vi "main_scan_2.vi"() -> ()   [LabVIEW 2009]
uses:
  <vilib>/userDefined/High Color/IMAQdx.ctl
  <vilib>/vision/Image Controls.llb/IMAQ Image.ctl
  global_stage_initialised.vi
  <vilib>/vision/driver/IMAQdx.llb/IMAQdx Buffer Number Mode.ctl
  <vilib>/Utility/file.llb/Write To Spreadsheet File (DBL).vi
  <vilib>/vision/driver/NI_Vision_Acquisition_Software.lvlib
  C:/Program Files/National Instruments/LabVIEW 2009/resource/objmgr/imaqdx.rc
panel:
  in  "Max. Spannungsdifferenz":dbl=150.0
  out "Geschätzte Messzeit":string="00:00"
  out "Start time [ms]":timestamp
  out "2D-Intensitätsverteilung (MCP)":dbl[][](graph)
  in  "# Photosignale":i32
  in  "Achs-ID":i32
  in  "Spannungskanal":refnum<k21>
  out "x-U-Scan läuft":bool
  out "Spannungsscan läuft":bool
  out "LAPD Spannung (V)":dbl format="%#.3g"
  out "Summierte Helligkeit (a.u.)":u64
  out "# Messschritte":i32
  out "Aktueller Messschritt":i32
  in  "LAPD-Daten speichern":bool
  in  "Summierte Helligkeit speichern":bool
  in  "Einzelbilder speichern":bool
  in  "Gemittelte Bilder speichern":bool
  in  "# Bilder/Messschritt":i32=1
  in  "SN von Rotationsbühne":i32=83831982
  in  "Wellenplatte [°]":refnum<k7>(container)
  out "Wellenplatte":bool
  in  "Waveplate ON/OFF":bool
  in  "Registerkarte":T1(tab)=enum."x-U-Scan"
  out "Aktuelle xyz-Position [mm]":dbl[](array[numeric]) format="%.5g"
  in  "Rasterweite [µm]":dbl[](array[numeric])
  in  "# Rasterschritte":i32[](array[numeric])=[1, 1, 1] min=1 step=1
  in  "Rasterung ON/OFF":bool
  out "Start xyz-Position [mm]":dbl[](array[numeric]) format="%.5g"
  in  "Rasterart":T2(ring)=enum."2D-Scan(xy)"
  out "Rasterschritt [µm]":dbl[](array[numeric])
  out "2D-Intensitätsverteilung (LAPD)":dbl[][](graph)
  out "Spannungsstart [V]":dbl[](array[numeric])
  out "TIP/SUP":string[](array[string])=["Tip", "Suppressor"]
  out "Spannungsschritt [V]":dbl[](array[numeric]) format="%.1g"
  out "Aktuelle Spannung [V]":dbl[](array[numeric]) format="%.1f"
  in  "# Spannungsschritte":i32[](array[numeric])
  in  "Spannungsweite [V]":dbl[](array[numeric])
  in  "Spannungsscan ON/OFF":bool
  out "Schräglage berücksichtigen":string="Schräglage berücksichtigen"
  in  "Ausgleichslage Start festlegen":bool
  out "x-U-Scan (Ausgleichslage) xy-Start [mm]":dbl[](array[numeric]) format="%_5g"
  in  "Raum-Koordinate 2 (Lagenausgleich)":enum16{"x-Achse", "y-Achse", "z-Achse"}(ring)=enum."y-Achse"
  out "x-U-Scan y-Startposition [mm]":dbl format="%.4g"
  out "x-U-Scan aktuelle y-Position [mm]":dbl format="%.4g"
  in  "x-U-Scan (Ausgleichslage) Steigung":dbl format="%_3g"
  out "x-U-Scan Spannungsstart [V]":dbl
  out "x-U-Scan Spannungsschritt [V]":dbl
  out "x-U-Scan aktuelle Spannung [V]":dbl
  in  "# x-U-Scan Spannungsschritte":i32
  in  "x-U-Scan Spannungsweite [V]":dbl
  in  "Raum-Koordinate 1":enum16{"x-Achse", "y-Achse", "z-Achse"}(ring)
  in  "Spannungs-Koordinate":enum16{"Tip-Spannung", "Suppressor-Spannung"}(ring)=2
  in  "x-U-Scan ON/OFF":bool
  in  "x-U-Scan x-Rasterweite [µm]":dbl
  in  "# x-U-Scan x-Rasterschritte":i32
  out "x-U-Scan x-Startposition [mm]":dbl format="%.4g"
  out "x-U-Scan aktuelle x-Position [mm]":dbl format="%.4g"
  out "x-U-Scan x-Rasterschritt [µm]":dbl
  out "x-U-Scan (Ausgleichslage) xy-End [mm]":dbl[](array[numeric]) format="%_5g"
  in  "Ausgleichslage Ende festlegen":bool
  in  "Sequenz Ordner":string="Referenzbilder"
  in  "Sequenzaufnahme ON":bool
  in  "MCP-Spannung [V]":dbl=1400.0
  in  "P-Schirm-Spannung [V]":dbl=4400.0
  in  "Proben-ID":string="140528_06"
  out "Messlogbuch":path
  out "Gemitteltes Bild":u64[][](array[numeric])
  in  "Polarisation [°]":dbl=90.0
  out "Current y step":i32
  out "Current z step":i32
  out "Current x step":i32
  out "Scanschleifenzähler":i32
  out "Kameraschleifenzähler":i32
  out "Steuerschleifenzähler":i32
  out "Bühne":bool
  in  "HV ON/OFF":bool
  out "HV-Steuerung":bool
  in  "Suppressor-Spannung [V]":dbl min=0.0 max=1000.0 step=1.0 format="%.1p"
  in  "Tip-Spannung [V]":dbl min=0.0 max=800.0 step=1.0 format="%.1p"
  in  "Leistung (iK) [mW]":dbl format="%.1g"
  in  "LAPD-Kanal (Meilhaus)":u32=1 max=31
  out "Save folder":string
  out "Buffer Number":u64
  out "ROI table":string[](array[string])=["Breite [px]", "Höhe [px]", "X-Offset [px]", "Y-Offset [px]"]
  in  "Vollbild":bool
  out "Frame Rate (FPS)":dbl format="%#_3g"
  in  "Buffer Interval":u32=1
  out "Ereignis: FrameDone?":refnum<event-registration>
  out "Image Display":T3(plugin-control)
  in  "ROI":i32[](array[numeric])=[640, 480, 0, 0]
  in  "Shutter time (ms)":u16(ring)=3 items=["1000", "500", "200", "100", "50", "20", "10"]
  out "Buffer Overrun":bool
  out "Image Memory":T3
  out "Kamera":bool
  in  "Kamera ON/OFF":bool
  in  "Detektionskamera":T4="cam0"
  out "Day folder":string
  in  "Root folder":string="E:\\GIPES\\Messungen\\"
  out "z-Achse":i32=3
  out "y-Achse":i32=2
  out "x-Achse":i32=1
  out "Event: Rasterung gestartet?":refnum<user-event>
  out "Fehler (Ausgang)":errorcluster
  in  "Programm beenden":bool
  out "Rasterung läuft":bool
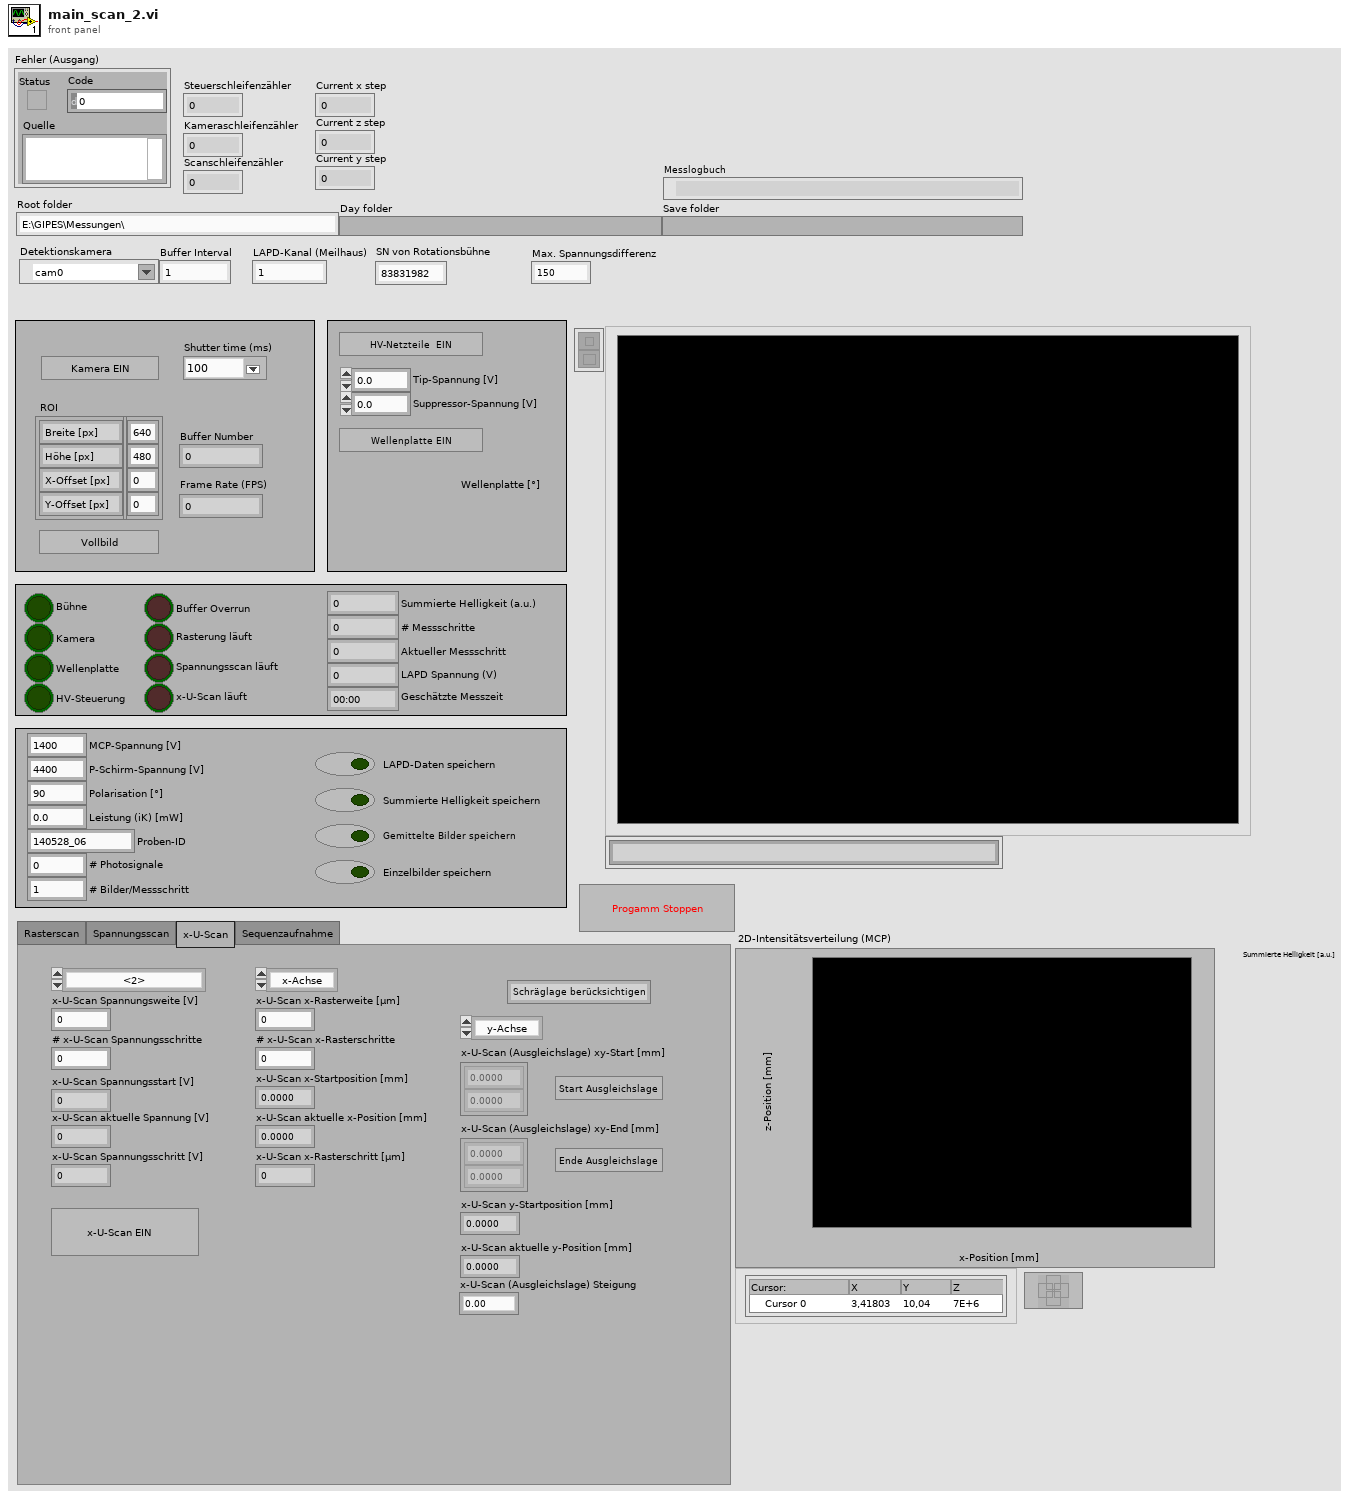
[diagram p1: front panel]
types:
  T1 = enum32{"Rasterscan", "Spannungsscan", "x-U-Scan", "Sequenzaufnahme"}
  T2 = enum16{"Linescan(x)", "Linescan(z)", "2D-Scan(xy)", "2D-Scan(yz)", "2D-Scan(xz)"}
  T3 = typedef "IMAQ Image.ctl" = refnum<image>
  T4 = typedef "IMAQdx.ctl" = refnum<k21>
  T5 = enum32{"Bad", "Idle", "Run top level", "Running"}
  T6 = typedef "NI_Vision_Acquisition_Software.lvlib/IMAQdx Buffer Number Mode.ctl" = enum32{"Next", "Last", "Buffer Number"}
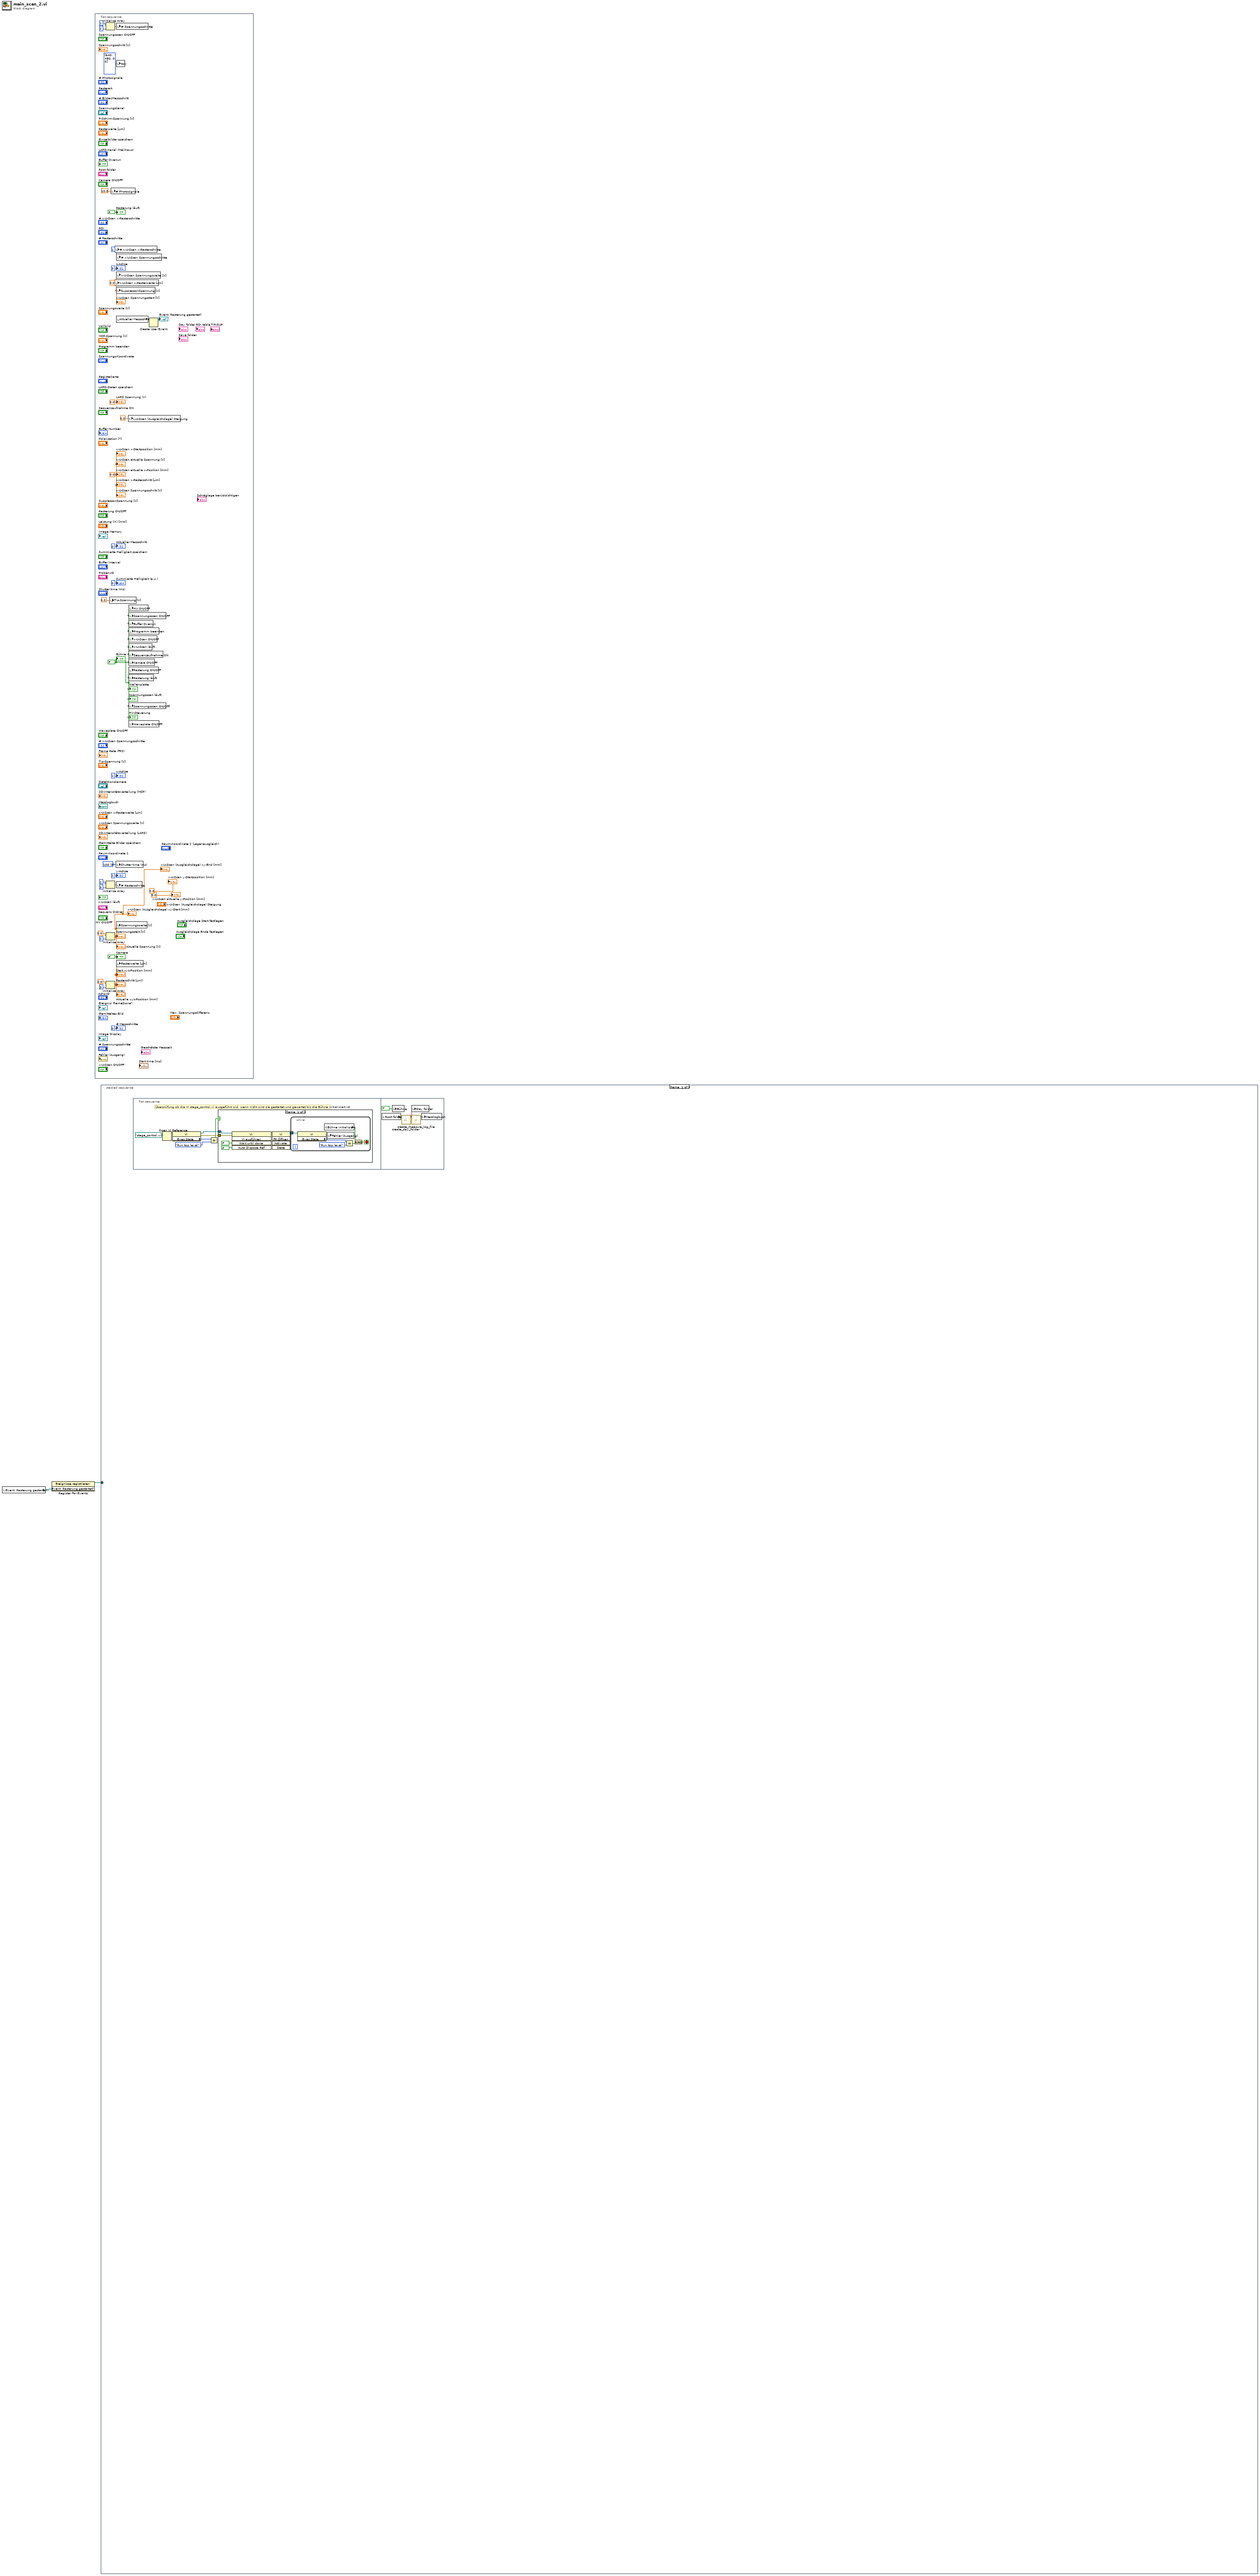
[diagram p0: block diagram]
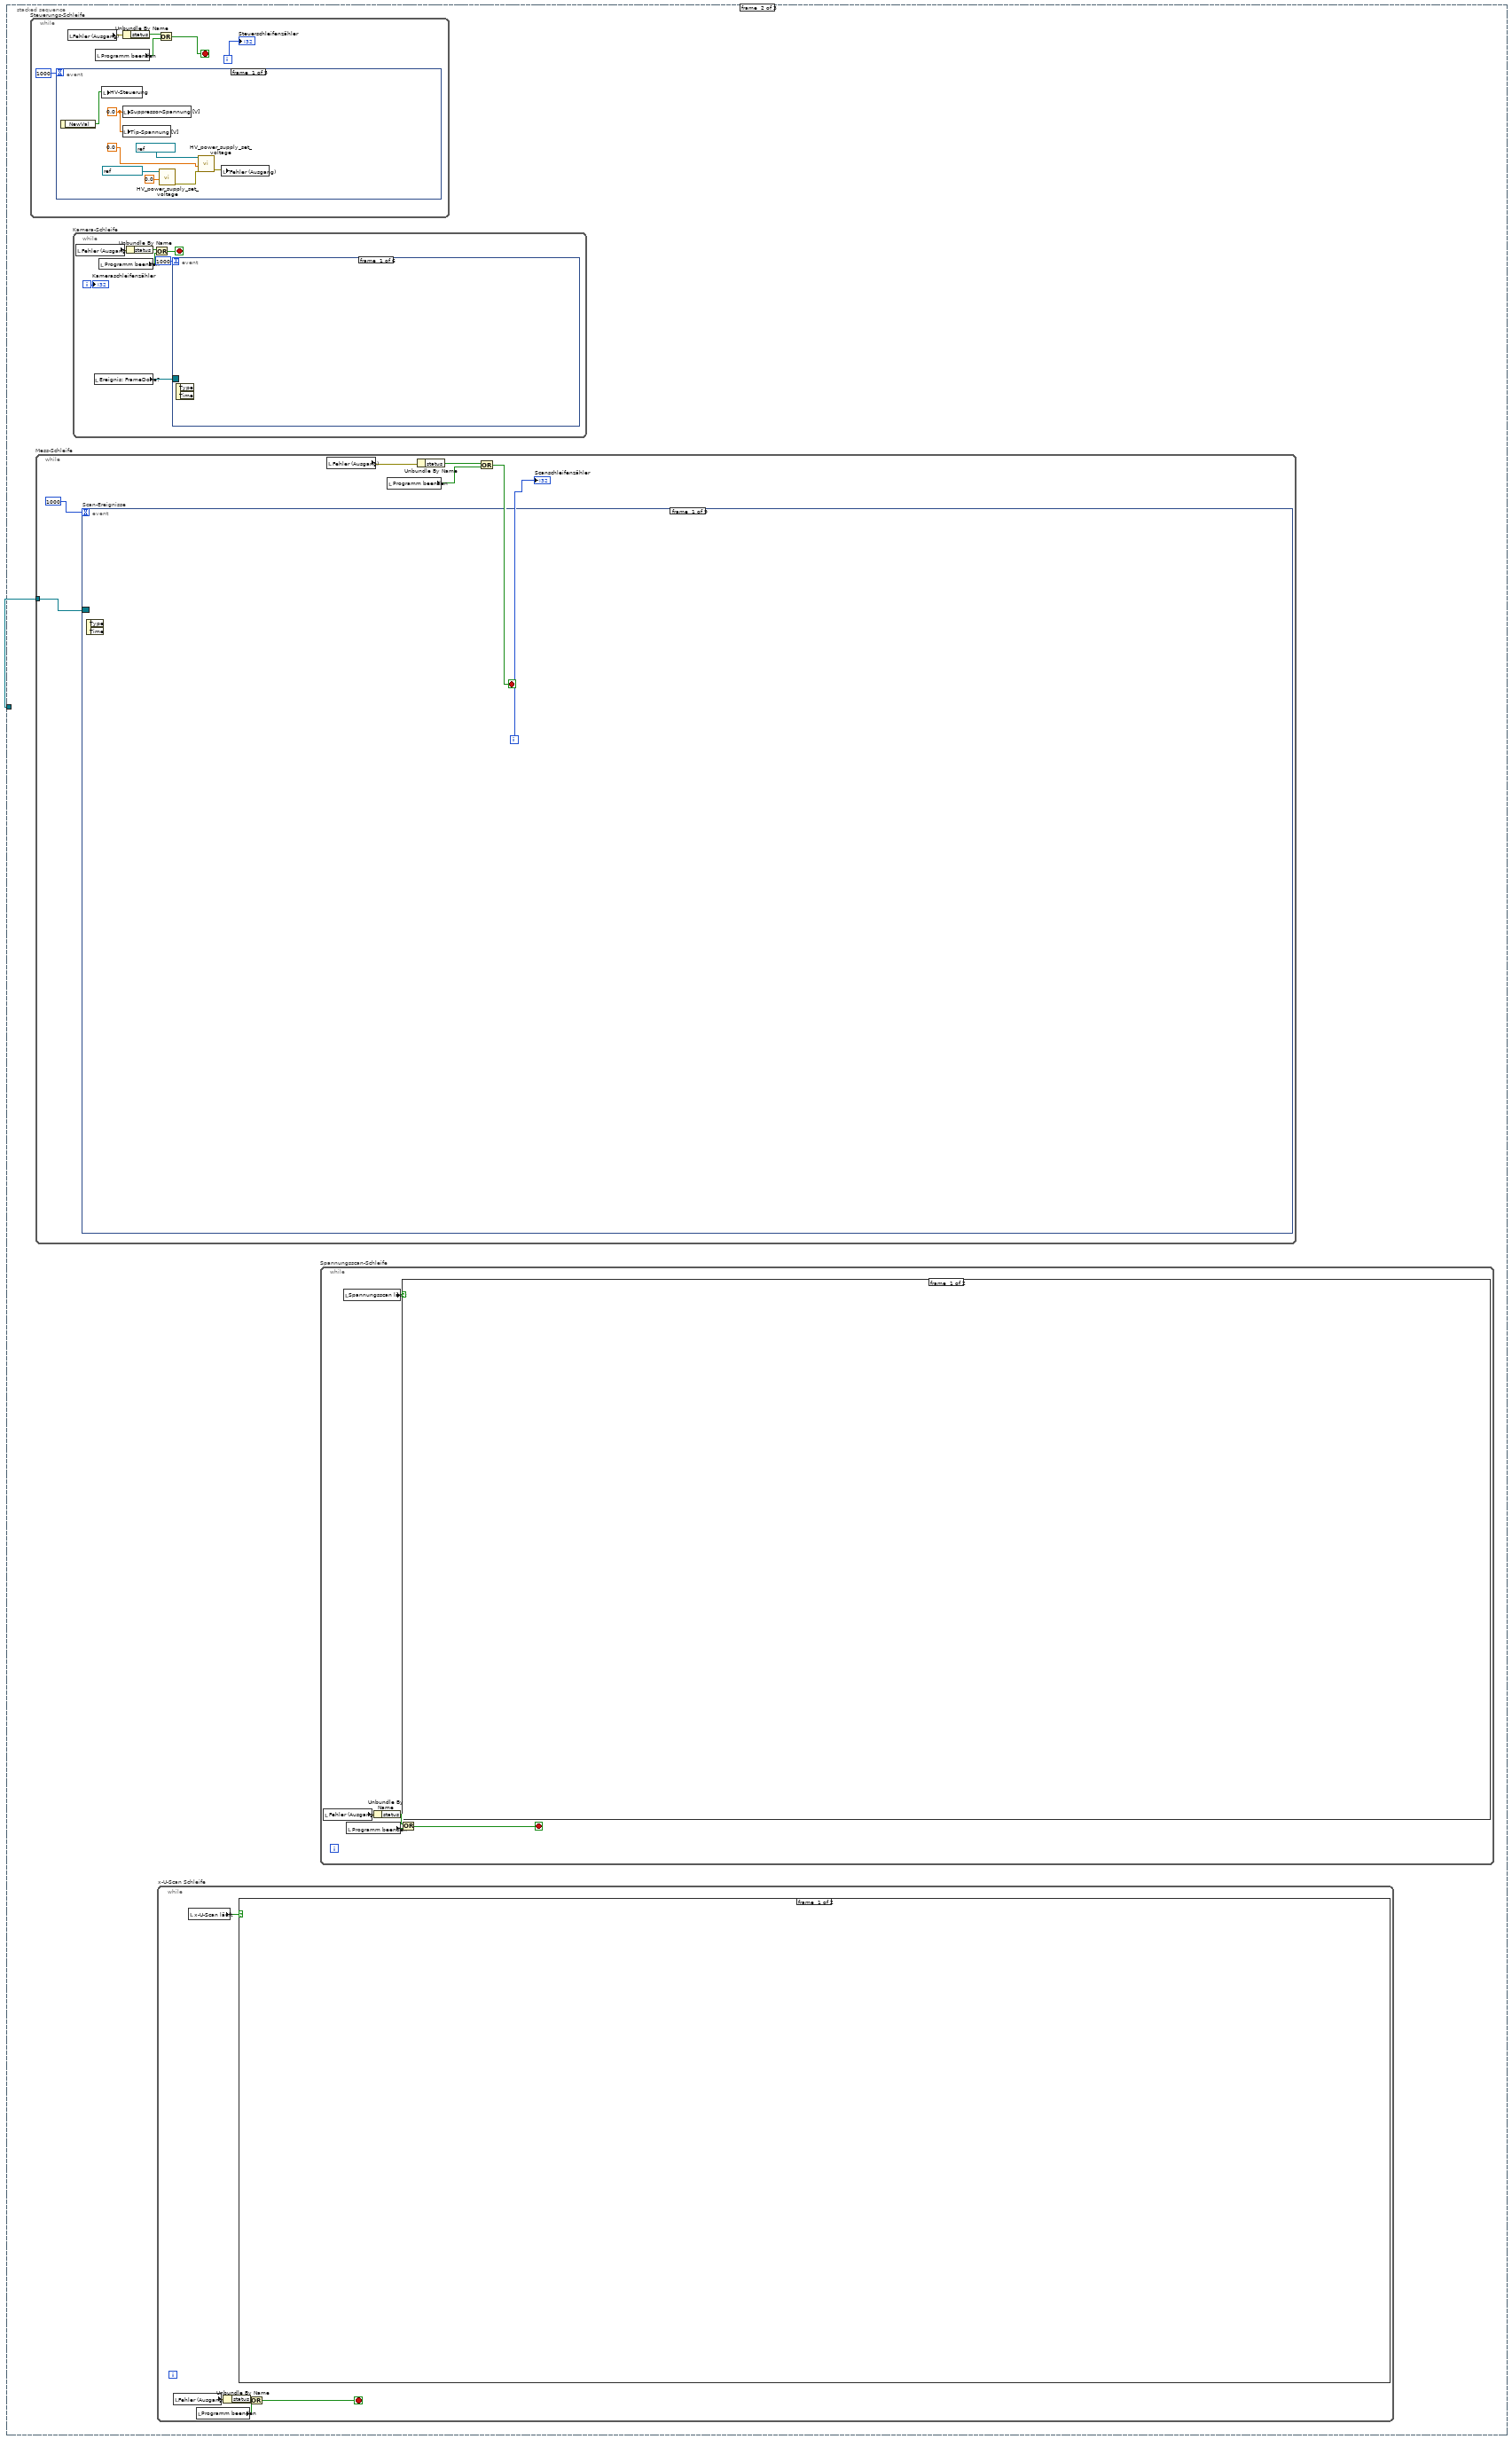
[diagram p3: hidden frame]
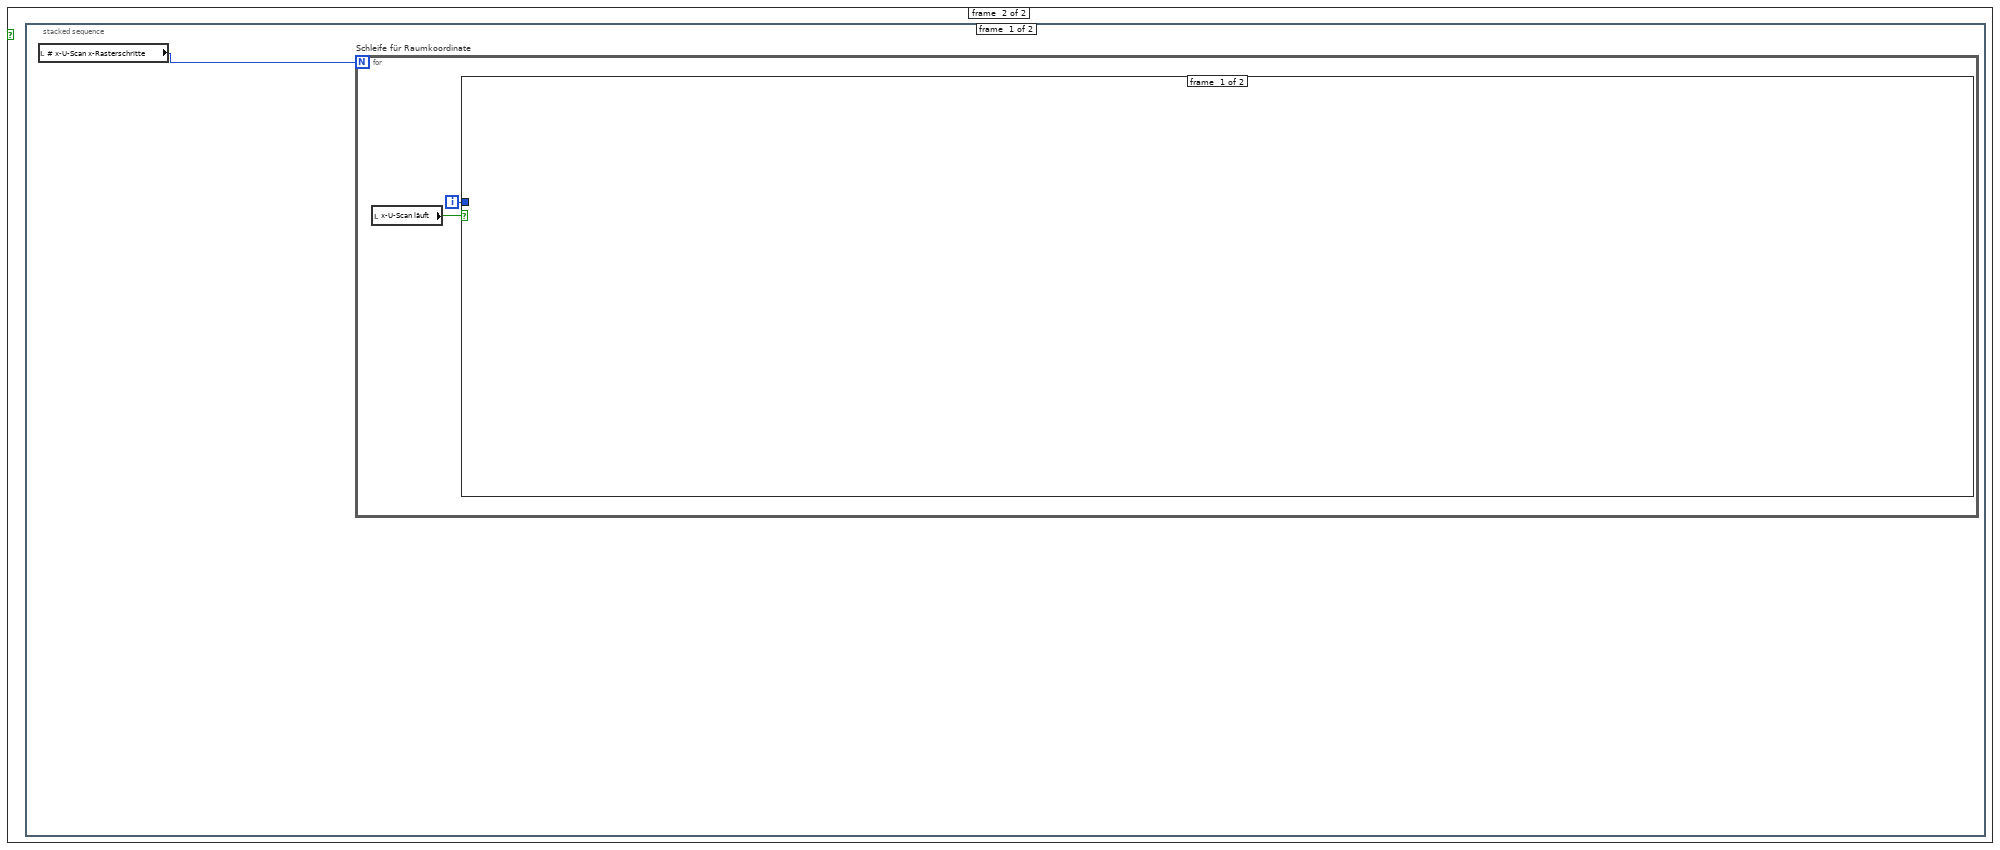
[diagram p4: hidden frame]
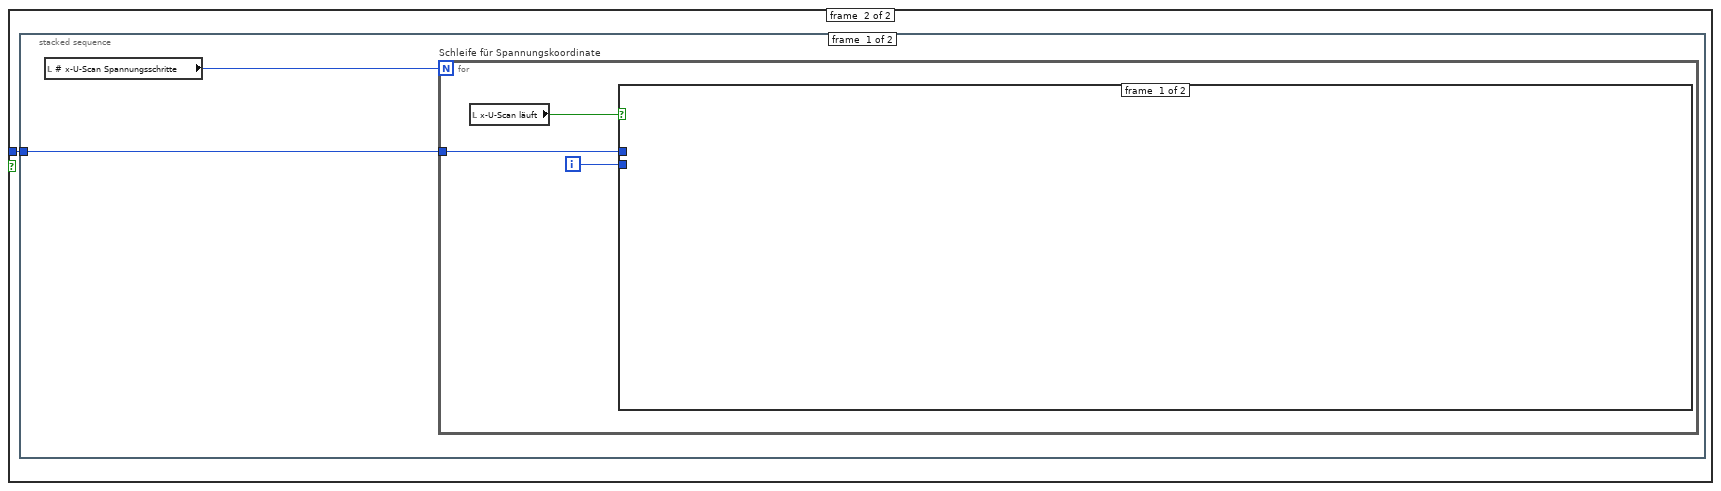
[diagram p5: hidden frame]
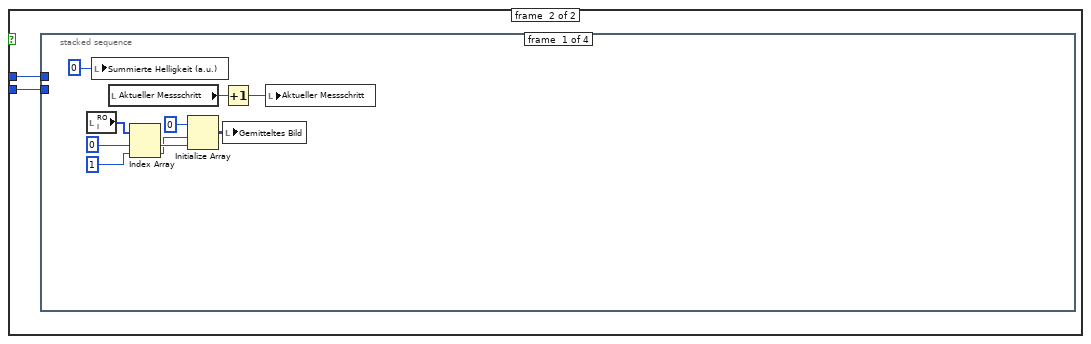
[diagram p6: hidden frame]
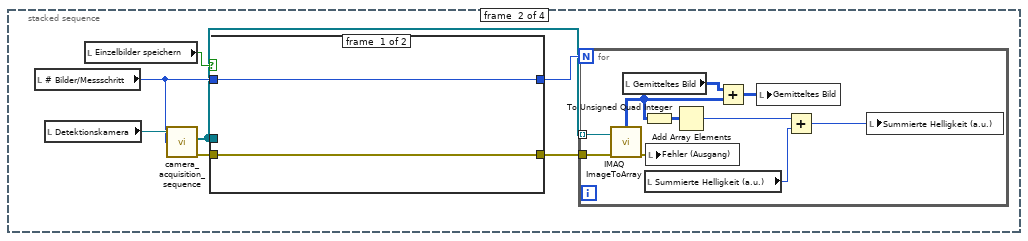
[diagram p7: hidden frame]
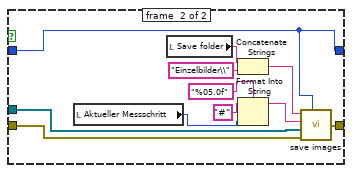
[diagram p8: hidden frame]
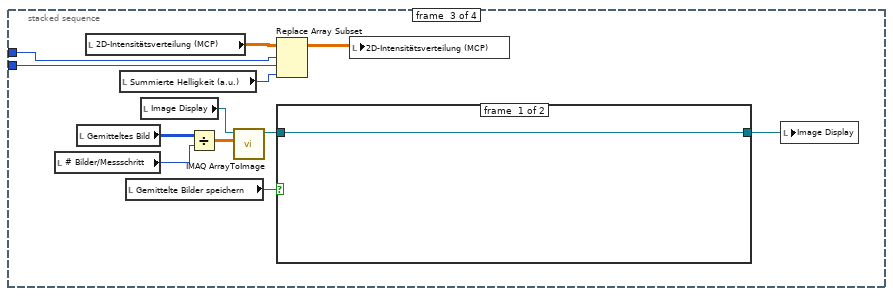
[diagram p9: hidden frame]
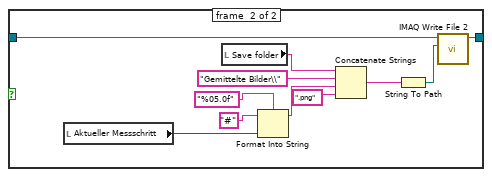
[diagram p10: hidden frame]
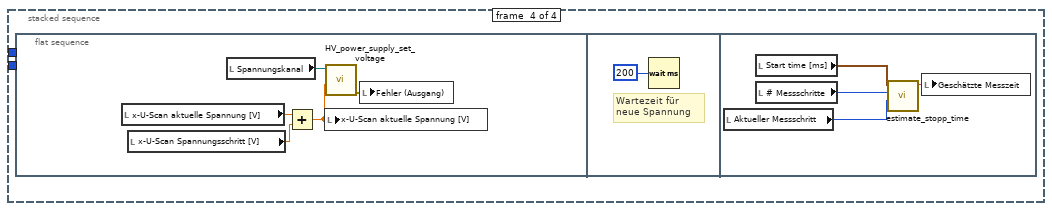
[diagram p11: hidden frame]
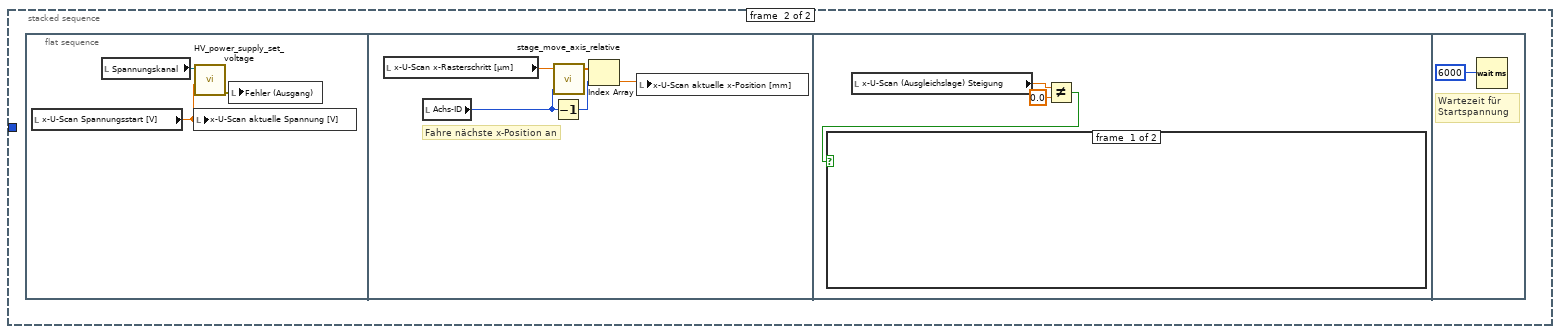
[diagram p12: hidden frame]
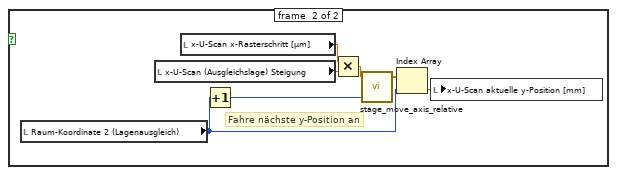
[diagram p13: hidden frame]
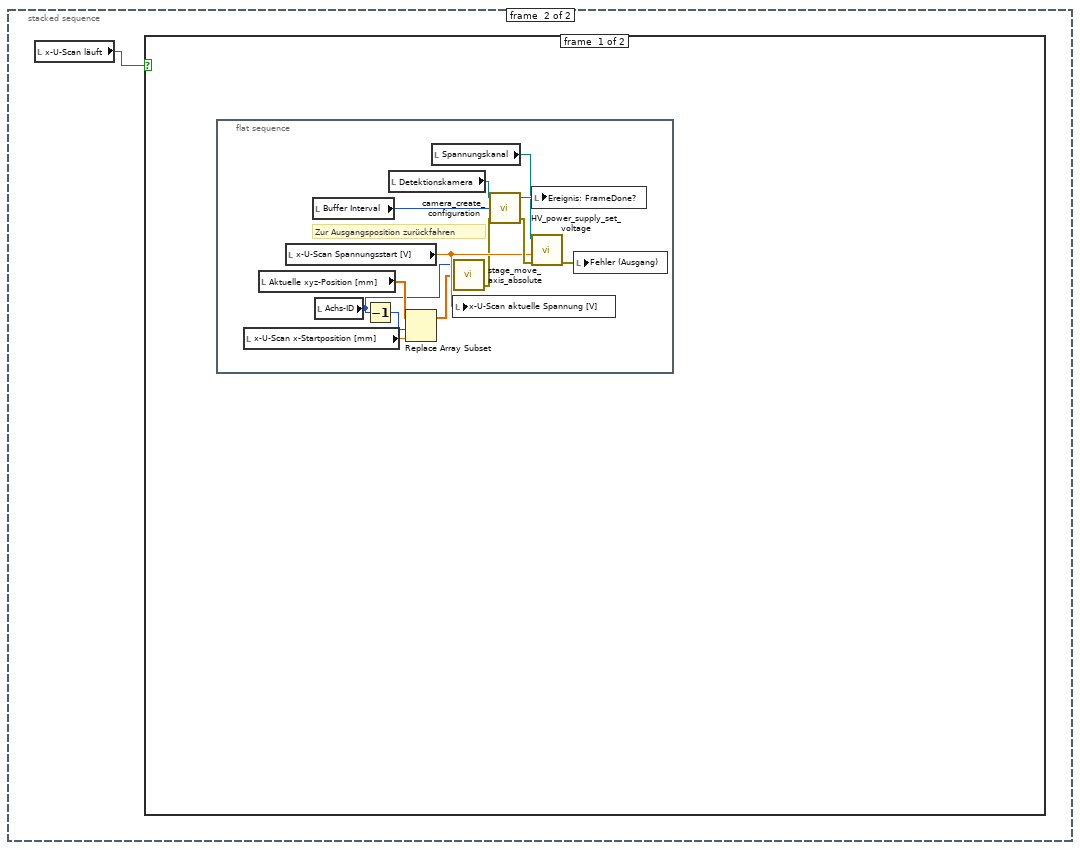
[diagram p14: hidden frame]
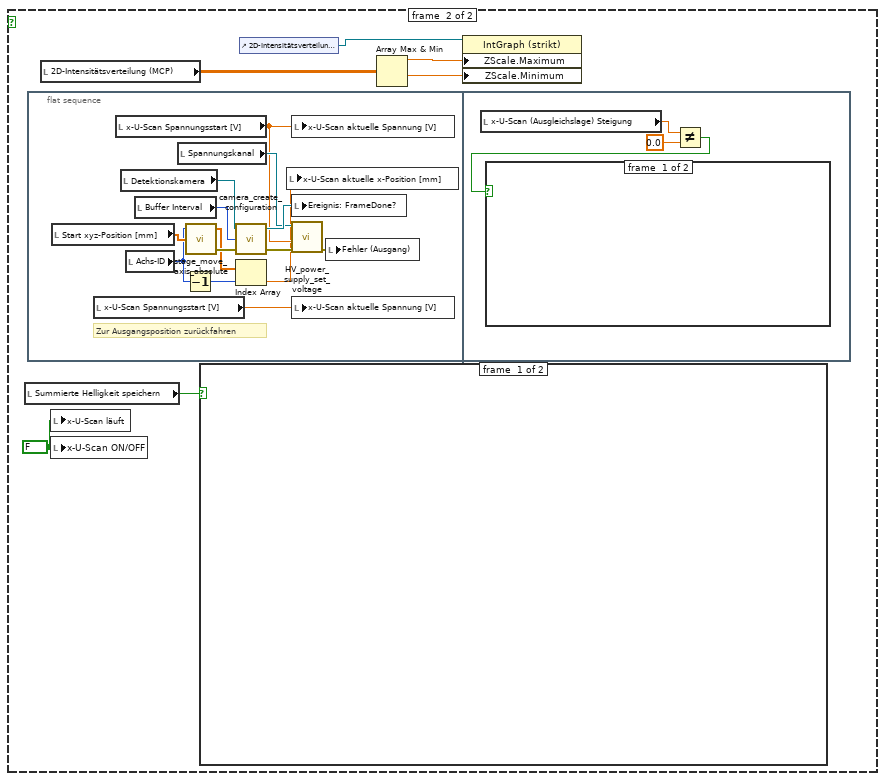
[diagram p15: hidden frame]
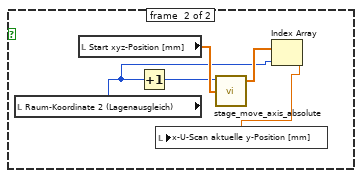
[diagram p16: hidden frame]
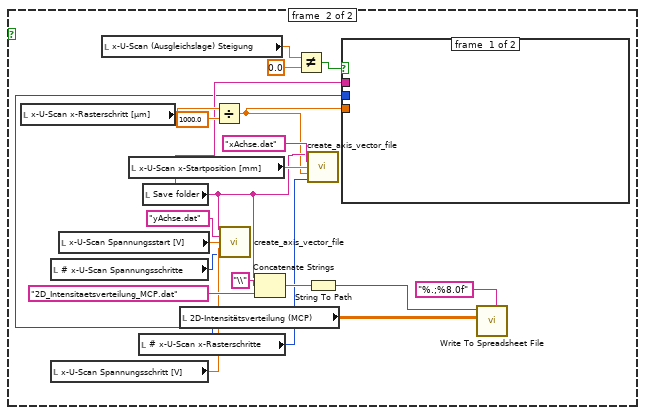
[diagram p17: hidden frame]
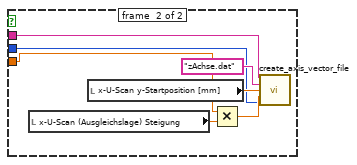
[diagram p18: hidden frame]
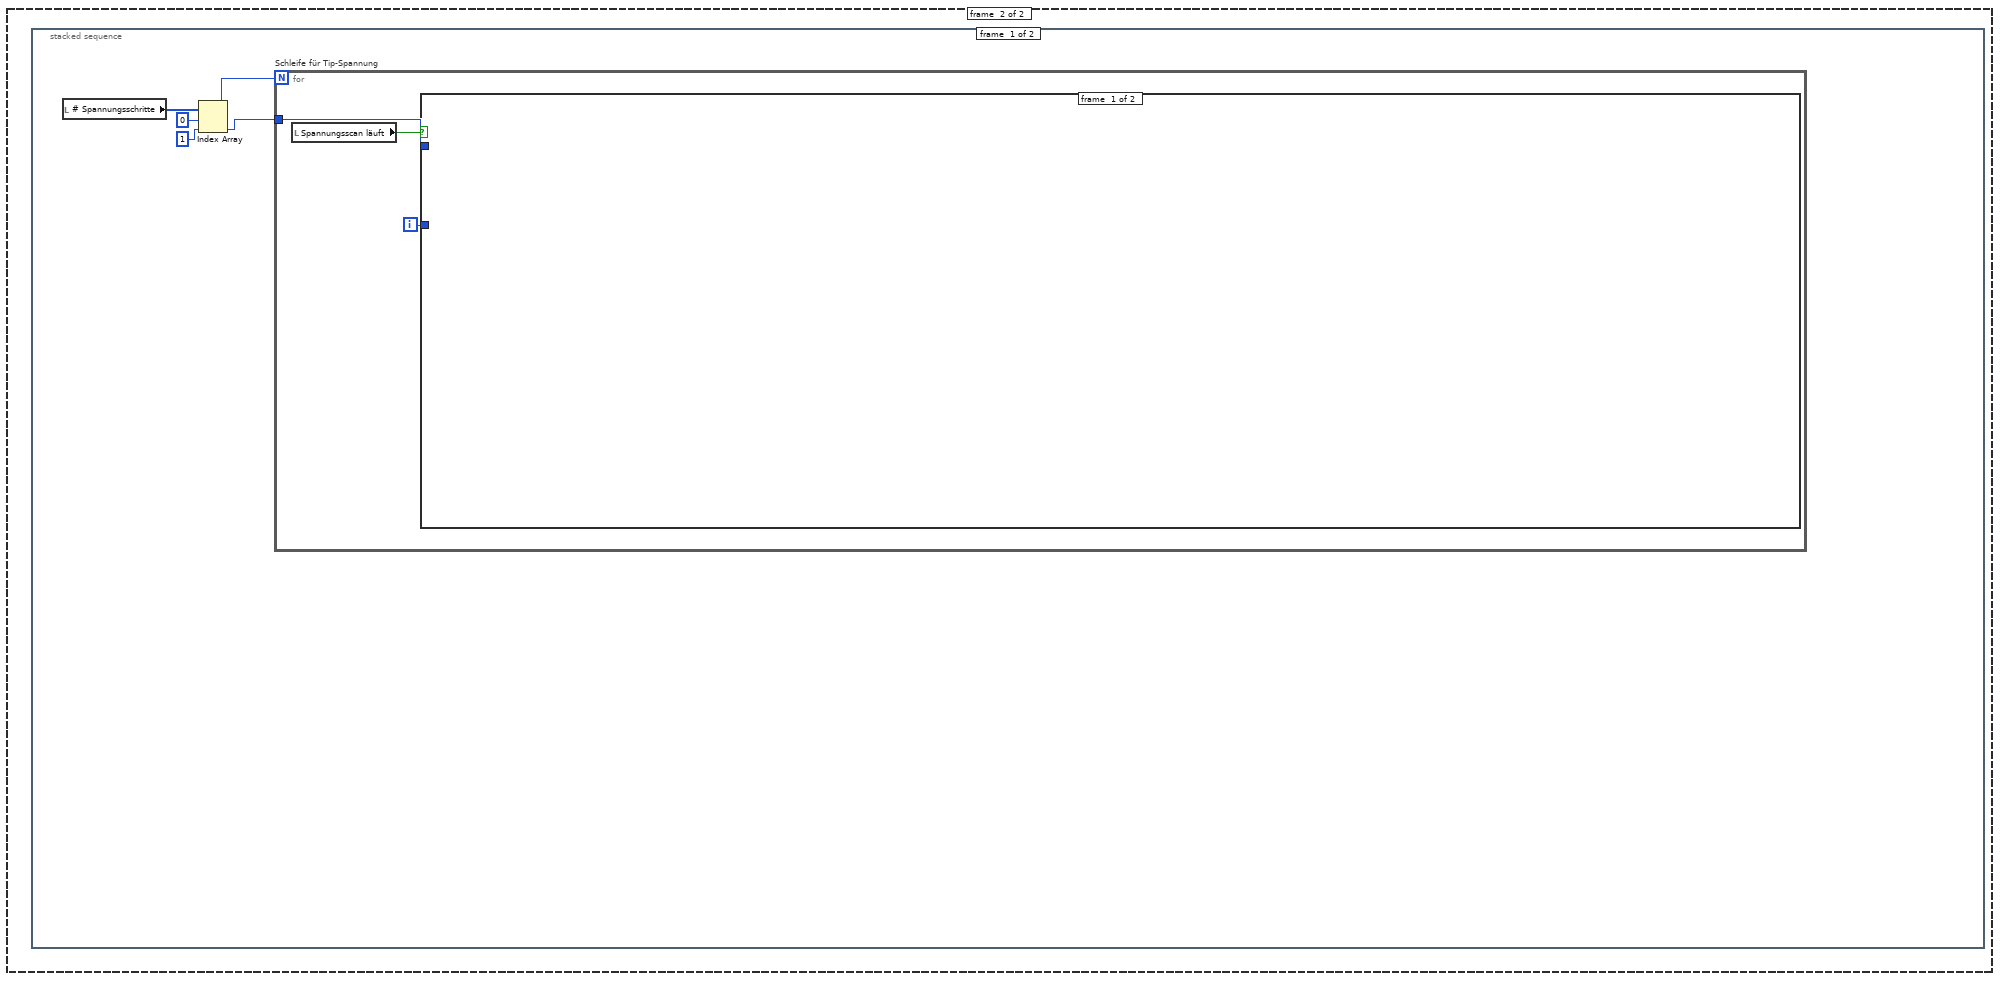
[diagram p19: hidden frame]
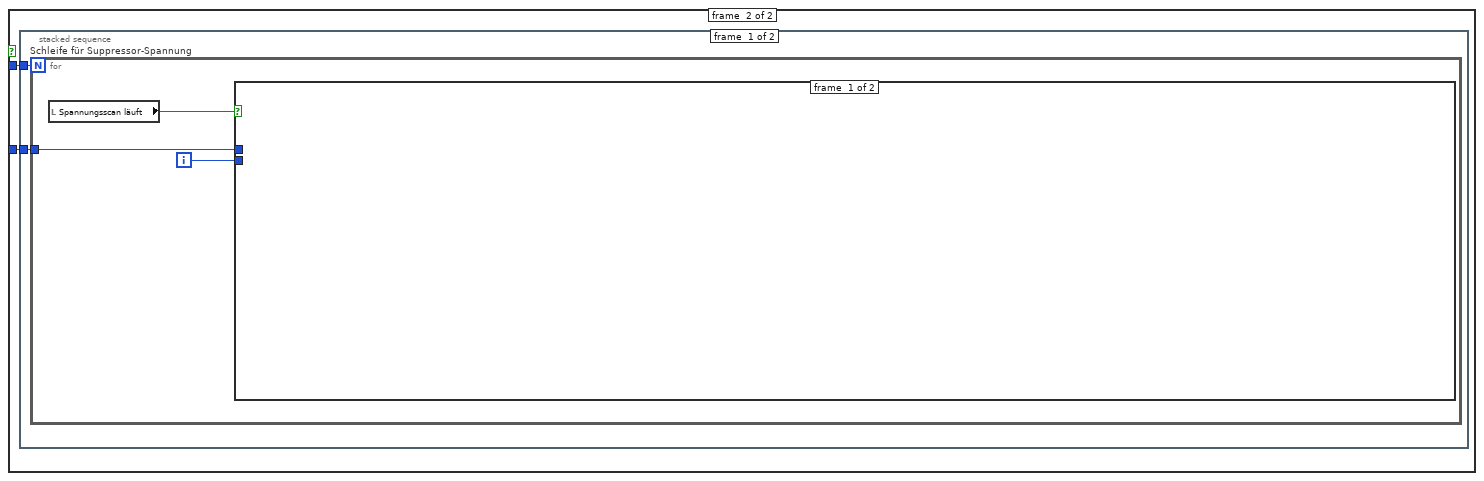
[diagram p20: hidden frame]
diagram:
  n1 = local read "Event: Rasterung gestartet?"() -> (w2:refnum<user-event>)
  n2 = register-events(w2) -> (reference out=w1:refnum<event-registration>)  [unwired: 2 in, 1 out]
  n3 = flat-sequence {
    frame #0 {
      w9 = 1 ("# x-U-Scan Spannungsschritte")
      w10 = 0.0 ("Aktuelle x-Position [mm]")
      w8 = 0.0 ("Suppressor-Spannung [V]")
      w23 = u16 3 items=["1000", "500", "200", "100", "50", "20", "10"] ("Shutter time (ms)")
      w6 = FALSE ("Scanstart")
      n4 = Initialize Array(1 ("Element"), 2 ("Dimension")) -> (w11:i32[])
      n5 = Initialize Array(1 ("Dimension"), 3 ("Dimension")) -> (w35:i32[])
      n6 = Initialize Array(0.0 ("Element"), 2 ("Dimension")) -> (w7:dbl[])
      "Aktuelle Spannung [V]" <- w7
      "Spannungsstart [V]" <- w7
      "x-U-Scan (Ausgleichslage) xy-Start [mm]" <- w7
      "x-U-Scan (Ausgleichslage) xy-End [mm]" <- w7
      n7 = Initialize Array(0.0 ("Element"), 3 ("Dimension")) -> (w17:dbl[])
      "Aktuelle xyz-Position [mm]" <- w17
      "Start xyz-Position [mm]" <- w17
      "Rasterschritt [µm]" <- w17
      n8 = local write "Tip-Spannung [V]"(0.0 ("Tip-Spannung [V]")) -> ()
      n9 = local write "# Photosignale"(10.0 ("Anzahl Mittelungen")) -> ()
      n10 = local write "# x-U-Scan x-Rasterschritte"(w9) -> ()
      n11 = local write "x-U-Scan x-Rasterweite [µm]"(w8) -> ()
      n12 = local write "Shutter time (ms)"(w23) -> ()
      n13 = local write "# Spannungsschritte"(w11) -> ()
      n14 = local write "ROI"(i32[] [640, 480, 0, 0] ("Region of Interest (px)")) -> ()
      n15 = local write "# x-U-Scan Spannungsschritte"(w9) -> ()
      n16 = local write "x-U-Scan Spannungsweite [V]"(w8) -> ()
      n17 = local write "Suppressor-Spannung [V]"(w8) -> ()
      n18 = local read "Aktueller Messschritt"() -> (w28:i32)
      n19 = local write "# Rasterschritte"(w35) -> ()
      n20 = local write "Spannungsweite [V]"(w7) -> ()
      n21 = local write "Rasterweite [µm]"(w17) -> ()
      n22 = local write "x-U-Scan (Ausgleichslage) Steigung"(0.0 ("x-U-Scan (Ausgleichslage) Steigung")) -> ()
      n23 = local write "HV ON/OFF"(w6) -> ()
      n24 = local write "Spannungsscan ON/OFF"(w6) -> ()
      n25 = local write "Buffer Overrun"(w6) -> ()
      n26 = local write "Programm beenden"(w6) -> ()
      n27 = local write "x-U-Scan ON/OFF"(w6) -> ()
      n28 = local write "x-U-Scan läuft"(w6) -> ()
      n29 = local write "Sequenzaufnahme ON"(w6) -> ()
      n30 = local write "Kamera ON/OFF"(w6) -> ()
      n31 = local write "Rasterung ON/OFF"(w6) -> ()
      n32 = local write "Rasterung läuft"(w6) -> ()
      n33 = local write "Spannungsscan ON/OFF"(w6) -> ()
      n34 = local write "Waveplate ON/OFF"(w6) -> ()
      n35 = Create User Event(user event datatype=w28) -> (user event=→"Event: Rasterung gestartet?":refnum<user-event>)  [unwired: 1 in, 1 out]
      "Rasterung läuft" <- FALSE ("Scan aktiv")
      "# Messschritte" <- 0 ("# Messschritte")
      "Aktueller Messschritt" <- 0 ("Aktueller Messschritt")
      "x-Achse" <- 1 ("x-Achse")
      "y-Achse" <- 2 ("y-Achse")
      "z-Achse" <- 3 ("z-Achse")
      "Summierte Helligkeit (a.u.)" <- i64 0 ("Numerisches Element")
      "LAPD Spannung (V)" <- 0.0 ("Transmittierte Intensität (a.u.)")
      "Bühne" <- w6
      "Wellenplatte" <- w6
      "Kamera" <- FALSE ("Camera eingeschaltet")
      "HV-Steuerung" <- w6
      "Spannungsscan läuft" <- w6
      "x-U-Scan aktuelle x-Position [mm]" <- w10
      "x-U-Scan x-Rasterschritt [µm]" <- w10
      "x-U-Scan aktuelle Spannung [V]" <- w10
      "x-U-Scan Spannungsschritt [V]" <- w10
      "x-U-Scan x-Startposition [mm]" <- w10
      "x-U-Scan Spannungsstart [V]" <- w8
      "x-U-Scan aktuelle y-Position [mm]" <- 0.0 ("x-U-Scan aktuelle y-Position [mm]")
      "x-U-Scan y-Startposition [mm]" <- 0.0 ("x-U-Scan y-Startposition [mm]")
    }
  }
  n36 = stacked-sequence {
    tunnel: w1 -> [_ w61 _]
    frame #0 {
      n37 = flat-sequence {
        frame #0 {
          # "Überprüfung ob die VI stage_control.vi ausgeführt wid, wenn nicht wird sie gestartet und gewartet bis die Bühne initialisiert ist"
          n38 = Open VI Reference(vi path=path "stage_control.vi" ("VI-Pfad")) -> (vi reference=w39:refnum<vi>)  [unwired: 5 in, 1 out]
          n39 = property class="VI"(reference=w39) -> (reference out=w38:refnum<vi>, error out=w37:errorcluster, "Exec.State"=w42:T5)  [unwired: 1 in]
          n40 = Equal?(x=w42, y=T5."Run top level") -> (x = y?=w40:bool)
          n41 = case shown="False" w40 {
            tunnel: w38 -> [w49 _]
            tunnel: w37 -> [w48 _]
            frame #0 {
              n42 = invoke class="VI" method="VI ausführen"(reference=w49, error in=w48, "Wait until done"=FALSE ("Warten bis beendet"), "Auto Dispose Ref"=FALSE ("Referenz automatisch schließen")) -> (reference out=w45:refnum<vi>)  [unwired: 1 in, 4 out]
              n43 = invoke class="VI" method="FP.Öffnen"(reference=w45) -> (reference out=w44:refnum<vi>)  [unwired: 4 in, 4 out]
              n44 = while {
                tunnel: w44 -> [w56]
                stop <- w51 stop-if-true
                n45 = property class="VI"(reference=w56) -> (error out=w55:errorcluster, "Exec.State"=w54:T5)  [unwired: 1 in, 1 out]
                n46 = global read "global_stage_initialised.vi" "Bühne initialisiert"() -> (w50:bool)
                n47 = local write "Fehler (Ausgang)"(w55) -> ()
                n48 = Equal?(x=w54, y=T5."Run top level") -> (x = y?=w52:bool)
                n49 = And(x=w50, y=w52) -> (x .and. y?=w51:bool)
              }
            }
            frame #1 {
            }
          }
        }
        frame #1 {
          n50 = local read "Root folder"() -> (w60:string)
          n51 = local write "Bühne"(TRUE ("Bühne bereit")) -> ()
          n52 = call "create_day_folder.vi"("Root folder"=w60) -> ("Day Folder"=w58:string)  [unwired: 9 in, 1 out]
          n53 = local write "Day folder"(w58) -> ()
          n54 = call "create_measure_log_file.vi"("Tagesordner"=w58) -> ("Messlogbuch"=w57:path)  [unwired: 9 in]
          n55 = local write "Messlogbuch"(w57) -> ()
        }
      }
    }
    frame #1 {
      n56 = while "Steuerungs-Schleife" {
        i -> [w418]
        stop <- w417 stop-if-true
        n57 = event shown="[2] \"Tip-Spannung [V]\": Wertänderung" {
          selector: _ -> [_ _ _ _ _]
          dyn-events: _ -> [_ _ _ _ _]
          timeout: 1000 -> [_ _ _ _ _]
          event #0 {
            w423 = 0.0 ("Suppressor-Spannung [V]")
            n58 = event-data() -> ("NewVal"=w424:bool)  [unwired: 1 in]
            n59 = local write "HV-Steuerung"(w424) -> ()
            n60 = local write "Suppressor-Spannung [V]"(w423) -> ()
            n61 = local write "Tip-Spannung [V]"(w423) -> ()
            n62 = call "HV_power_supply_set_voltage.vi"("Desired output voltage in V (HV power supply)"=0.0, "Channel of HV power supply"=refnum<k21> "Dev0/Ao0") -> ("error out"=w426:errorcluster)  [unwired: 8 in]
            n63 = call "HV_power_supply_set_voltage.vi"("error in"=w426, "Desired output voltage in V (HV power supply)"=0.0, "Channel of HV power supply"=refnum<k21> "Dev0/Ao1") -> ("error out"=w425:errorcluster)  [unwired: 7 in]
            n64 = local write "Fehler (Ausgang)"(w425) -> ()
          }
          event #1 {
            n65 = event-data() -> ("NewVal"=w431:bool)  [unwired: 1 in]
            n66 = case shown="True" w431 {
              frame #0 {
                n67 = local read "Wellenplatte [°]"() -> (w434:refnum<k7>)
                n68 = invoke class="MG17Motor" method="StopCtrl"(reference=w434) -> (error out=w433:errorcluster)  [unwired: 2 in, 2 out]
                n69 = Unbundle By Name(w433) -> ("status"=w432:bool)
                n70 = local write "Wellenplatte"(w432) -> ()
              }
              frame #1 {
                n71 = property class="MG17Motor"(reference="Wellenplatte [°]", "HWSerialNum"="SN von Rotationsbühne") -> (reference out=w441:refnum<k7>, error out=w440:errorcluster)  [unwired: 1 in]
                n72 = invoke class="MG17Motor" method="StartCtrl"(reference=w441, error in=w440) -> (error out=w439:errorcluster)  [unwired: 1 in, 2 out]
                n73 = local write "Fehler (Ausgang)"(w439) -> ()
                n74 = Unbundle By Name(w439) -> ("status"=w438:bool)
                n75 = Not(x=w438) -> (.not. x?=w437:bool)
                n76 = local write "Wellenplatte"(w437) -> ()
              }
            }
          }
          event #2 {
            n77 = event-data() -> ("OldVal"=w442:dbl, "NewVal"=w448:dbl)  [unwired: 1 in]
            n78 = local read "Suppressor-Spannung [V]"() -> (w447:dbl)
            n79 = local read "Max. Spannungsdifferenz"() -> (w445:dbl)
            n80 = local read "HV-Steuerung"() -> (w443:bool)
            n81 = Subtract(x=w448, y=w447) -> (x-y=w446:dbl)
            n82 = Less Or Equal?(x=w446, y=w445) -> (x <= y?=w444:bool)
            n83 = case shown="True" w443 {
              tunnel: w444 -> [_ w450]
              tunnel: w442 -> [_ w449]
              frame #0 {
              }
              frame #1 {
                n84 = case shown="True" w450 {
                  tunnel: w449 -> [w451 _]
                  frame #0 {
                    n85 = local write "Tip-Spannung [V]"(w451) -> ()
                  }
                  frame #1 {
                    n86 = local read "Tip-Spannung [V]"() -> (w452:dbl)
                    n87 = call "HV_power_supply_set_voltage.vi"("Desired output voltage in V (HV power supply)"=w452, "Channel of HV power supply"=refnum<k21> "Dev0/Ao1") -> ("error out"=w453:errorcluster)  [unwired: 8 in]
                    n88 = local write "Fehler (Ausgang)"(w453) -> ()
                  }
                }
              }
            }
          }
          event #3 {
            n89 = event-data() -> ("OldVal"=w455:dbl, "NewVal"=w457:dbl)  [unwired: 1 in]
            n90 = local read "Max. Spannungsdifferenz"() -> (w458:dbl)
            n91 = local read "Tip-Spannung [V]"() -> (w456:dbl)
            n92 = local read "HV-Steuerung"() -> (w461:bool)
            n93 = Subtract(x=w456, y=w457) -> (x-y=w460:dbl)
            n94 = Less Or Equal?(x=w460, y=w458) -> (x <= y?=w459:bool)
            n95 = case shown="True" w461 {
              tunnel: w459 -> [_ w463]
              tunnel: w455 -> [_ w462]
              frame #0 {
              }
              frame #1 {
                n96 = case shown="True" w463 {
                  tunnel: w462 -> [w464 _]
                  frame #0 {
                    n97 = local write "Suppressor-Spannung [V]"(w464) -> ()
                  }
                  frame #1 {
                    n98 = local read "Suppressor-Spannung [V]"() -> (w465:dbl)
                    n99 = call "HV_power_supply_set_voltage.vi"("Desired output voltage in V (HV power supply)"=w465, "Channel of HV power supply"=refnum<k21> "Dev0/Ao0") -> ("error out"=w466:errorcluster)  [unwired: 8 in]
                    n100 = local write "Fehler (Ausgang)"(w466) -> ()
                  }
                }
              }
            }
          }
          event #4 {
            n101 = event-data() -> ()  [unwired: 1 in, 2 out]
          }
        }
        n102 = local read "Fehler (Ausgang)"() -> (w422:errorcluster)
        n103 = local read "Programm beenden"() -> (w421:bool)
        n104 = Unbundle By Name(w422) -> ("status"=w420:bool)
        n105 = Or(x=w420, y=w421) -> (x .or. y?=w417:bool)
        "Steuerschleifenzähler" <- w418
      }
      n106 = while "Mess-Schleife" {
        tunnel: w61 -> [w470]
        i -> [w469]
        stop <- w468 stop-if-true
        n107 = event "Scan-Ereignisse" shown="[3] <Event: Rasterung gestartet?>: Benutzerereignis" {
          selector: w470 -> [_ _ _ _ _ _ _ _ _]
          dyn-events: _ -> [_ _ _ _ _ _ _ _ _]
          timeout: 1000 -> [_ _ _ _ _ _ _ _ _]
          event #0 {
            n108 = event-data() -> ()  [unwired: 1 in, 2 out]
          }
          event #1 {
            n109 = event-data() -> ("NewVal"=w477:bool)  [unwired: 1 in]
            n110 = local read "Kamera"() -> (w476:bool)
            n111 = And(x=w476, y=w477) -> (x .and. y?=w475:bool)
            n112 = case shown="True" w475 {
              frame #0 {
                n113 = local write "Rasterung läuft"(FALSE ("Rasterung läuft")) -> ()
              }
              frame #1 {
                n114 = stacked-sequence {
                  frame #0 {
                    n115 = flat-sequence {
                      tunnel: [w489] -> w479
                      tunnel: w479 -> [w552]
                      frame #0 {
                        n116 = local read "# Bilder/Messschritt"() -> (w495:i32)
                        n117 = local read "Rasterweite [µm]"() -> (w500:dbl[])
                        n118 = local read "# Rasterschritte"() -> (w502:i32[])
                        n119 = control-ref of="Rasterart"() -> (w498:refnum<vi>)
                        n120 = local read "ROI"() -> (w483:i32[])
                        n121 = property class="Enum (strikt)"(reference=w498) -> ("RingText.Text"=w484:string)  [unwired: 1 in, 2 out]
                        n122 = local read "Rasterart"() -> (w503:T2)
                        n123 = control-ref of="Shutter time (ms)"() -> (w497:refnum<vi>)
                        n124 = call "stage_get_current_xyz.vi"() -> ("Aktuelle xyz-Position OUT [mm]"=w488:dbl[])  [unwired: 3 in, 1 out]
                        n125 = case shown="\"2D-Scan(xz)\"" w503 {
                          tunnel: w502 -> [w511 w527 w532 w541 w547]
                          tunnel: [w510 w526 w533 w540 w544] -> w501
                          tunnel: w500 -> [w509 w517 w529 w537 w546]
                          tunnel: [w508 w516 w528 w536 w545] -> w499
                          frame #0 {
                            n126 = Replace Array Subset(array=w509, new element #1=0.0 ("Neues Element/Teil-Array"), index #1=1 ("Index"), new element #2=0.0 ("Neues Element/Teil-Array"), index #2=2 ("Index")) -> (w508:dbl[])
                            n127 = Replace Array Subset(array=w511, new element #1=1 ("Neues Element/Teil-Array"), index #1=1 ("Index"), new element #2=1 ("Neues Element/Teil-Array"), index #2=2 ("Index")) -> (w510:i32[])
                          }
                          frame #1 {
                            n128 = Replace Array Subset(array=w517, new element #1=0.0 ("Neues Element/Teil-Array"), index #1=0 ("Index"), new element #2=0.0 ("Neues Element/Teil-Array"), index #2=1 ("Index")) -> (w516:dbl[])
                            n129 = Replace Array Subset(array=w527, new element #1=1 ("Neues Element/Teil-Array"), index #1=0 ("Index"), new element #2=1 ("Neues Element/Teil-Array"), index #2=1 ("Index")) -> (w526:i32[])
                          }
                          frame #2 {
                            n130 = Replace Array Subset(array=w529, new element=0.0 ("Neues Element/Teil-Array"), index=2 ("Index")) -> (w528:dbl[])
                            n131 = Replace Array Subset(array=w532, new element=1 ("Neues Element/Teil-Array"), index=2 ("Index")) -> (w533:i32[])
                          }
                          frame #3 {
                            n132 = Replace Array Subset(array=w537, new element=0.0 ("Neues Element/Teil-Array"), index=0 ("Index")) -> (w536:dbl[])
                            n133 = Replace Array Subset(array=w541, new element=1 ("Neues Element/Teil-Array"), index=0 ("Index")) -> (w540:i32[])
                          }
                          frame #4 {
                            n134 = Replace Array Subset(array=w546, new element=0.0 ("Neues Element/Teil-Array"), index=1 ("Index")) -> (w545:dbl[])
                            n135 = Replace Array Subset(array=w547, new element=1 ("Neues Element/Teil-Array"), index=1 ("Index")) -> (w544:i32[])
                          }
                        }
                        n136 = property class="Ring (strikt)"(reference=w497) -> ("RingText.Text"=w496:string)  [unwired: 1 in, 2 out]
                        n137 = Decimal String To Number(string=w496) -> (number=w493:i32)  [unwired: 2 in, 1 out]
                        n138 = local read "P-Schirm-Spannung [V]"() -> (w487:dbl)
                        n139 = local read "Suppressor-Spannung [V]"() -> (w482:dbl)
                        n140 = local read "MCP-Spannung [V]"() -> (w486:dbl)
                        n141 = local read "Leistung (iK) [mW]"() -> (w485:dbl)
                        n142 = local read "Polarisation [°]"() -> (w490:dbl)
                        n143 = local read "Tip-Spannung [V]"() -> (w481:dbl)
                        n144 = local read "Messlogbuch"() -> (w492:path)
                        n145 = local read "Proben-ID"() -> (w491:string)
                        n146 = Get Date/Time In Seconds() -> (seconds since 1Jan1904=w480:timestamp)
                        n147 = Multiply(x=w495, y=w493) -> (x*y=w494:i32)
                        n148 = local write "Start time [ms]"(w480) -> ()
                        n149 = local write "Rasterweite [µm]"(w499) -> ()
                        n150 = local write "# Rasterschritte"(w501) -> ()
                        n151 = call "create_measure_log_entry.vi"("Messlogbuch-Pfad"=w492, "Probe"=w491, "Polarisation [°]"=w490, "Messart"=w484, "ROI"=w483, "Messungen/Messschritt"=w495, "Maximalleistung (iK) [mW]"=w485, "Tip-Spannung [V]"=w481, "Suppressor-Spannung [V]"=w482, "Zeit/Messschritt [ms]"=w493, "MCP-Spannung [V]"=w486, "Zeit/Messung [ms]"=w494, "Phosphorschirm-Spannung [V]"=w487, "xyz [mm]"=w488) -> ("Messung Nr."=w489:i32)  [unwired: 4 in, 1 out]
                      }
                      frame #1 {
                        n152 = local read "Day folder"() -> (w558:string)
                        n153 = local read "Fehler (Ausgang)"() -> (w553:errorcluster)
                        n154 = local write "Aktueller Messschritt"(0 ("Aktueller Messschritt")) -> ()
                        n155 = local read "Rasterweite [µm]"() -> (w578:dbl[])
                        n156 = local read "# Rasterschritte"() -> (w577:i32[])
                        n157 = local read "# Rasterschritte"() -> (w575:i32[])
                        n158 = local read "Einzelbilder speichern"() -> (w561:bool)
                        n159 = call "create_save_folder.vi"("Day folder"=w558, "Measuring number"=w552, "Measuring folder"="Rasterung" ("Subfolder"), "error in"=w553) -> ("Save Folder"=w557:string, "Error Out"=w556:errorcluster)  [unwired: 5 in]
                        n160 = local write "Save folder"(w557) -> ()
                        n161 = Divide(x=w578, y=w577) -> (x/y=w576:dbl[])
                        n162 = Index Array(array=w575, index #1=0 ("Index"), index #2=1 ("Index"), index #3=2 ("Index")) -> (element #1=w572:i32, element #2=w571:i32, element #3=w570:i32)
                        n163 = Multiply(x=w572, y=w571) -> (x*y=w569:i32)
                        n164 = local write "Rasterschritt [µm]"(w576) -> ()
                        n165 = local read "Kamera"() -> (w564:bool)
                        n166 = local read "Gemittelte Bilder speichern"() -> (w562:bool)
                        n167 = case shown="True" w561 {
                          tunnel: w556 -> [w579 w581]
                          tunnel: [w579 w580] -> w555
                          frame #0 {
                          }
                          frame #1 {
                            n168 = local read "Save folder"() -> (w584:string)
                            n169 = Concatenate Strings(w584, "\\Einzelbilder" ("Subfolder")) -> (w582:string)
                            n170 = String To Path(string=w582) -> (path=w585:path)
                            n171 = call <vilib>:"Check if File or Folder Exists.vi"("error in (no error)"=w581, "path"=w585) -> ("error out"=w580:errorcluster, "file or folder exists?"=w586:bool, "dup path"=w587:path)  [unwired: 7 in]
                            n172 = case shown="False" w586 {
                              tunnel: w587 -> [w588 _]
                              frame #0 {
                                n173 = Create Folder(path (use dialog)=w588) -> ()  [unwired: 2 in, 3 out]
                              }
                              frame #1 {
                              }
                            }
                          }
                        }
                        n174 = Multiply(x=w569, y=w570) -> (x*y=w568:i32)
                        n175 = local write "# Messschritte"(w568) -> ()
                        n176 = case shown="True" w562 {
                          tunnel: w555 -> [w589 w591]
                          tunnel: [w589 w590] -> w554
                          frame #0 {
                          }
                          frame #1 {
                            n177 = local read "Save folder"() -> (w595:string)
                            n178 = Concatenate Strings(w595, "\\Gemittelte Bilder" ("Subfolder")) -> (w597:string)
                            n179 = String To Path(string=w597) -> (path=w594:path)
                            n180 = call <vilib>:"Check if File or Folder Exists.vi"("error in (no error)"=w591, "path"=w594) -> ("error out"=w590:errorcluster, "file or folder exists?"=w593:bool, "dup path"=w592:path)  [unwired: 7 in]
                            n181 = case shown="False" w593 {
                              tunnel: w592 -> [w598 _]
                              frame #0 {
                                n182 = Create Folder(path (use dialog)=w598) -> ()  [unwired: 2 in, 3 out]
                              }
                              frame #1 {
                              }
                            }
                          }
                        }
                        n183 = case shown="True" w564 {
                          tunnel: [w599 w601] -> w563
                          tunnel: w554 -> [w599 w600]
                          frame #0 {
                          }
                          frame #1 {
                            n184 = local read "Ereignis: FrameDone?"() -> (w602:refnum<event-registration>)
                            n185 = local read "Detektionskamera"() -> (w603:T4)
                            n186 = call "camera_release_configuration.vi"("error in"=w600, "Session In"=w603, "Ereignisregistrierung (Referenz) 2"=w602) -> ("error out"=w601:errorcluster)  [unwired: 1 out]
                          }
                        }
                        n187 = call "stage_get_current_xyz.vi"("error in"=w563) -> ("error out"=w560:errorcluster, "Aktuelle xyz-Position OUT [mm]"=w565:dbl[])  [unwired: 2 in]
                        n188 = local write "Start xyz-Position [mm]"(w565) -> ()
                        n189 = local write "Fehler (Ausgang)"(w560) -> ()
                      }
                    }
                  }
                  frame #1 {
                    n190 = flat-sequence {
                      tunnel: [w618] -> w614
                      tunnel: [w617] -> w613
                      tunnel: [w616] -> w612
                      tunnel: [w616] -> w611
                      tunnel: [w616] -> w610
                      tunnel: [w616] -> w609
                      tunnel: [w616] -> w608
                      tunnel: [w615] -> w607
                      tunnel: [w616] -> w606
                      tunnel: [w616] -> w605
                      tunnel: [w615] -> w604
                      tunnel: w614 -> [w632]
                      tunnel: w613 -> [w642]
                      tunnel: w612 -> [w641]
                      tunnel: w611 -> [w640]
                      tunnel: w610 -> [w639]
                      tunnel: w609 -> [w638]
                      tunnel: w608 -> [w637]
                      tunnel: w607 -> [w636]
                      tunnel: w606 -> [w635]
                      tunnel: w605 -> [w634]
                      tunnel: w604 -> [w633]
                      frame #0 {
                        n191 = local read "Rasterart"() -> (w619:T2)
                        n192 = case shown="\"2D-Scan(yz)\"" w619 {
                          tunnel: [0 ("Index") 2 ("Index") 0 ("Index")] -> w615
                          tunnel: [1 ("Index") 1 ("Index") 2 ("Index")] -> w616
                          tunnel: ["x-Position [mm]" ("X-Achse.Namensbeschriftung.Text") "z-Position [mm]" ("Y-Achse.Namensbeschriftung.Text") "x-Position [mm]" ("Y-Achse.Namensbeschriftung.Text")] -> w618
                          tunnel: ["y-Position [mm]" ("Y-Achse.Namensbeschriftung.Text") "y-Position [mm]" ("X-Achse.Namensbeschriftung.Text") "z-Position [mm]" ("X-Achse.Namensbeschriftung.Text")] -> w617
                          frame #0 {
                          }
                          frame #1 {
                          }
                          frame #2 {
                          }
                        }
                      }
                      frame #1 {
                        w650 = 1000.0 ("y")
                        w669 = 1000.0 ("y")
                        n193 = local read "Rasterweite [µm]"() -> (w674:dbl[])
                        n194 = local read "# Rasterschritte"() -> (w678:i32[])
                        n195 = local read "Rasterweite [µm]"() -> (w645:dbl[])
                        n196 = local read "# Rasterschritte"() -> (w667:i32[])
                        n197 = local read "Start xyz-Position [mm]"() -> (w673:dbl[])
                        n198 = Index Array(array=w678, index #1=w636, index #2=w641) -> (element #1=w676:i32, element #2=w677:i32)
                        n199 = Index Array(array=w674, index #1=w636, index #2=w635) -> (element #1=w670:dbl, element #2=w671:dbl)
                        n200 = local read "# Rasterschritte"() -> (w652:i32[])
                        n201 = Divide(x=w670, y=w669) -> (x/y=w664:dbl)
                        n202 = Divide(x=w671, y=w669) -> (x/y=w666:dbl)
                        n203 = local read "Start xyz-Position [mm]"() -> (w646:dbl[])
                        n204 = Index Array(array=w667, index #1=w636, index #2=w640) -> (element #1=w663:i32, element #2=w665:i32)
                        n205 = Index Array(array=w645, index #1=w636, index #2=w637) -> (element #1=w649:dbl, element #2=w648:dbl)
                        n206 = Initialize Array(0.0 ("y"), w676, w677) -> (w659:dbl[][])
                        n207 = control-ref of="2D-Intensitätsverteilung (MCP)"() -> (w675:refnum<vi>)
                        n208 = Divide(x=w649, y=w650) -> (x/y=w655:dbl)
                        n209 = Divide(x=w648, y=w650) -> (x/y=w653:dbl)
                        n210 = Index Array(array=w673, index #1=w633, index #2=w634) -> (element #1=w672:dbl, element #2=w668:dbl)
                        n211 = Index Array(array=w652, index #1=w636, index #2=w639) -> (element #1=w656:i32, element #2=w654:i32)
                        n212 = Divide(x=w664, y=w663) -> (x/y=w662:dbl)
                        n213 = Divide(x=w666, y=w665) -> (x/y=w661:dbl)
                        n214 = local write "2D-Intensitätsverteilung (LAPD)"(w659) -> ()
                        n215 = local write "2D-Intensitätsverteilung (MCP)"(w659) -> ()
                        n216 = property class="IntGraph (strikt)"(reference=w675, "XScale.Offset"=w672, "XScale.Multiplier"=w662, "YScale.Offset"=w668, "YScale.Multiplier"=w661, "XScale.MinorInc"=w662, "YScale.MinorInc"=w661, "XScale.NameLbl.Text"=w632, "YScale.NameLbl.Text"=w642) -> (error out=w679:errorcluster)  [unwired: 1 in, 1 out]
                        n217 = Index Array(array=w646, index #1=w636, index #2=w638) -> (element #1=w647:dbl, element #2=w651:dbl)
                        n218 = control-ref of="2D-Intensitätsverteilung (LAPD)"() -> (w643:refnum<vi>)
                        n219 = Divide(x=w655, y=w656) -> (x/y=w657:dbl)
                        n220 = Divide(x=w653, y=w654) -> (x/y=w658:dbl)
                        n221 = property class="IntGraph (strikt)"(reference=w643, error in=w679, "XScale.Offset"=w647, "XScale.Multiplier"=w657, "YScale.Offset"=w651, "YScale.Multiplier"=w658, "XScale.MinorInc"=w657, "YScale.MinorInc"=w658, "XScale.NameLbl.Text"=w632, "YScale.NameLbl.Text"=w642) -> (error out=w644:errorcluster)  [unwired: 1 out]
                        n222 = local write "Fehler (Ausgang)"(w644) -> ()
                      }
                    }
                  }
                  frame #2 {
                    n223 = local read "Event: Rasterung gestartet?"() -> (w683:refnum<user-event>)
                    n224 = local write "Rasterung läuft"(TRUE ("x-Linsescan")) -> ()
                    n225 = local read "Aktueller Messschritt"() -> (w682:i32)
                    n226 = Generate User Event(user event=w683, event data cluster=w682) -> (user event out=w681:refnum<user-event>)  [unwired: 1 in, 1 out]
                    n227 = local write "Event: Rasterung gestartet?"(w681) -> ()
                  }
                }
              }
            }
          }
          event #2 {
            n228 = event-data() -> ()  [unwired: 1 in, 1 out]
            n229 = local read "Rasterweite [µm]"() -> (w685:dbl[])
            n230 = local read "# Rasterschritte"() -> (w696:i32[])
            n231 = Replace Array Subset(array=w685, new element #1=0 ("Neues Element/Teil-Array"), index #1=0 ("Index"), new element #2=0 ("Neues Element/Teil-Array"), index #2=1 ("Index"), new element #3=0 ("Neues Element/Teil-Array"), index #3=2 ("Index")) -> (w684:dbl[])
            n232 = Replace Array Subset(array=w696, new element #1=1 ("Neues Element/Teil-Array"), index #1=0 ("Index"), new element #2=1 ("Neues Element/Teil-Array"), index #2=1 ("Index"), new element #3=1 ("Neues Element/Teil-Array"), index #3=2 ("Index")) -> (w692:i32[])
            n233 = local write "Rasterweite [µm]"(w684) -> ()
            n234 = local write "# Rasterschritte"(w692) -> ()
          }
          event #3 {
            n235 = event-data() -> ()  [unwired: 1 in, 1 out]
            n236 = stacked-sequence {
              frame #0 {
                n237 = while "x-Schleife" {
                  i -> [w702]
                  stop <- w703 stop-if-true
                  n238 = local read "# Rasterschritte"() -> (w700:i32[])
                  n239 = local read "x-Achse"() -> (w701:i32)
                  n240 = stacked-sequence {
                    frame #0 {
                      n241 = while "z-Schleife" {
                        i -> [w710]
                        stop <- w712 stop-if-true
                        n242 = local read "# Rasterschritte"() -> (w715:i32[])
                        n243 = stacked-sequence {
                          frame #0 {
                            n244 = while "y-Schleife" {
                              i -> [w721]
                              stop <- w727 stop-if-true
                              # "Schleife für y-Achse"
                              n245 = stacked-sequence {
                                frame #0 {
                                # "Hier findet die Messung statt"
                                n246 = stacked-sequence {
                                frame #0 {
                                n247 = local write "LAPD Spannung (V)"(0.0 ("Transmittierte Intensität (a.u.)")) -> ()
                                n248 = local write "Summierte Helligkeit (a.u.)"(u64 0 ("Summierte Helligkeit (a.u.)")) -> ()
                                n249 = local read "ROI"() -> (w734:i32[])
                                n250 = Index Array(array=w734, index #1=0 ("Index"), index #2=1 ("Index")) -> (element #1=w730:i32, element #2=w731:i32)
                                n251 = local read "Aktueller Messschritt"() -> (w737:i32)
                                n252 = Initialize Array(u64 0 ("Element"), w731, w730) -> (w736:u64[][])
                                n253 = local write "Gemitteltes Bild"(w736) -> ()
                                n254 = Increment(x=w737) -> (x+1=w738:i32)
                                n255 = local write "Aktueller Messschritt"(w738) -> ()
                                }
                                frame #1 {
                                n256 = local read "# Photosignale"() -> (w748:i32)
                                n257 = local read "# Bilder/Messschritt"() -> (w744:i32)
                                n258 = local read "Detektionskamera"() -> (w747:T4)
                                n259 = local read "Einzelbilder speichern"() -> (w742:bool)
                                n260 = for {
                                N: w748 -> [_]
                                n261 = Wait (ms)(milliseconds to wait=u32 10 ("Zu wartende ms")) -> ()  [unwired: 1 out]
                                n262 = local read "LAPD-Kanal (Meilhaus)"() -> (w766:u32)
                                n263 = local read "LAPD Spannung (V)"() -> (w764:dbl)
                                n264 = call "AISingle.vi"("Time Out"=u32 0, "Channel Number"=w766, "Board Number"=u32 0) -> ("Analog Input Voltage"=w765:dbl)
                                n265 = Add(x=w765, y=w764) -> (x+y=w763:dbl)
                                n266 = local write "LAPD Spannung (V)"(w763) -> ()
                                }
                                n267 = call "camera_acquisition_sequence.vi"("Session In"=w747, "Desired image number"=w744) -> ("Image Array"=w741:T3[], "error out"=w746:errorcluster)  [unwired: 2 in, 1 out]
                                n268 = case shown="True" w742 {
                                tunnel: w746 -> [w750 w758]
                                tunnel: [w750 w757] -> w745
                                tunnel: w744 -> [w749 w756]
                                tunnel: [w749 w756] -> w743
                                tunnel: w741 -> [_ w755]
                                frame #0 {
                                }
                                frame #1 {
                                n269 = local read "Aktueller Messschritt"() -> (w761:i32)
                                n270 = local read "Save folder"() -> (w753:string)
                                n271 = Concatenate Strings(w753, "Einzelbilder\\" ("String")) -> (w751:string)
                                n272 = Format Into String(format string="%05.0f" ("Format-String"), initial string="#" ("Eingangs-String"), w761) -> (resulting string=w754:string)  [unwired: 1 in, 1 out]
                                n273 = call "save images.vi"("Save Folder"=w751, "File name prefix"=w754, "Array"=w755, "error out 2"=w758, "Bilder/Messschritt"=w756) -> ("error out"=w757:errorcluster)
                                }
                                }
                                n274 = for {
                                N: w743 -> [_]
                                tunnel: w745 -> [w774]
                                tunnel: w741 -> [w772] mode=indexing
                                n275 = call "IMAQ ImageToArray"("error in (no error)"=w774, "Image"=w772) -> ("error out"=w773:errorcluster, "Image Pixels (U8)"=w771:u8[][])  [unwired: 2 in, 3 out]
                                n276 = local read "Gemitteltes Bild"() -> (w769:u64[][])
                                n277 = To Unsigned Quad Integer(1:w771) -> (0:w776:u64[][])
                                n278 = local write "Fehler (Ausgang)"(w773) -> ()
                                n279 = local read "Summierte Helligkeit (a.u.)"() -> (w777:u64)
                                n280 = Add Array Elements(numeric array=w776) -> (sum=w775:u64)
                                n281 = Add(x=w769, y=w771) -> (x+y=w770:u64[][])
                                n282 = local write "Gemitteltes Bild"(w770) -> ()
                                n283 = Add(x=w775, y=w777) -> (x+y=w778:u64)
                                n284 = local write "Summierte Helligkeit (a.u.)"(w778) -> ()
                                }
                                }
                                frame #2 {
                                n285 = local read "Rasterart"() -> (w788:T2)
                                n286 = case shown="\"2D-Scan(xz)\"" w788 {
                                tunnel: [w810 w811 w813 w814 w816] -> w787
                                tunnel: [w809 w812 w813 w814 w815] -> w786
                                frame #0 {
                                n287 = local read "Current x step"() -> (w810:i32)
                                n288 = local read "Current y step"() -> (w809:i32)
                                }
                                frame #1 {
                                n289 = local read "Current z step"() -> (w811:i32)
                                n290 = local read "Current y step"() -> (w812:i32)
                                }
                                frame #2 {
                                n291 = local read "Current z step"() -> (w813:i32)
                                }
                                frame #3 {
                                n292 = local read "Current x step"() -> (w814:i32)
                                }
                                frame #4 {
                                n293 = local read "Current x step"() -> (w816:i32)
                                n294 = local read "Current z step"() -> (w815:i32)
                                }
                                }
                                n295 = local read "# Bilder/Messschritt"() -> (w783:i32)
                                n296 = local read "Gemitteltes Bild"() -> (w785:u64[][])
                                n297 = local read "2D-Intensitätsverteilung (MCP)"() -> (w790:dbl[][])
                                n298 = local read "2D-Intensitätsverteilung (LAPD)"() -> (w789:dbl[][])
                                n299 = local read "LAPD Spannung (V)"() -> (w794:dbl)
                                n300 = local read "Summierte Helligkeit (a.u.)"() -> (w795:u64)
                                n301 = local read "Gemittelte Bilder speichern"() -> (w779:bool)
                                n302 = local read "# Photosignale"() -> (w793:i32)
                                n303 = local read "Image Display"() -> (w781:T3)
                                n304 = Divide(x=w785, y=w783) -> (x/y=w784:dbl[][])
                                n305 = Divide(x=w794, y=w793) -> (x/y=w791:dbl)
                                n306 = call "IMAQ ArrayToImage"("Image Pixels (U8)"=w784, "Image"=w781) -> ("Image Out"=w782:T3)  [unwired: 8 in, 1 out]
                                n307 = Replace Array Subset(array=w789, new element=w791, index (row)=w787, index (col)=w786) -> (w792:dbl[][])
                                n308 = local write "LAPD Spannung (V)"(w791) -> ()
                                n309 = Replace Array Subset(array=w790, new element=w795, index (row)=w787, index (col)=w786) -> (w796:dbl[][])
                                n310 = case shown="True" w779 {
                                tunnel: w782 -> [w797 w808]
                                tunnel: [w797 w799] -> w780
                                frame #0 {
                                }
                                frame #1 {
                                n311 = local read "Aktueller Messschritt"() -> (w803:i32)
                                n312 = local read "Save folder"() -> (w805:string)
                                n313 = Format Into String(format string="%05.0f" ("Format-String"), initial string="#" ("Eingangs-String"), w803) -> (resulting string=w802:string)  [unwired: 1 in, 1 out]
                                n314 = Concatenate Strings(w805, "Gemittelte Bilder\\" ("String"), w802, ".png" ("String")) -> (w801:string)
                                n315 = String To Path(string=w801) -> (path=w800:path)
                                n316 = call-poly "IMAQ Write File 2"("File Path"=w800, "Image"=w808) -> ("Image Out (duplicate)"=w799:T3)  [unwired: 8 in, 1 out]
                                }
                                }
                                n317 = local write "2D-Intensitätsverteilung (LAPD)"(w792) -> ()
                                n318 = local write "2D-Intensitätsverteilung (MCP)"(w796) -> ()
                                n319 = local write "Image Display"(w780) -> ()
                                }
                                }
                                }
                                frame #1 {
                                n320 = local read "Rasterschritt [µm]"() -> (w826:dbl[])
                                n321 = local read "y-Achse"() -> (w822:i32)
                                n322 = Decrement(x=w822) -> (x-1=w825:i32)
                                n323 = Index Array(array=w826, index=w825) -> (element=w821:dbl)
                                n324 = local read "Aktueller Messschritt"() -> (w819:i32)
                                n325 = local read "Start time [ms]"() -> (w820:timestamp)
                                n326 = local read "# Messschritte"() -> (w818:i32)
                                n327 = Not Equal?(x=w821, y=0.0) -> (x != y?=w823:bool)
                                n328 = case shown="True" w823 {
                                tunnel: w822 -> [_ w828]
                                tunnel: w821 -> [_ w827]
                                frame #0 {
                                }
                                frame #1 {
                                # "Fahre nächste y-Position an"
                                n329 = call "stage_move_axis_relative.vi"("Achse"=w828, "Schrittweite [µm]"=w827) -> ("error out"=w830:errorcluster, "xyz-Position OUT [mm]"=w829:dbl[])  [unwired: 1 in, 1 out]
                                n330 = local write "Aktuelle xyz-Position [mm]"(w829) -> ()
                                n331 = local write "Fehler (Ausgang)"(w830) -> ()
                                }
                                }
                                n332 = call "estimate_stopp_time.vi"("Aktueller Messschritt"=w819, "# Messschritte"=w818, "Startzeit"=w820) -> ("Stopp Zeit"=w817:string)  [unwired: 8 in]
                                n333 = local write "Geschätzte Messzeit"(w817) -> ()
                                }
                              }
                              n334 = local read "# Rasterschritte"() -> (w726:i32[])
                              n335 = local read "y-Achse"() -> (w720:i32)
                              n336 = local read "Rasterung ON/OFF"() -> (w728:bool)
                              n337 = Decrement(x=w720) -> (x-1=w722:i32)
                              n338 = Increment(x=w721) -> (x+1=w723:i32)
                              n339 = Index Array(array=w726, index=w722) -> (element=w725:i32)
                              n340 = Equal?(x=w725, y=w723) -> (x = y?=w724:bool)
                              n341 = Not(x=w728) -> (.not. x?=w729:bool)
                              n342 = Or(x=w724, y=w729) -> (x .or. y?=w727:bool)
                              "Current y step" <- w721
                            }
                          }
                          frame #1 {
                            n343 = flat-sequence {
                              frame #0 {
                                n344 = local read "Rasterschritt [µm]"() -> (w837:dbl[])
                                n345 = local read "y-Achse"() -> (w832:i32)
                                n346 = local read "Start xyz-Position [mm]"() -> (w831:dbl[])
                                n347 = Decrement(x=w832) -> (x-1=w836:i32)
                                n348 = Index Array(array=w837, index=w836) -> (element=w835:dbl)
                                n349 = Not Equal?(x=w835, y=0.0) -> (x != y?=w833:bool)
                                n350 = case shown="True" w833 {
                                tunnel: w832 -> [_ w839]
                                tunnel: w831 -> [_ w838]
                                frame #0 {
                                }
                                frame #1 {
                                # "Fahre Startposition für y an"
                                n351 = call "stage_move_axis_absolute.vi"("Ziel xyz IN [mm]"=w838, "Achse"=w839) -> ("error out"=w841:errorcluster, "Ziel xyz OUT [mm]"=w840:dbl[])  [unwired: 1 in, 1 out]
                                n352 = local write "Aktuelle xyz-Position [mm]"(w840) -> ()
                                n353 = local write "Fehler (Ausgang)"(w841) -> ()
                                }
                                }
                              }
                              frame #1 {
                                n354 = local read "Rasterschritt [µm]"() -> (w847:dbl[])
                                n355 = local read "z-Achse"() -> (w842:i32)
                                n356 = Decrement(x=w842) -> (x-1=w843:i32)
                                n357 = Index Array(array=w847, index=w843) -> (element=w844:dbl)
                                n358 = Not Equal?(x=w844, y=0.0) -> (x != y?=w845:bool)
                                n359 = case shown="True" w845 {
                                tunnel: w844 -> [_ w849]
                                tunnel: w842 -> [_ w848]
                                frame #0 {
                                }
                                frame #1 {
                                # "Fahre nächste Position für z an"
                                n360 = call "stage_move_axis_relative.vi"("Achse"=w848, "Schrittweite [µm]"=w849) -> ("error out"=w850:errorcluster, "xyz-Position OUT [mm]"=w851:dbl[])  [unwired: 1 in, 1 out]
                                n361 = local write "Aktuelle xyz-Position [mm]"(w851) -> ()
                                n362 = local write "Fehler (Ausgang)"(w850) -> ()
                                }
                                }
                              }
                            }
                          }
                        }
                        n363 = local read "z-Achse"() -> (w711:i32)
                        n364 = local read "Rasterung ON/OFF"() -> (w714:bool)
                        n365 = Decrement(x=w711) -> (x-1=w719:i32)
                        n366 = Increment(x=w710) -> (x+1=w718:i32)
                        n367 = Index Array(array=w715, index=w719) -> (element=w716:i32)
                        n368 = Equal?(x=w716, y=w718) -> (x = y?=w717:bool)
                        n369 = Not(x=w714) -> (.not. x?=w713:bool)
                        n370 = Or(x=w717, y=w713) -> (x .or. y?=w712:bool)
                        "Current z step" <- w710
                      }
                    }
                    frame #1 {
                      n371 = flat-sequence {
                        frame #0 {
                          n372 = local read "Rasterschritt [µm]"() -> (w855:dbl[])
                          n373 = local read "z-Achse"() -> (w852:i32)
                          n374 = local read "Start xyz-Position [mm]"() -> (w853:dbl[])
                          n375 = Decrement(x=w852) -> (x-1=w856:i32)
                          n376 = Index Array(array=w855, index=w856) -> (element=w857:dbl)
                          n377 = Not Equal?(x=w857, y=0.0) -> (x != y?=w854:bool)
                          n378 = case shown="True" w854 {
                            tunnel: w853 -> [_ w860]
                            tunnel: w852 -> [_ w859]
                            frame #0 {
                            }
                            frame #1 {
                              # "Fahre Startposition für z an"
                              n379 = call "stage_move_axis_absolute.vi"("Ziel xyz IN [mm]"=w860, "Achse"=w859) -> ("error out"=w861:errorcluster, "Ziel xyz OUT [mm]"=w862:dbl[])  [unwired: 1 in, 1 out]
                              n380 = local write "Aktuelle xyz-Position [mm]"(w862) -> ()
                              n381 = local write "Fehler (Ausgang)"(w861) -> ()
                            }
                          }
                        }
                        frame #1 {
                          n382 = local read "Rasterschritt [µm]"() -> (w868:dbl[])
                          n383 = local read "x-Achse"() -> (w863:i32)
                          n384 = Decrement(x=w863) -> (x-1=w867:i32)
                          n385 = Index Array(array=w868, index=w867) -> (element=w866:dbl)
                          n386 = Not Equal?(x=w866, y=0.0) -> (x != y?=w864:bool)
                          n387 = case shown="True" w864 {
                            tunnel: w866 -> [_ w871]
                            tunnel: w863 -> [_ w869]
                            frame #0 {
                            }
                            frame #1 {
                              # "Fahre nächste Position für x an"
                              n388 = call "stage_move_axis_relative.vi"("Achse"=w869, "Schrittweite [µm]"=w871) -> ("error out"=w872:errorcluster, "xyz-Position OUT [mm]"=w870:dbl[])  [unwired: 1 in, 1 out]
                              n389 = local write "Aktuelle xyz-Position [mm]"(w870) -> ()
                              n390 = local write "Fehler (Ausgang)"(w872) -> ()
                            }
                          }
                        }
                      }
                    }
                  }
                  n391 = local read "Rasterung ON/OFF"() -> (w708:bool)
                  n392 = Decrement(x=w701) -> (x-1=w704:i32)
                  n393 = Increment(x=w702) -> (x+1=w705:i32)
                  n394 = Index Array(array=w700, index=w704) -> (element=w707:i32)
                  n395 = Equal?(x=w707, y=w705) -> (x = y?=w706:bool)
                  n396 = Not(x=w708) -> (.not. x?=w709:bool)
                  n397 = Or(x=w706, y=w709) -> (x .or. y?=w703:bool)
                  "Current x step" <- w702
                }
              }
              frame #1 {
                n398 = local read "Summierte Helligkeit speichern"() -> (w887:bool)
                n399 = local read "LAPD-Daten speichern"() -> (w886:bool)
                n400 = local read "Summierte Helligkeit speichern"() -> (w875:bool)
                n401 = local read "Gemittelte Bilder speichern"() -> (w876:bool)
                n402 = local read "2D-Intensitätsverteilung (MCP)"() -> (w885:dbl[][])
                n403 = local read "2D-Intensitätsverteilung (LAPD)"() -> (w881:dbl[][])
                n404 = local read "LAPD-Daten speichern"() -> (w874:bool)
                n405 = local read "Einzelbilder speichern"() -> (w873:bool)
                n406 = flat-sequence {
                  frame #0 {
                    # "Zur Ausgangsposition zurückfahren"
                    n407 = local read "Start xyz-Position [mm]"() -> (w967:dbl[])
                    n408 = local read "Detektionskamera"() -> (w957:T4)
                    n409 = local read "Buffer Interval"() -> (w956:u32)
                    n410 = call "camera_create_configuration.vi"("BufferInterval"=w956, "Session Out 2"=w957) -> ("Fehler (Ausgang)"=w955:errorcluster, "Ereignisregistrierung (Referenz)"=w958:refnum<event-registration>)  [unwired: 1 in, 1 out]
                    n411 = local write "Ereignis: FrameDone?"(w958) -> ()
                    n412 = local read "x-Achse"() -> (w964:i32)
                    n413 = call "stage_move_axis_absolute.vi"("error in"=w955, "Ziel xyz IN [mm]"=w967, "Achse"=w964) -> ("error out"=w960:errorcluster)  [unwired: 2 out]
                    n414 = local read "y-Achse"() -> (w965:i32)
                    n415 = call "stage_move_axis_absolute.vi"("error in"=w960, "Ziel xyz IN [mm]"=w967, "Achse"=w965) -> ("error out"=w961:errorcluster)  [unwired: 2 out]
                    n416 = local read "z-Achse"() -> (w966:i32)
                    n417 = call "stage_move_axis_absolute.vi"("error in"=w961, "Ziel xyz IN [mm]"=w967, "Achse"=w966) -> ("error out"=w962:errorcluster, "Fertig?"=w963:bool, "Ziel xyz OUT [mm]"=w968:dbl[])
                    n418 = Not(x=w963) -> (.not. x?=w959:bool)
                    n419 = local write "Aktuelle xyz-Position [mm]"(w968) -> ()
                    n420 = local write "Fehler (Ausgang)"(w962) -> ()
                    n421 = local write "Rasterung ON/OFF"(w959) -> ()
                    n422 = local write "Rasterung läuft"(w959) -> ()
                  }
                }
                n423 = control-ref of="2D-Intensitätsverteilung (MCP)"() -> (w884:refnum<vi>)
                n424 = control-ref of="2D-Intensitätsverteilung (LAPD)"() -> (w878:refnum<vi>)
                n425 = case shown="True" w886 {
                  frame #0 {
                  }
                  frame #1 {
                    n426 = local read "Save folder"() -> (w973:string)
                    n427 = local read "2D-Intensitätsverteilung (LAPD)"() -> (w971:dbl[][])
                    n428 = Concatenate Strings(w973, "\\" ("String"), "2D_Intensitaetsverteilung_LAPD.dat" ("String")) -> (w975:string)
                    n429 = String To Path(string=w975) -> (path=w974:path)
                    n430 = call-poly <vilib>:"Write To Spreadsheet File.vi"("format (%.3f)"="%.;%.5f", "2D data"=w971, "file path (dialog if empty)"=w974) -> ()  [unwired: 5 in, 1 out]
                  }
                }
                n431 = Compound Arithmetic op=OR(w873, w874, w876, w875) -> (w877:bool)
                n432 = case shown="True" w887 {
                  frame #0 {
                  }
                  frame #1 {
                    n433 = local read "Save folder"() -> (w979:string)
                    n434 = local read "2D-Intensitätsverteilung (MCP)"() -> (w981:dbl[][])
                    n435 = Concatenate Strings(w979, "\\" ("String"), "2D_Intensitaetsverteilung_MCP.dat" ("String")) -> (w977:string)
                    n436 = String To Path(string=w977) -> (path=w978:path)
                    n437 = call-poly <vilib>:"Write To Spreadsheet File.vi"("format (%.3f)"="%.;%8.0f", "2D data"=w981, "file path (dialog if empty)"=w978) -> ()  [unwired: 5 in, 1 out]
                  }
                }
                n438 = case shown="True" w877 {
                  frame #0 {
                  }
                  frame #1 {
                    n439 = local read "Rasterschritt [µm]"() -> (w889:dbl[])
                    n440 = local read "Start xyz-Position [mm]"() -> (w892:dbl[])
                    n441 = local read "# Rasterschritte"() -> (w893:i32[])
                    n442 = local read "Save folder"() -> (w891:string)
                    n443 = Divide(x=w889, y=1000) -> (x/y=w890:dbl[])
                    n444 = local read "Rasterart"() -> (w894:T2)
                    n445 = case shown="\"2D-Scan(xz)\"" w894 {
                      tunnel: w893 -> [w897 w904 w916 w937 w947]
                      tunnel: w892 -> [w895 w906 w914 w938 w949]
                      tunnel: w891 -> [w898 w907 w913 w936 w950]
                      tunnel: w890 -> [w896 w905 w915 w927 w948]
                      frame #0 {
                        w903 = 0 ("Index")
                        n446 = Index Array(array=w895, index=w903) -> (element=w901:dbl)
                        n447 = Index Array(array=w896, index=w903) -> (element=w899:dbl)
                        n448 = Index Array(array=w897, index=w903) -> (element=w900:i32)
                        n449 = call "create_axis_vector_file.vi"("Save folder"=w898, "Dateiname"="xAchse.dat", "Start"=w901, "Schrittlänge"=w899, "# Schritte"=w900) -> ()  [unwired: 11 in]
                      }
                      frame #1 {
                        w912 = 2 ("Index")
                        n450 = Index Array(array=w906, index=w912) -> (element=w910:dbl)
                        n451 = Index Array(array=w905, index=w912) -> (element=w908:dbl)
                        n452 = Index Array(array=w904, index=w912) -> (element=w909:i32)
                        n453 = call "create_axis_vector_file.vi"("Save folder"=w907, "Dateiname"="xAchse.dat", "Start"=w910, "Schrittlänge"=w908, "# Schritte"=w909) -> ()  [unwired: 11 in]
                      }
                      frame #2 {
                        w925 = 1 ("Index")
                        w926 = 0 ("Index")
                        n454 = Index Array(array=w914, index #1=w926, index #2=w925) -> (element #1=w922:dbl, element #2=w919:dbl)
                        n455 = Index Array(array=w915, index #1=w926, index #2=w925) -> (element #1=w920:dbl, element #2=w918:dbl)
                        n456 = Index Array(array=w916, index #1=w926, index #2=w925) -> (element #1=w921:i32, element #2=w917:i32)
                        n457 = call "create_axis_vector_file.vi"("Save folder"=w913, "Dateiname"="yAchse.dat", "Start"=w919, "Schrittlänge"=w918, "# Schritte"=w917) -> ()  [unwired: 11 in]
                        n458 = call "create_axis_vector_file.vi"("Save folder"=w913, "Dateiname"="xAchse.dat", "Start"=w922, "Schrittlänge"=w920, "# Schritte"=w921) -> ()  [unwired: 11 in]
                      }
                      frame #3 {
                        w939 = 2 ("Index")
                        w940 = 1 ("Index")
                        n459 = Index Array(array=w938, index #1=w940, index #2=w939) -> (element #1=w933:dbl, element #2=w930:dbl)
                        n460 = Index Array(array=w927, index #1=w940, index #2=w939) -> (element #1=w931:dbl, element #2=w929:dbl)
                        n461 = Index Array(array=w937, index #1=w940, index #2=w939) -> (element #1=w932:i32, element #2=w928:i32)
                        n462 = call "create_axis_vector_file.vi"("Save folder"=w936, "Dateiname"="xAchse.dat", "Start"=w930, "Schrittlänge"=w929, "# Schritte"=w928) -> ()  [unwired: 11 in]
                        n463 = call "create_axis_vector_file.vi"("Save folder"=w936, "Dateiname"="yAchse.dat", "Start"=w933, "Schrittlänge"=w931, "# Schritte"=w932) -> ()  [unwired: 11 in]
                      }
                      frame #4 {
                        w953 = 2 ("Index")
                        w954 = 0 ("Index")
                        n464 = Index Array(array=w949, index #1=w954, index #2=w953) -> (element #1=w946:dbl, element #2=w941:dbl)
                        n465 = Index Array(array=w948, index #1=w954, index #2=w953) -> (element #1=w945:dbl, element #2=w942:dbl)
                        n466 = Index Array(array=w947, index #1=w954, index #2=w953) -> (element #1=w944:i32, element #2=w943:i32)
                        n467 = call "create_axis_vector_file.vi"("Save folder"=w950, "Dateiname"="xAchse.dat", "Start"=w946, "Schrittlänge"=w945, "# Schritte"=w944) -> ()  [unwired: 11 in]
                        n468 = call "create_axis_vector_file.vi"("Save folder"=w950, "Dateiname"="yAchse.dat", "Start"=w941, "Schrittlänge"=w942, "# Schritte"=w943) -> ()  [unwired: 11 in]
                      }
                    }
                  }
                }
                n469 = Array Max & Min(array=w881) -> (max value=w880:dbl, min value=w879:dbl)  [unwired: 2 out]
                n470 = Array Max & Min(array=w885) -> (max value=w883:dbl, min value=w882:dbl)  [unwired: 2 out]
                n471 = property class="IntGraph (strikt)"(reference=w878, "ZScale.Maximum"=w880, "ZScale.Minimum"=w879) -> ()  [unwired: 1 in, 2 out]
                n472 = property class="IntGraph (strikt)"(reference=w884, "ZScale.Maximum"=w883, "ZScale.Minimum"=w882) -> ()  [unwired: 1 in, 2 out]
              }
            }
          }
          event #4 {
            n473 = event-data() -> ("NewVal"=w985:bool)  [unwired: 1 in]
            n474 = local read "Kamera"() -> (w986:bool)
            n475 = local read "HV-Steuerung"() -> (w983:bool)
            n476 = Compound Arithmetic op=AND(w986, w985, w983) -> (w984:bool)
            n477 = case shown="True" w984 {
              frame #0 {
                n478 = local write "Spannungsscan läuft"(FALSE ("Messung läuft")) -> ()
              }
              frame #1 {
                n479 = stacked-sequence {
                  frame #0 {
                    n480 = flat-sequence {
                      tunnel: [w1001] -> w988
                      tunnel: w988 -> [w1017]
                      frame #0 {
                        n481 = control-ref of="Shutter time (ms)"() -> (w1014:refnum<vi>)
                        n482 = local read "Suppressor-Spannung [V]"() -> (w991:dbl)
                        n483 = property class="Ring (strikt)"(reference=w1014) -> ("RingText.Text"=w1013:string)  [unwired: 1 in, 2 out]
                        n484 = local read "# Bilder/Messschritt"() -> (w1007:i32)
                        n485 = local read "Spannungsstart [V]"() -> (w995:dbl[])
                        n486 = local read "# Spannungsschritte"() -> (w1010:i32[])
                        n487 = local read "Spannungsweite [V]"() -> (w1009:dbl[])
                        n488 = local read "Tip-Spannung [V]"() -> (w992:dbl)
                        n489 = local read "P-Schirm-Spannung [V]"() -> (w999:dbl)
                        n490 = local write "Aktueller Messschritt"(0 ("Aktueller Messschritt")) -> ()
                        n491 = local read "MCP-Spannung [V]"() -> (w998:dbl)
                        n492 = local read "Leistung (iK) [mW]"() -> (w997:dbl)
                        n493 = local read "Polarisation [°]"() -> (w1004:dbl)
                        n494 = local read "Messlogbuch"() -> (w1006:path)
                        n495 = Decimal String To Number(string=w1013) -> (number=w996:i32)  [unwired: 2 in, 1 out]
                        n496 = local read "Proben-ID"() -> (w1005:string)
                        n497 = Multiply(x=w1007, y=w996) -> (x*y=w1008:i32)
                        n498 = Divide(x=w1009, y=w1010) -> (x/y=w1011:dbl[])
                        n499 = local read "ROI"() -> (w1002:i32[])
                        n500 = Replace Array Subset(array=w995, new element #1=w992, index #1=0 ("Index"), new element #2=w991, index #2=1 ("Index")) -> (w990:dbl[])
                        n501 = local write "Spannungsschritt [V]"(w1011) -> ()
                        n502 = Get Date/Time In Seconds() -> (seconds since 1Jan1904=w989:timestamp)
                        n503 = local write "Aktuelle Spannung [V]"(w990) -> ()
                        n504 = call "stage_get_current_xyz.vi"() -> ("Aktuelle xyz-Position OUT [mm]"=w1000:dbl[])  [unwired: 3 in, 1 out]
                        n505 = call "create_measure_log_entry.vi"("Messlogbuch-Pfad"=w1006, "Probe"=w1005, "Polarisation [°]"=w1004, "Messart"="Spannungsscan", "ROI"=w1002, "Messungen/Messschritt"=w1007, "Maximalleistung (iK) [mW]"=w997, "Tip-Spannung [V]"=w992, "Suppressor-Spannung [V]"=w991, "Zeit/Messschritt [ms]"=w996, "MCP-Spannung [V]"=w998, "Zeit/Messung [ms]"=w1008, "Phosphorschirm-Spannung [V]"=w999, "xyz [mm]"=w1000) -> ("Messung Nr."=w1001:i32)  [unwired: 4 in, 1 out]
                        n506 = local write "Start time [ms]"(w989) -> ()
                        n507 = local write "Spannungsstart [V]"(w990) -> ()
                      }
                      frame #1 {
                        n508 = local read "Day folder"() -> (w1023:string)
                        n509 = local read "Fehler (Ausgang)"() -> (w1018:errorcluster)
                        n510 = local read "# Spannungsschritte"() -> (w1032:i32[])
                        n511 = local read "Einzelbilder speichern"() -> (w1025:bool)
                        n512 = call "create_save_folder.vi"("Day folder"=w1023, "Measuring number"=w1017, "Measuring folder"="Spannungsscan" ("Subfolder"), "error in"=w1018) -> ("Save Folder"=w1022:string, "Error Out"=w1021:errorcluster)  [unwired: 5 in]
                        n513 = local write "Save folder"(w1022) -> ()
                        n514 = Index Array(array=w1032, index #1=0 ("Index"), index #2=1 ("Index")) -> (element #1=w1029:i32, element #2=w1028:i32)
                        n515 = local read "Gemittelte Bilder speichern"() -> (w1026:bool)
                        n516 = Multiply(x=w1029, y=w1028) -> (x*y=w1015:i32)
                        n517 = local read "Kamera"() -> (w1027:bool)
                        n518 = case shown="True" w1025 {
                          tunnel: w1021 -> [w1033 w1035]
                          tunnel: [w1033 w1034] -> w1020
                          frame #0 {
                          }
                          frame #1 {
                            n519 = local read "Save folder"() -> (w1038:string)
                            n520 = Concatenate Strings(w1038, "\\Einzelbilder" ("Subfolder")) -> (w1036:string)
                            n521 = String To Path(string=w1036) -> (path=w1039:path)
                            n522 = call <vilib>:"Check if File or Folder Exists.vi"("error in (no error)"=w1035, "path"=w1039) -> ("error out"=w1034:errorcluster, "file or folder exists?"=w1040:bool, "dup path"=w1041:path)  [unwired: 7 in]
                            n523 = case shown="False" w1040 {
                              tunnel: w1041 -> [w1042 _]
                              frame #0 {
                                n524 = Create Folder(path (use dialog)=w1042) -> ()  [unwired: 2 in, 3 out]
                              }
                              frame #1 {
                              }
                            }
                          }
                        }
                        n525 = local write "# Messschritte"(w1015) -> ()
                        n526 = case shown="True" w1026 {
                          tunnel: w1020 -> [w1043 w1045]
                          tunnel: [w1043 w1044] -> w1019
                          frame #0 {
                          }
                          frame #1 {
                            n527 = local read "Save folder"() -> (w1049:string)
                            n528 = Concatenate Strings(w1049, "\\Gemittelte Bilder" ("Subfolder")) -> (w1051:string)
                            n529 = String To Path(string=w1051) -> (path=w1048:path)
                            n530 = call <vilib>:"Check if File or Folder Exists.vi"("error in (no error)"=w1045, "path"=w1048) -> ("error out"=w1044:errorcluster, "file or folder exists?"=w1047:bool, "dup path"=w1046:path)  [unwired: 7 in]
                            n531 = case shown="False" w1047 {
                              tunnel: w1046 -> [w1052 _]
                              frame #0 {
                                n532 = Create Folder(path (use dialog)=w1052) -> ()  [unwired: 2 in, 3 out]
                              }
                              frame #1 {
                              }
                            }
                          }
                        }
                        n533 = case shown="True" w1027 {
                          tunnel: [w1053 w1055] -> w1016
                          tunnel: w1019 -> [w1053 w1054]
                          frame #0 {
                          }
                          frame #1 {
                            n534 = local read "Ereignis: FrameDone?"() -> (w1056:refnum<event-registration>)
                            n535 = local read "Detektionskamera"() -> (w1057:T4)
                            n536 = call "camera_release_configuration.vi"("error in"=w1054, "Session In"=w1057, "Ereignisregistrierung (Referenz) 2"=w1056) -> ("error out"=w1055:errorcluster)  [unwired: 1 out]
                          }
                        }
                        n537 = local write "Fehler (Ausgang)"(w1016) -> ()
                      }
                    }
                  }
                  frame #1 {
                    n538 = flat-sequence {
                      frame #0 {
                        w1063 = 1 ("Index")
                        w1064 = 0 ("Index")
                        n539 = local read "Spannungsstart [V]"() -> (w1059:dbl[])
                        n540 = local read "# Spannungsschritte"() -> (w1074:i32[])
                        n541 = local read "Spannungsschritt [V]"() -> (w1062:dbl[])
                        n542 = Index Array(array=w1074, index #1=w1064, index #2=w1063) -> (element #1=w1072:i32, element #2=w1073:i32)
                        n543 = control-ref of="2D-Intensitätsverteilung (MCP)"() -> (w1058:refnum<vi>)
                        n544 = Initialize Array(0.0 ("y"), w1072, w1073) -> (w1070:dbl[][])
                        n545 = Index Array(array=w1062, index #1=w1064, index #2=w1063) -> (element #1=w1066:dbl, element #2=w1065:dbl)
                        n546 = Index Array(array=w1059, index #1=w1064, index #2=w1063) -> (element #1=w1061:dbl, element #2=w1060:dbl)
                        n547 = local write "2D-Intensitätsverteilung (MCP)"(w1070) -> ()
                        n548 = property class="IntGraph (strikt)"(reference=w1058, "XScale.Offset"=w1061, "XScale.Multiplier"=w1066, "YScale.Offset"=w1060, "YScale.Multiplier"=w1065, "XScale.MinorInc"=w1066, "YScale.MinorInc"=w1065, "XScale.NameLbl.Text"="Tip-Spannung [V]" ("Y-Achse.Namensbeschriftung.Text"), "YScale.NameLbl.Text"="Suppressor-Spannung [V]" ("X-Achse.Namensbeschriftung.Text")) -> (error out=w1069:errorcluster)  [unwired: 1 in, 1 out]
                        n549 = local write "Fehler (Ausgang)"(w1069) -> ()
                      }
                      frame #1 {
                        n550 = local write "Spannungsscan läuft"(TRUE ("Messung läuft")) -> ()
                      }
                    }
                  }
                }
              }
            }
          }
          event #5 {
            n551 = event-data() -> ("NewVal"=w1078:bool)  [unwired: 1 in]
            n552 = local read "Kamera"() -> (w1079:bool)
            n553 = local read "HV-Steuerung"() -> (w1076:bool)
            n554 = Compound Arithmetic op=AND(w1079, w1078, w1076) -> (w1077:bool)
            n555 = case shown="True" w1077 {
              frame #0 {
                n556 = local write "x-U-Scan läuft"(FALSE ("Messung läuft")) -> ()
              }
              frame #1 {
                n557 = stacked-sequence {
                  frame #0 {
                    # "Falls der gewählte Startwert für den Scan und der Startwert zur Berechnung der Ausgleichslage nicht identisch sind muss ein korrigierter Wert für die Raum-Koordinate 2 angefahren werden"
                    n558 = local read "x-U-Scan (Ausgleichslage) Steigung"() -> (w1082:dbl)
                    n559 = Not Equal?(x=w1082, y=0.0) -> (x != y?=w1083:bool)
                    n560 = case shown="True" w1083 {
                      frame #0 {
                      }
                      frame #1 {
                        n561 = flat-sequence {
                          tunnel: [w1086] -> w1084
                          tunnel: w1084 -> [w1099]
                          frame #0 {
                            n562 = local read "x-U-Scan (Ausgleichslage) xy-Start [mm]"() -> (w1097:dbl[])
                            n563 = local read "Raum-Koordinate 2 (Lagenausgleich)"() -> (w1086:enum16{"x-Achse", "y-Achse", "z-Achse"})
                            n564 = local read "Raum-Koordinate 1"() -> (w1095:enum16{"x-Achse", "y-Achse", "z-Achse"})
                            n565 = local read "x-U-Scan (Ausgleichslage) Steigung"() -> (w1092:dbl)
                            n566 = call "stage_get_current_xyz.vi"() -> ("Aktuelle xyz-Position OUT [mm]"=w1088:dbl[])  [unwired: 3 in, 1 out]
                            n567 = Index Array(array=w1097, index #1=w1095, index #2=w1086) -> (element #1=w1096:dbl, element #2=w1089:dbl)
                            n568 = Index Array(array=w1088, index=w1095) -> (element=w1094:dbl)
                            n569 = Subtract(x=w1094, y=w1096) -> (x-y=w1093:dbl)
                            n570 = local write "x-U-Scan x-Startposition [mm]"(w1094) -> ()
                            n571 = Multiply(x=w1093, y=w1092) -> (x*y=w1090:dbl)
                            n572 = Increment(x=w1086) -> (x+1=w1091:enum16{"x-Achse", "y-Achse", "z-Achse"})
                            n573 = Add(x=w1090, y=w1089) -> (x+y=w1085:dbl)
                            n574 = Replace Array Subset(array=w1088, new element=w1085, index=w1086) -> (w1087:dbl[])
                            n575 = call "stage_move_axis_absolute.vi"("Ziel xyz IN [mm]"=w1087, "Achse"=w1091) -> ()  [unwired: 1 in, 3 out]
                          }
                          frame #1 {
                            n576 = call "stage_get_current_xyz.vi"() -> ("Aktuelle xyz-Position OUT [mm]"=w1100:dbl[])  [unwired: 3 in, 1 out]
                            n577 = Index Array(array=w1100, index=w1099) -> (element=w1098:dbl)
                            n578 = local write "Start xyz-Position [mm]"(w1100) -> ()
                            n579 = local write "x-U-Scan y-Startposition [mm]"(w1098) -> ()
                          }
                        }
                      }
                    }
                  }
                  frame #1 {
                    n580 = flat-sequence {
                      tunnel: [w1116] -> w1101
                      tunnel: w1101 -> [w1142]
                      frame #0 {
                        n581 = local read "Raum-Koordinate 2 (Lagenausgleich)"() -> (w1104:enum16{"x-Achse", "y-Achse", "z-Achse"})
                        n582 = local read "Raum-Koordinate 1"() -> (w1105:enum16{"x-Achse", "y-Achse", "z-Achse"})
                        n583 = local read "# x-U-Scan x-Rasterschritte"() -> (w1128:i32)
                        n584 = local read "# x-U-Scan Spannungsschritte"() -> (w1131:i32)
                        n585 = local read "x-U-Scan x-Rasterweite [µm]"() -> (w1129:dbl)
                        n586 = local read "x-U-Scan Spannungsweite [V]"() -> (w1130:dbl)
                        n587 = local read "# Bilder/Messschritt"() -> (w1117:i32)
                        n588 = local read "ROI"() -> (w1120:i32[])
                        n589 = Add(x=w1105, y=1) -> (x+y=w1109:i32)
                        n590 = local write "Aktueller Messschritt"(0 ("Aktueller Messschritt")) -> ()
                        n591 = local write "Achs-ID"(w1109) -> ()
                        n592 = control-ref of="Shutter time (ms)"() -> (w1135:refnum<vi>)
                        n593 = call "stage_get_current_xyz.vi"() -> ("Aktuelle xyz-Position OUT [mm]"=w1106:dbl[])  [unwired: 3 in, 1 out]
                        n594 = local read "Spannungs-Koordinate"() -> (w1126:enum16{"Tip-Spannung", "Suppressor-Spannung"})
                        n595 = property class="Ring (strikt)"(reference=w1135) -> ("RingText.Text"=w1134:string)  [unwired: 1 in, 2 out]
                        n596 = local read "Tip-Spannung [V]"() -> (w1111:dbl)
                        n597 = Divide(x=w1129, y=w1128) -> (x/y=w1127:dbl)
                        n598 = Divide(x=w1130, y=w1131) -> (x/y=w1132:dbl)
                        n599 = Index Array(array=w1106, index #1=w1105, index #2=w1104) -> (element #1=w1102:dbl, element #2=w1103:dbl)
                        n600 = local write "x-U-Scan y-Startposition [mm]"(w1103) -> ()
                        n601 = local write "x-U-Scan x-Startposition [mm]"(w1102) -> ()
                        n602 = local write "x-U-Scan x-Rasterschritt [µm]"(w1127) -> ()
                        n603 = local read "P-Schirm-Spannung [V]"() -> (w1115:dbl)
                        n604 = local write "x-U-Scan Spannungsschritt [V]"(w1132) -> ()
                        n605 = Decimal String To Number(string=w1134) -> (number=w1118:i32)  [unwired: 2 in, 1 out]
                        n606 = local read "MCP-Spannung [V]"() -> (w1114:dbl)
                        n607 = case shown="\"Suppressor-Spannung\", Voreinstellung" w1126 {
                          tunnel: [refnum<k21> "Dev0/Ao1" ("Spannungskanal") refnum<k21> "Dev0/Ao0" ("Spannungskanal")] -> w1125
                          tunnel: [w1136 w1138] -> w1108
                          frame #0 {
                            n608 = local read "Tip-Spannung [V]"() -> (w1136:dbl)
                          }
                          frame #1 {
                            n609 = local read "Suppressor-Spannung [V]"() -> (w1138:dbl)
                          }
                        }
                        n610 = local read "Leistung (iK) [mW]"() -> (w1113:dbl)
                        n611 = local read "Polarisation [°]"() -> (w1122:dbl)
                        n612 = Get Date/Time In Seconds() -> (seconds since 1Jan1904=w1107:timestamp)
                        n613 = local read "Messlogbuch"() -> (w1124:path)
                        n614 = local read "Proben-ID"() -> (w1123:string)
                        n615 = local read "Suppressor-Spannung [V]"() -> (w1112:dbl)
                        n616 = Multiply(x=w1117, y=w1118) -> (x*y=w1119:i32)
                        n617 = local write "Start time [ms]"(w1107) -> ()
                        n618 = local write "x-U-Scan aktuelle y-Position [mm]"(w1103) -> ()
                        n619 = local write "x-U-Scan aktuelle x-Position [mm]"(w1102) -> ()
                        n620 = local write "Spannungskanal"(w1125) -> ()
                        n621 = local write "x-U-Scan aktuelle Spannung [V]"(w1108) -> ()
                        n622 = local write "x-U-Scan Spannungsstart [V]"(w1108) -> ()
                        n623 = local write "Start xyz-Position [mm]"(w1106) -> ()
                        n624 = call "create_measure_log_entry.vi"("Messlogbuch-Pfad"=w1124, "Probe"=w1123, "Polarisation [°]"=w1122, "Messart"="x-U-Scan", "ROI"=w1120, "Messungen/Messschritt"=w1117, "Maximalleistung (iK) [mW]"=w1113, "Tip-Spannung [V]"=w1111, "Suppressor-Spannung [V]"=w1112, "Zeit/Messschritt [ms]"=w1118, "MCP-Spannung [V]"=w1114, "Zeit/Messung [ms]"=w1119, "Phosphorschirm-Spannung [V]"=w1115, "xyz [mm]"=w1106) -> ("Messung Nr."=w1116:i32)  [unwired: 4 in, 1 out]
                      }
                      frame #1 {
                        n625 = local read "Day folder"() -> (w1150:string)
                        n626 = local read "Fehler (Ausgang)"() -> (w1145:errorcluster)
                        n627 = local read "Einzelbilder speichern"() -> (w1152:bool)
                        n628 = local read "# x-U-Scan Spannungsschritte"() -> (w1141:i32)
                        n629 = local read "# x-U-Scan x-Rasterschritte"() -> (w1140:i32)
                        n630 = call "create_save_folder.vi"("Day folder"=w1150, "Measuring number"=w1142, "Measuring folder"="x-U-Scan" ("Subfolder"), "error in"=w1145) -> ("Save Folder"=w1149:string, "Error Out"=w1148:errorcluster)  [unwired: 5 in]
                        n631 = local write "Save folder"(w1149) -> ()
                        n632 = Multiply(x=w1141, y=w1140) -> (x*y=w1143:i32)
                        n633 = local read "Gemittelte Bilder speichern"() -> (w1153:bool)
                        n634 = local read "Kamera"() -> (w1154:bool)
                        n635 = case shown="True" w1152 {
                          tunnel: w1148 -> [w1155 w1157]
                          tunnel: [w1155 w1156] -> w1147
                          frame #0 {
                          }
                          frame #1 {
                            n636 = local read "Save folder"() -> (w1160:string)
                            n637 = Concatenate Strings(w1160, "\\Einzelbilder" ("Subfolder")) -> (w1158:string)
                            n638 = String To Path(string=w1158) -> (path=w1161:path)
                            n639 = call <vilib>:"Check if File or Folder Exists.vi"("error in (no error)"=w1157, "path"=w1161) -> ("error out"=w1156:errorcluster, "file or folder exists?"=w1162:bool, "dup path"=w1163:path)  [unwired: 7 in]
                            n640 = case shown="False" w1162 {
                              tunnel: w1163 -> [w1164 _]
                              frame #0 {
                                n641 = Create Folder(path (use dialog)=w1164) -> ()  [unwired: 2 in, 3 out]
                              }
                              frame #1 {
                              }
                            }
                          }
                        }
                        n642 = local write "# Messschritte"(w1143) -> ()
                        n643 = case shown="True" w1153 {
                          tunnel: w1147 -> [w1165 w1167]
                          tunnel: [w1165 w1166] -> w1146
                          frame #0 {
                          }
                          frame #1 {
                            n644 = local read "Save folder"() -> (w1171:string)
                            n645 = Concatenate Strings(w1171, "\\Gemittelte Bilder" ("Subfolder")) -> (w1173:string)
                            n646 = String To Path(string=w1173) -> (path=w1170:path)
                            n647 = call <vilib>:"Check if File or Folder Exists.vi"("error in (no error)"=w1167, "path"=w1170) -> ("error out"=w1166:errorcluster, "file or folder exists?"=w1169:bool, "dup path"=w1168:path)  [unwired: 7 in]
                            n648 = case shown="False" w1169 {
                              tunnel: w1168 -> [w1174 _]
                              frame #0 {
                                n649 = Create Folder(path (use dialog)=w1174) -> ()  [unwired: 2 in, 3 out]
                              }
                              frame #1 {
                              }
                            }
                          }
                        }
                        n650 = case shown="True" w1154 {
                          tunnel: [w1175 w1177] -> w1144
                          tunnel: w1146 -> [w1175 w1176]
                          frame #0 {
                          }
                          frame #1 {
                            n651 = local read "Ereignis: FrameDone?"() -> (w1178:refnum<event-registration>)
                            n652 = local read "Detektionskamera"() -> (w1179:T4)
                            n653 = call "camera_release_configuration.vi"("error in"=w1176, "Session In"=w1179, "Ereignisregistrierung (Referenz) 2"=w1178) -> ("error out"=w1177:errorcluster)  [unwired: 1 out]
                          }
                        }
                        n654 = local write "Fehler (Ausgang)"(w1144) -> ()
                      }
                    }
                  }
                  frame #2 {
                    n655 = flat-sequence {
                      frame #0 {
                        n656 = local read "x-U-Scan x-Rasterschritt [µm]"() -> (w1181:dbl)
                        n657 = local read "x-U-Scan Spannungsstart [V]"() -> (w1186:dbl)
                        n658 = local read "x-U-Scan x-Startposition [mm]"() -> (w1185:dbl)
                        n659 = local read "x-U-Scan Spannungsschritt [V]"() -> (w1184:dbl)
                        n660 = local read "# x-U-Scan Spannungsschritte"() -> (w1188:i32)
                        n661 = local read "# x-U-Scan x-Rasterschritte"() -> (w1187:i32)
                        n662 = control-ref of="2D-Intensitätsverteilung (MCP)"() -> (w1183:refnum<vi>)
                        n663 = Divide(x=w1181, y=1000.0) -> (x/y=w1182:dbl)
                        n664 = Initialize Array(0.0 ("y"), w1187, w1188) -> (w1192:dbl[][])
                        n665 = local write "2D-Intensitätsverteilung (MCP)"(w1192) -> ()
                        n666 = property class="IntGraph (strikt)"(reference=w1183, "XScale.Offset"=w1185, "XScale.Multiplier"=w1182, "YScale.Offset"=w1186, "YScale.Multiplier"=w1184, "XScale.MinorInc"=w1182, "YScale.MinorInc"=w1184, "XScale.NameLbl.Text"="Position [mm]" ("Y-Achse.Namensbeschriftung.Text"), "YScale.NameLbl.Text"="Spannung [V]" ("X-Achse.Namensbeschriftung.Text")) -> (error out=w1191:errorcluster)  [unwired: 1 in, 1 out]
                        n667 = local write "Fehler (Ausgang)"(w1191) -> ()
                      }
                      frame #1 {
                        n668 = local write "x-U-Scan läuft"(TRUE ("Messung läuft")) -> ()
                      }
                    }
                  }
                }
              }
            }
          }
          event #6 {
            n669 = event-data() -> ("NewVal"=w1195:bool)  [unwired: 1 in]
            n670 = case shown="True" w1195 {
              frame #0 {
              }
              frame #1 {
                n671 = flat-sequence {
                  tunnel: [w1200] -> w1196
                  tunnel: w1196 -> [w1217]
                  frame #0 {
                    n672 = local read "Raum-Koordinate 2 (Lagenausgleich)"() -> (w1198:enum16{"x-Achse", "y-Achse", "z-Achse"})
                    n673 = local write "Ausgleichslage Start festlegen"(FALSE ("Ausgleichslage Ende festlegen")) -> ()
                    n674 = local read "x-U-Scan (Ausgleichslage) xy-Start [mm]"() -> (w1201:dbl[])
                    n675 = local read "Raum-Koordinate 1"() -> (w1199:enum16{"x-Achse", "y-Achse", "z-Achse"})
                    n676 = call "stage_get_current_xyz.vi"() -> ("Aktuelle xyz-Position OUT [mm]"=w1206:dbl[])  [unwired: 3 in, 1 out]
                    n677 = Index Array(array=w1206, index #1=w1199, index #2=w1198) -> (element #1=w1203:dbl, element #2=w1202:dbl)
                    n678 = Replace Array Subset(array=w1201, new element #1=w1203, index #1=0 ("Index"), new element #2=w1202, index #2=1 ("Index")) -> (w1200:dbl[])
                    n679 = local write "x-U-Scan (Ausgleichslage) xy-Start [mm]"(w1200) -> ()
                  }
                  frame #1 {
                    n680 = local read "x-U-Scan (Ausgleichslage) xy-End [mm]"() -> (w1218:dbl[])
                    n681 = Index Array(array=w1217, index #1=0 ("Index"), index #2=1 ("Index")) -> (element #1=w1209:dbl, element #2=w1212:dbl)
                    n682 = Index Array(array=w1218, index #1=0 ("Index"), index #2=1 ("Index")) -> (element #1=w1208:dbl, element #2=w1211:dbl)
                    n683 = Not Equal?(x=w1209, y=w1208) -> (x != y?=w1207:bool)
                    n684 = case shown="True" w1207 {
                      tunnel: w1212 -> [_ w1224]
                      tunnel: w1211 -> [_ w1223]
                      tunnel: w1208 -> [_ w1222]
                      tunnel: w1209 -> [_ w1221]
                      tunnel: [0.0 w1220] -> w1210
                      frame #0 {
                      }
                      frame #1 {
                        n685 = Subtract(x=w1221, y=w1222) -> (x-y=w1225:dbl)
                        n686 = Subtract(x=w1224, y=w1223) -> (x-y=w1226:dbl)
                        n687 = Divide(x=w1226, y=w1225) -> (x/y=w1220:dbl)
                      }
                    }
                    n688 = local write "x-U-Scan (Ausgleichslage) Steigung"(w1210) -> ()
                  }
                }
              }
            }
          }
          event #7 {
            n689 = event-data() -> ("NewVal"=w1227:bool)  [unwired: 1 in]
            n690 = case shown="True" w1227 {
              frame #0 {
              }
              frame #1 {
                n691 = flat-sequence {
                  tunnel: [w1232] -> w1228
                  tunnel: w1228 -> [w1249]
                  frame #0 {
                    n692 = local read "Raum-Koordinate 2 (Lagenausgleich)"() -> (w1230:enum16{"x-Achse", "y-Achse", "z-Achse"})
                    n693 = local write "Ausgleichslage Ende festlegen"(FALSE ("Ausgleichslage Ende festlegen")) -> ()
                    n694 = local read "x-U-Scan (Ausgleichslage) xy-End [mm]"() -> (w1233:dbl[])
                    n695 = local read "Raum-Koordinate 1"() -> (w1231:enum16{"x-Achse", "y-Achse", "z-Achse"})
                    n696 = call "stage_get_current_xyz.vi"() -> ("Aktuelle xyz-Position OUT [mm]"=w1238:dbl[])  [unwired: 3 in, 1 out]
                    n697 = Index Array(array=w1238, index #1=w1231, index #2=w1230) -> (element #1=w1235:dbl, element #2=w1234:dbl)
                    n698 = Replace Array Subset(array=w1233, new element #1=w1235, index #1=0 ("Index"), new element #2=w1234, index #2=1 ("Index")) -> (w1232:dbl[])
                    n699 = local write "x-U-Scan (Ausgleichslage) xy-End [mm]"(w1232) -> ()
                  }
                  frame #1 {
                    n700 = local read "x-U-Scan (Ausgleichslage) xy-Start [mm]"() -> (w1250:dbl[])
                    n701 = Index Array(array=w1249, index #1=0 ("Index"), index #2=1 ("Index")) -> (element #1=w1241:dbl, element #2=w1244:dbl)
                    n702 = Index Array(array=w1250, index #1=0 ("Index"), index #2=1 ("Index")) -> (element #1=w1240:dbl, element #2=w1243:dbl)
                    n703 = Not Equal?(x=w1241, y=w1240) -> (x != y?=w1239:bool)
                    n704 = case shown="True" w1239 {
                      tunnel: w1244 -> [_ w1256]
                      tunnel: w1243 -> [_ w1255]
                      tunnel: w1240 -> [_ w1254]
                      tunnel: w1241 -> [_ w1253]
                      tunnel: [0.0 w1252] -> w1242
                      frame #0 {
                      }
                      frame #1 {
                        n705 = Subtract(x=w1253, y=w1254) -> (x-y=w1257:dbl)
                        n706 = Subtract(x=w1256, y=w1255) -> (x-y=w1258:dbl)
                        n707 = Divide(x=w1258, y=w1257) -> (x/y=w1252:dbl)
                      }
                    }
                    n708 = local write "x-U-Scan (Ausgleichslage) Steigung"(w1242) -> ()
                  }
                }
              }
            }
          }
          event #8 {
            n709 = event-data() -> ("NewVal"=w1259:bool)  [unwired: 1 in]
            n710 = case shown="True" w1259 {
              frame #0 {
              }
              frame #1 {
                n711 = control-ref of="Shutter time (ms)"() -> (w1295:refnum<vi>)
                n712 = property class="Ring (strikt)"(reference=w1295) -> ("RingText.Text"=w1277:string)  [unwired: 1 in, 2 out]
                n713 = local read "# Bilder/Messschritt"() -> (w1273:i32)
                n714 = local read "Suppressor-Spannung [V]"() -> (w1260:dbl)
                n715 = local read "P-Schirm-Spannung [V]"() -> (w1265:dbl)
                n716 = local read "MCP-Spannung [V]"() -> (w1264:dbl)
                n717 = local read "Leistung (iK) [mW]"() -> (w1263:dbl)
                n718 = local read "Tip-Spannung [V]"() -> (w1261:dbl)
                n719 = local read "Polarisation [°]"() -> (w1268:dbl)
                n720 = local read "Messlogbuch"() -> (w1270:path)
                n721 = Decimal String To Number(string=w1277) -> (number=w1272:i32)  [unwired: 2 in, 1 out]
                n722 = local read "Proben-ID"() -> (w1269:string)
                n723 = Multiply(x=w1273, y=w1272) -> (x*y=w1271:i32)
                n724 = Concatenate Strings(w1277, "ms_" ("String")) -> (w1276:string)
                n725 = local read "Sequenz Ordner"() -> (w1293:string)
                n726 = local read "ROI"() -> (w1266:i32[])
                n727 = local read "Day folder"() -> (w1294:string)
                n728 = call "stage_get_current_xyz.vi"() -> ("Aktuelle xyz-Position OUT [mm]"=w1274:dbl[])  [unwired: 3 in, 1 out]
                n729 = call "create_measure_log_entry.vi"("Messlogbuch-Pfad"=w1270, "Probe"=w1269, "Polarisation [°]"=w1268, "Messart"="Referenzbilder", "ROI"=w1266, "Messungen/Messschritt"=w1273, "Maximalleistung (iK) [mW]"=w1263, "Tip-Spannung [V]"=w1261, "Suppressor-Spannung [V]"=w1260, "Zeit/Messschritt [ms]"=w1272, "MCP-Spannung [V]"=w1264, "Zeit/Messung [ms]"=w1271, "Phosphorschirm-Spannung [V]"=w1265, "xyz [mm]"=w1274) -> ("Messung Nr."=w1262:i32)  [unwired: 4 in, 1 out]
                n730 = call "create_save_folder.vi"("Day folder"=w1294, "Measuring number"=w1262, "Measuring folder"=w1293) -> ("Save Folder"=w1280:string, "Error Out"=w1291:errorcluster)  [unwired: 6 in]
                n731 = local write "Save folder"(w1280) -> ()
                n732 = local read "Kamera"() -> (w1292:bool)
                n733 = case shown="True" w1292 {
                  tunnel: [w1297 w1300] -> w1283
                  tunnel: w1291 -> [w1297 w1299]
                  tunnel: [w1296 w1298] -> w1282
                  frame #0 {
                    n734 = local read "Detektionskamera"() -> (w1296:T4)
                  }
                  frame #1 {
                    n735 = local read "Ereignis: FrameDone?"() -> (w1301:refnum<event-registration>)
                    n736 = local read "Detektionskamera"() -> (w1302:T4)
                    n737 = call "camera_release_configuration.vi"("error in"=w1299, "Session In"=w1302, "Ereignisregistrierung (Referenz) 2"=w1301) -> ("error out"=w1300:errorcluster, "Session Out"=w1298:T4)
                  }
                }
                n738 = local read "# Bilder/Messschritt"() -> (w1289:i32)
                n739 = call "camera_acquisition_sequence.vi"("Session In"=w1282, "Desired image number"=w1289, "error in"=w1283) -> ("Session Out"=w1281:T4, "Image Array"=w1290:T3[], "error out"=w1288:errorcluster)  [unwired: 1 in]
                n740 = local read "Buffer Interval"() -> (w1286:u32)
                n741 = call "save images.vi"("Save Folder"=w1280, "File name prefix"=w1276, "Array"=w1290, "error out 2"=w1288, "Bilder/Messschritt"=w1289) -> ("error out"=w1285:errorcluster)
                n742 = call "camera_create_configuration.vi"("error in"=w1285, "BufferInterval"=w1286, "Session Out 2"=w1281) -> ("Fehler (Ausgang)"=w1279:errorcluster, "Session Out"=w1284:T4, "Ereignisregistrierung (Referenz)"=w1287:refnum<event-registration>)
                n743 = local write "Ereignis: FrameDone?"(w1287) -> ()
                n744 = local write "Detektionskamera"(w1284) -> ()
                n745 = local write "Fehler (Ausgang)"(w1279) -> ()
                n746 = Unbundle By Name(w1279) -> ("status"=w1275:bool)
                n747 = local write "Sequenzaufnahme ON"(w1275) -> ()
              }
            }
          }
        }
        n748 = local read "Fehler (Ausgang)"() -> (w473:errorcluster)
        n749 = local read "Programm beenden"() -> (w471:bool)
        n750 = Unbundle By Name(w473) -> ("status"=w472:bool)
        n751 = Or(x=w472, y=w471) -> (x .or. y?=w468:bool)
        "Scanschleifenzähler" <- w469
      }
      n752 = while "Kamera-Schleife" {
        i -> [w1303]
        stop <- w1304 stop-if-true
        n753 = local read "Fehler (Ausgang)"() -> (w1305:errorcluster)
        n754 = local read "Ereignis: FrameDone?"() -> (w1308:refnum<event-registration>)
        n755 = local read "Programm beenden"() -> (w1307:bool)
        n756 = Unbundle By Name(w1305) -> ("status"=w1306:bool)
        n757 = Or(x=w1306, y=w1307) -> (x .or. y?=w1304:bool)
        n758 = event "Kamera-Ereignisse" shown="[1] \"Kamera ON/OFF\": Wertänderung" {
          selector: w1308 -> [_ _ _ _ _ _]
          dyn-events: _ -> [_ _ _ _ _ _]
          timeout: 1000 -> [_ _ _ _ _ _]
          event #0 {
            n759 = event-data() -> ()  [unwired: 1 in, 2 out]
          }
          event #1 {
            n760 = event-data() -> ()  [unwired: 1 in, 4 out]
            n761 = local read "Detektionskamera"() -> (w1311:T4)
            n762 = local read "Kamera ON/OFF"() -> (w1312:bool)
            n763 = case shown="True" w1312 {
              tunnel: w1311 -> [w1313 w1318]
              tunnel: [w1316 w1319] -> w1310
              frame #0 {
                n764 = local read "Image Memory"() -> (w1314:T3)
                n765 = call "camera_release configuration_stop.vi"("Image Memory"=w1314, "Detektionskamera"=w1313) -> ("error out"=w1316:errorcluster, "status"=w1315:bool)
                n766 = local write "Kamera"(w1315) -> ()
              }
              frame #1 {
                n767 = local read "Buffer Interval"() -> (w1317:u32)
                n768 = call "camera_acquisition_continously.vi"("BufferInterval"=w1317, "Detektionskamera"=w1318) -> ("error out"=w1319:errorcluster, "Ereignis: FrameDone?"=w1320:refnum<event-registration>, "Image Memory"=w1321:T3, "Detektionskamera"=w1322:T4, "Kamera eingeschaltet?"=w1323:bool)
                n769 = local write "Kamera"(w1323) -> ()
                n770 = local write "Detektionskamera"(w1322) -> ()
                n771 = local write "Image Memory"(w1321) -> ()
                n772 = local write "Ereignis: FrameDone?"(w1320) -> ()
              }
            }
            n773 = local write "Fehler (Ausgang)"(w1310) -> ()
          }
          event #2 {
            w1336 = IMAQdx_Buffer_Number_Mode."Buffer Number"  # Buffer Number Mode
            n774 = event-data() -> ("ActualBufferNumber"=w1330:u32)  [unwired: 1 in]
            n775 = local read "Detektionskamera"() -> (w1335:T4)
            n776 = local read "Image Memory"() -> (w1334:T3)
            n777 = call <vilib>:"IMAQdx Get Image.vi"("Buffer Number Mode (Next)"=w1336, "Buffer Number In"=w1330, "Image In"=w1334, "Session In"=w1335) -> ("error out"=w1328:errorcluster, "Buffer Number Out"=w1331:u32, "Image Out"=w1327:T3, "Session Out"=w1332:T4)  [unwired: 1 in, 3 out]
            n778 = Not Equal?(x=w1331, y=w1330) -> (x != y?=w1329:bool)
            n779 = local write "Detektionskamera"(w1332) -> ()
            n780 = local write "Image Display"(w1327) -> ()
            n781 = call "IMAQ ImageToArray"("Image"=w1327) -> ("Image Pixels (U8)"=w1326:u8[][])  [unwired: 3 in, 4 out]
            n782 = local write "Image Memory"(w1327) -> ()
            n783 = local write "Buffer Number"(w1331) -> ()
            n784 = call "CalculateFPS.vi"("buffer number"=w1331) -> ("processed FPS"=w1333:dbl)  [unwired: 2 out]
            n785 = local write "Fehler (Ausgang)"(w1328) -> ()
            n786 = To Unsigned Quad Integer(1:w1326) -> (0:w1325:u64[][])
            n787 = local write "Frame Rate (FPS)"(w1333) -> ()
            n788 = local write "Buffer Overrun"(w1329) -> ()
            n789 = Add Array Elements(numeric array=w1325) -> (sum=w1324:u64)
            n790 = local write "Summierte Helligkeit (a.u.)"(w1324) -> ()
          }
          event #3 {
            n791 = event-data() -> ()  [unwired: 1 in, 2 out]
            n792 = local read "Kamera"() -> (w1337:bool)
            n793 = case shown="True" w1337 {
              frame #0 {
              }
              frame #1 {
                n794 = control-ref of="Shutter time (ms)"() -> (w1344:refnum<vi>)
                n795 = property class="Ring (strikt)"(reference=w1344) -> ("RingText.Text"=w1343:string)  [unwired: 1 in, 2 out]
                n796 = local read "Detektionskamera"() -> (w1342:T4)
                n797 = Decimal String To Number(string=w1343) -> (number=w1339:i32)  [unwired: 2 in, 1 out]
                n798 = property class="IMAQdx"(reference=w1342, "ActiveAttribute"="CameraAttributes::Shutter::Value", "ValueDBL"=w1339) -> (reference out=w1341:T4, error out=w1338:errorcluster)  [unwired: 1 in]
                n799 = local write "Detektionskamera"(w1341) -> ()
                n800 = local write "Fehler (Ausgang)"(w1338) -> ()
              }
            }
          }
          event #4 {
            n801 = event-data() -> ()  [unwired: 1 in, 1 out]
            n802 = local read "Kamera"() -> (w1345:bool)
            n803 = case shown="True" w1345 {
              frame #0 {
              }
              frame #1 {
                n804 = local read "Ereignis: FrameDone?"() -> (w1347:refnum<event-registration>)
                n805 = local read "Detektionskamera"() -> (w1351:T4)
                n806 = local read "Buffer Interval"() -> (w1350:u32)
                n807 = local read "ROI"() -> (w1352:i32[])
                n808 = call "camera_change_ROI.vi"("BufferInterval"=w1350, "Region of Interest"=w1352, "Ereignisregistrierung (Referenz) 2"=w1347, "Session In"=w1351) -> ("Fehler (Ausgang)"=w1346:errorcluster, "Ereignisregistrierung (Referenz)"=w1349:refnum<event-registration>, "Session Out"=w1348:T4)  [unwired: 5 in]
                n809 = local write "Detektionskamera"(w1348) -> ()
                n810 = local write "Ereignis: FrameDone?"(w1349) -> ()
                n811 = local write "Fehler (Ausgang)"(w1346) -> ()
              }
            }
          }
          event #5 {
            n812 = event-data() -> ("NewVal"=w1354:bool)  [unwired: 1 in, 1 out]
            n813 = local read "Kamera"() -> (w1355:bool)
            n814 = And(x=w1355, y=w1354) -> (x .and. y?=w1353:bool)
            n815 = case shown="True" w1353 {
              frame #0 {
              }
              frame #1 {
                n816 = local read "Ereignis: FrameDone?"() -> (w1358:refnum<event-registration>)
                n817 = local read "Detektionskamera"() -> (w1362:T4)
                n818 = local read "Buffer Interval"() -> (w1361:u32)
                n819 = call "camera_change_ROI.vi"("BufferInterval"=w1361, "Region of Interest"=i32[] [640, 480, 0, 0] ("Region of Interest (px)"), "Ereignisregistrierung (Referenz) 2"=w1358, "Session In"=w1362) -> ("Fehler (Ausgang)"=w1356:errorcluster, "Ereignisregistrierung (Referenz)"=w1360:refnum<event-registration>, "Session Out"=w1359:T4)  [unwired: 5 in]
                n820 = local write "Detektionskamera"(w1359) -> ()
                n821 = local write "Ereignis: FrameDone?"(w1360) -> ()
                n822 = local write "Fehler (Ausgang)"(w1356) -> ()
              }
            }
          }
        }
        "Kameraschleifenzähler" <- w1303
      }
      n823 = while "x-U-Scan Schleife" {
        stop <- w63 stop-if-true
        n824 = local read "Fehler (Ausgang)"() -> (w64:errorcluster)
        n825 = local read "x-U-Scan läuft"() -> (w62:bool)
        n826 = local read "Programm beenden"() -> (w66:bool)
        n827 = Unbundle By Name(w64) -> ("status"=w65:bool)
        n828 = case shown="True" w62 {
          frame #0 {
          }
          frame #1 {
            n829 = stacked-sequence {
              frame #0 {
                n830 = local read "# x-U-Scan x-Rasterschritte"() -> (w67:i32)
                n831 = for "Schleife für Raumkoordinate" {
                  N: w67 -> [_]
                  i -> [w68]
                  n832 = local read "x-U-Scan läuft"() -> (w69:bool)
                  n833 = case shown="True" w69 {
                    tunnel: w68 -> [_ w70]
                    frame #0 {
                    }
                    frame #1 {
                      n834 = stacked-sequence {
                        tunnel: w70 -> [w72 _]
                        frame #0 {
                          n835 = local read "# x-U-Scan Spannungsschritte"() -> (w71:i32)
                          n836 = for "Schleife für Spannungskoordinate" {
                            N: w71 -> [_]
                            tunnel: w72 -> [w74]
                            i -> [w73]
                            n837 = local read "x-U-Scan läuft"() -> (w75:bool)
                            n838 = case shown="True" w75 {
                              tunnel: w74 -> [_ w77]
                              tunnel: w73 -> [_ w76]
                              frame #0 {
                              }
                              frame #1 {
                                n839 = stacked-sequence {
                                tunnel: w77 -> [_ _ w119 _]
                                tunnel: w76 -> [_ _ w118 _]
                                frame #0 {
                                n840 = local read "ROI"() -> (w83:i32[])
                                n841 = local write "Summierte Helligkeit (a.u.)"(u64 0 ("Summierte Helligkeit (a.u.)")) -> ()
                                n842 = local read "Aktueller Messschritt"() -> (w80:i32)
                                n843 = Index Array(array=w83, index #1=0 ("Index"), index #2=1 ("Index")) -> (element #1=w87:i32, element #2=w86:i32)
                                n844 = Initialize Array(u64 0 ("Element"), w86, w87) -> (w81:u64[][])
                                n845 = Increment(x=w80) -> (x+1=w79:i32)
                                n846 = local write "Gemitteltes Bild"(w81) -> ()
                                n847 = local write "Aktueller Messschritt"(w79) -> ()
                                }
                                frame #1 {
                                n848 = local read "# Bilder/Messschritt"() -> (w91:i32)
                                n849 = local read "Detektionskamera"() -> (w94:T4)
                                n850 = local read "Einzelbilder speichern"() -> (w89:bool)
                                n851 = call "camera_acquisition_sequence.vi"("Session In"=w94, "Desired image number"=w91) -> ("Image Array"=w88:T3[], "error out"=w93:errorcluster)  [unwired: 2 in, 1 out]
                                n852 = case shown="True" w89 {
                                tunnel: w93 -> [w96 w104]
                                tunnel: [w96 w103] -> w92
                                tunnel: w91 -> [w95 w102]
                                tunnel: [w95 w102] -> w90
                                tunnel: w88 -> [_ w101]
                                frame #0 {
                                }
                                frame #1 {
                                n853 = local read "Aktueller Messschritt"() -> (w107:i32)
                                n854 = local read "Save folder"() -> (w99:string)
                                n855 = Concatenate Strings(w99, "Einzelbilder\\" ("String")) -> (w97:string)
                                n856 = Format Into String(format string="%05.0f" ("Format-String"), initial string="#" ("Eingangs-String"), w107) -> (resulting string=w100:string)  [unwired: 1 in, 1 out]
                                n857 = call "save images.vi"("Save Folder"=w97, "File name prefix"=w100, "Array"=w101, "error out 2"=w104, "Bilder/Messschritt"=w102) -> ("error out"=w103:errorcluster)
                                }
                                }
                                n858 = for {
                                N: w90 -> [_]
                                tunnel: w92 -> [w113]
                                tunnel: w88 -> [w111] mode=indexing
                                n859 = call "IMAQ ImageToArray"("error in (no error)"=w113, "Image"=w111) -> ("error out"=w112:errorcluster, "Image Pixels (U8)"=w110:u8[][])  [unwired: 2 in, 3 out]
                                n860 = local read "Gemitteltes Bild"() -> (w108:u64[][])
                                n861 = To Unsigned Quad Integer(1:w110) -> (0:w115:u64[][])
                                n862 = local read "Summierte Helligkeit (a.u.)"() -> (w116:u64)
                                n863 = local write "Fehler (Ausgang)"(w112) -> ()
                                n864 = Add Array Elements(numeric array=w115) -> (sum=w114:u64)
                                n865 = Add(x=w108, y=w110) -> (x+y=w109:u64[][])
                                n866 = local write "Gemitteltes Bild"(w109) -> ()
                                n867 = Add(x=w114, y=w116) -> (x+y=w117:u64)
                                n868 = local write "Summierte Helligkeit (a.u.)"(w117) -> ()
                                }
                                }
                                frame #2 {
                                n869 = local read "# Bilder/Messschritt"() -> (w125:i32)
                                n870 = local read "Gemitteltes Bild"() -> (w123:u64[][])
                                n871 = local read "2D-Intensitätsverteilung (MCP)"() -> (w122:dbl[][])
                                n872 = local read "Summierte Helligkeit (a.u.)"() -> (w120:u64)
                                n873 = local read "Gemittelte Bilder speichern"() -> (w129:bool)
                                n874 = local read "Image Display"() -> (w127:T3)
                                n875 = Divide(x=w123, y=w125) -> (x/y=w124:dbl[][])
                                n876 = call "IMAQ ArrayToImage"("Image Pixels (U8)"=w124, "Image"=w127) -> ("Image Out"=w126:T3)  [unwired: 8 in, 1 out]
                                n877 = Replace Array Subset(array=w122, new element=w120, index (row)=w119, index (col)=w118) -> (w121:dbl[][])
                                n878 = case shown="True" w129 {
                                tunnel: w126 -> [w130 w141]
                                tunnel: [w130 w132] -> w128
                                frame #0 {
                                }
                                frame #1 {
                                n879 = local read "Aktueller Messschritt"() -> (w136:i32)
                                n880 = local read "Save folder"() -> (w138:string)
                                n881 = Format Into String(format string="%05.0f" ("Format-String"), initial string="#" ("Eingangs-String"), w136) -> (resulting string=w135:string)  [unwired: 1 in, 1 out]
                                n882 = Concatenate Strings(w138, "Gemittelte Bilder\\" ("String"), w135, ".png" ("String")) -> (w134:string)
                                n883 = String To Path(string=w134) -> (path=w133:path)
                                n884 = call-poly "IMAQ Write File 2"("File Path"=w133, "Image"=w141) -> ("Image Out (duplicate)"=w132:T3)  [unwired: 8 in, 1 out]
                                }
                                }
                                n885 = local write "2D-Intensitätsverteilung (MCP)"(w121) -> ()
                                n886 = local write "Image Display"(w128) -> ()
                                }
                                frame #3 {
                                n887 = flat-sequence {
                                frame #0 {
                                n888 = local read "x-U-Scan aktuelle Spannung [V]"() -> (w144:dbl)
                                n889 = local read "x-U-Scan Spannungsschritt [V]"() -> (w145:dbl)
                                n890 = local read "Spannungskanal"() -> (w143:refnum<k21>)
                                n891 = Add(x=w144, y=w145) -> (x+y=w142:dbl)
                                n892 = local write "x-U-Scan aktuelle Spannung [V]"(w142) -> ()
                                n893 = call "HV_power_supply_set_voltage.vi"("Desired output voltage in V (HV power supply)"=w142, "Channel of HV power supply"=w143) -> ("error out"=w146:errorcluster)  [unwired: 8 in]
                                n894 = local write "Fehler (Ausgang)"(w146) -> ()
                                }
                                frame #1 {
                                # "Wartezeit für\nneue Spannung"
                                n895 = Wait (ms)(milliseconds to wait=u32 200 ("Zu wartende ms")) -> ()  [unwired: 1 out]
                                }
                                frame #2 {
                                n896 = local read "Aktueller Messschritt"() -> (w149:i32)
                                n897 = local read "Start time [ms]"() -> (w151:timestamp)
                                n898 = local read "# Messschritte"() -> (w150:i32)
                                n899 = call "estimate_stopp_time.vi"("Aktueller Messschritt"=w149, "# Messschritte"=w150, "Startzeit"=w151) -> ("Stopp Zeit"=w148:string)  [unwired: 8 in]
                                n900 = local write "Geschätzte Messzeit"(w148) -> ()
                                }
                                }
                                }
                                }
                              }
                            }
                          }
                        }
                        frame #1 {
                          n901 = flat-sequence {
                            frame #0 {
                              n902 = local read "x-U-Scan Spannungsstart [V]"() -> (w152:dbl)
                              n903 = local read "Spannungskanal"() -> (w153:refnum<k21>)
                              n904 = local write "x-U-Scan aktuelle Spannung [V]"(w152) -> ()
                              n905 = call "HV_power_supply_set_voltage.vi"("Desired output voltage in V (HV power supply)"=w152, "Channel of HV power supply"=w153) -> ("error out"=w154:errorcluster)  [unwired: 8 in]
                              n906 = local write "Fehler (Ausgang)"(w154) -> ()
                            }
                            frame #1 {
                              # "Fahre nächste x-Position an"
                              n907 = local read "x-U-Scan x-Rasterschritt [µm]"() -> (w159:dbl)
                              n908 = local read "Achs-ID"() -> (w158:i32)
                              n909 = Decrement(x=w158) -> (x-1=w157:i32)
                              n910 = call "stage_move_axis_relative.vi"("Achse"=w158, "Schrittweite [µm]"=w159) -> ("xyz-Position OUT [mm]"=w156:dbl[])  [unwired: 1 in, 2 out]
                              n911 = Index Array(array=w156, index=w157) -> (element=w155:dbl)
                              n912 = local write "x-U-Scan aktuelle x-Position [mm]"(w155) -> ()
                            }
                            frame #2 {
                              n913 = local read "x-U-Scan (Ausgleichslage) Steigung"() -> (w161:dbl)
                              n914 = Not Equal?(x=w161, y=0.0) -> (x != y?=w162:bool)
                              n915 = case shown="True" w162 {
                                frame #0 {
                                }
                                frame #1 {
                                # "Fahre nächste y-Position an"
                                n916 = local read "Raum-Koordinate 2 (Lagenausgleich)"() -> (w163:enum16{"x-Achse", "y-Achse", "z-Achse"})
                                n917 = local read "x-U-Scan (Ausgleichslage) Steigung"() -> (w165:dbl)
                                n918 = local read "x-U-Scan x-Rasterschritt [µm]"() -> (w167:dbl)
                                n919 = Increment(x=w163) -> (x+1=w164:enum16{"x-Achse", "y-Achse", "z-Achse"})
                                n920 = Multiply(x=w167, y=w165) -> (x*y=w166:dbl)
                                n921 = call "stage_move_axis_relative.vi"("Achse"=w164, "Schrittweite [µm]"=w166) -> ("xyz-Position OUT [mm]"=w168:dbl[])  [unwired: 1 in, 2 out]
                                n922 = Index Array(array=w168, index=w163) -> (element=w169:dbl)
                                n923 = local write "x-U-Scan aktuelle y-Position [mm]"(w169) -> ()
                                }
                              }
                            }
                            frame #3 {
                              # "Wartezeit für\nStartspannung"
                              n924 = Wait (ms)(milliseconds to wait=u32 6000 ("Zu wartende ms")) -> ()  [unwired: 1 out]
                            }
                          }
                        }
                      }
                    }
                  }
                }
              }
              frame #1 {
                n925 = local read "x-U-Scan läuft"() -> (w171:bool)
                n926 = case shown="True" w171 {
                  frame #0 {
                    n927 = flat-sequence {
                      frame #0 {
                        # "Zur Ausgangsposition zurückfahren"
                        n928 = local read "x-U-Scan x-Startposition [mm]"() -> (w172:dbl)
                        n929 = local read "Aktuelle xyz-Position [mm]"() -> (w175:dbl[])
                        n930 = local read "x-U-Scan Spannungsstart [V]"() -> (w179:dbl)
                        n931 = local read "Buffer Interval"() -> (w182:u32)
                        n932 = local read "Achs-ID"() -> (w173:i32)
                        n933 = Decrement(x=w173) -> (x-1=w174:i32)
                        n934 = local read "Detektionskamera"() -> (w183:T4)
                        n935 = Replace Array Subset(array=w175, new element=w172, index=w174) -> (w176:dbl[])
                        n936 = local read "Spannungskanal"() -> (w180:refnum<k21>)
                        n937 = local write "x-U-Scan aktuelle Spannung [V]"(w179) -> ()
                        n938 = call "stage_move_axis_absolute.vi"("Ziel xyz IN [mm]"=w176, "Achse"=w173) -> ("error out"=w177:errorcluster)  [unwired: 1 in, 2 out]
                        n939 = call "camera_create_configuration.vi"("error in"=w177, "BufferInterval"=w182, "Session Out 2"=w183) -> ("Fehler (Ausgang)"=w181:errorcluster, "Ereignisregistrierung (Referenz)"=w184:refnum<event-registration>)  [unwired: 1 out]
                        n940 = local write "Ereignis: FrameDone?"(w184) -> ()
                        n941 = call "HV_power_supply_set_voltage.vi"("error in"=w181, "Desired output voltage in V (HV power supply)"=w179, "Channel of HV power supply"=w180) -> ("error out"=w178:errorcluster)  [unwired: 7 in]
                        n942 = local write "Fehler (Ausgang)"(w178) -> ()
                      }
                    }
                  }
                  frame #1 {
                    w186 = FALSE ("Spannungsscan läuft")
                    n943 = local read "Summierte Helligkeit speichern"() -> (w190:bool)
                    n944 = flat-sequence {
                      frame #0 {
                        # "Zur Ausgangsposition zurückfahren"
                        n945 = local read "Start xyz-Position [mm]"() -> (w195:dbl[])
                        n946 = local read "x-U-Scan Spannungsstart [V]"() -> (w200:dbl)
                        n947 = local read "x-U-Scan Spannungsstart [V]"() -> (w198:dbl)
                        n948 = local read "Detektionskamera"() -> (w203:T4)
                        n949 = local read "Achs-ID"() -> (w192:i32)
                        n950 = local read "Buffer Interval"() -> (w202:u32)
                        n951 = local read "Spannungskanal"() -> (w199:refnum<k21>)
                        n952 = Decrement(x=w192) -> (x-1=w193:i32)
                        n953 = call "stage_move_axis_absolute.vi"("Ziel xyz IN [mm]"=w195, "Achse"=w192) -> ("error out"=w196:errorcluster, "Ziel xyz OUT [mm]"=w194:dbl[])  [unwired: 1 in, 1 out]
                        n954 = call "camera_create_configuration.vi"("error in"=w196, "BufferInterval"=w202, "Session Out 2"=w203) -> ("Fehler (Ausgang)"=w197:errorcluster, "Ereignisregistrierung (Referenz)"=w204:refnum<event-registration>)  [unwired: 1 out]
                        n955 = Index Array(array=w194, index=w193) -> (element=w191:dbl)
                        n956 = local write "x-U-Scan aktuelle x-Position [mm]"(w191) -> ()
                        n957 = local write "x-U-Scan aktuelle Spannung [V]"(w198) -> ()
                        n958 = local write "Ereignis: FrameDone?"(w204) -> ()
                        n959 = call "HV_power_supply_set_voltage.vi"("error in"=w197, "Desired output voltage in V (HV power supply)"=w198, "Channel of HV power supply"=w199) -> ("error out"=w201:errorcluster)  [unwired: 7 in]
                        n960 = local write "x-U-Scan aktuelle Spannung [V]"(w200) -> ()
                        n961 = local write "Fehler (Ausgang)"(w201) -> ()
                      }
                      frame #1 {
                        n962 = local read "x-U-Scan (Ausgleichslage) Steigung"() -> (w206:dbl)
                        n963 = Not Equal?(x=w206, y=0.0) -> (x != y?=w205:bool)
                        n964 = case shown="True" w205 {
                          frame #0 {
                          }
                          frame #1 {
                            n965 = local read "Raum-Koordinate 2 (Lagenausgleich)"() -> (w208:enum16{"x-Achse", "y-Achse", "z-Achse"})
                            n966 = local read "Start xyz-Position [mm]"() -> (w210:dbl[])
                            n967 = Increment(x=w208) -> (x+1=w209:enum16{"x-Achse", "y-Achse", "z-Achse"})
                            n968 = call "stage_move_axis_absolute.vi"("Ziel xyz IN [mm]"=w210, "Achse"=w209) -> ("Ziel xyz OUT [mm]"=w211:dbl[])  [unwired: 1 in, 2 out]
                            n969 = Index Array(array=w211, index=w208) -> (element=w212:dbl)
                            n970 = local write "x-U-Scan aktuelle y-Position [mm]"(w212) -> ()
                          }
                        }
                      }
                    }
                    n971 = local read "2D-Intensitätsverteilung (MCP)"() -> (w189:dbl[][])
                    n972 = local write "x-U-Scan läuft"(w186) -> ()
                    n973 = local write "x-U-Scan ON/OFF"(w186) -> ()
                    n974 = case shown="True" w190 {
                      frame #0 {
                      }
                      frame #1 {
                        n975 = local read "x-U-Scan x-Rasterschritt [µm]"() -> (w220:dbl)
                        n976 = local read "# x-U-Scan Spannungsschritte"() -> (w222:i32)
                        n977 = local read "x-U-Scan Spannungsschritt [V]"() -> (w223:dbl)
                        n978 = local read "x-U-Scan Spannungsstart [V]"() -> (w224:dbl)
                        n979 = local read "x-U-Scan (Ausgleichslage) Steigung"() -> (w214:dbl)
                        n980 = local read "x-U-Scan x-Startposition [mm]"() -> (w221:dbl)
                        n981 = local read "# x-U-Scan x-Rasterschritte"() -> (w216:i32)
                        n982 = local read "Save folder"() -> (w218:string)
                        n983 = local read "2D-Intensitätsverteilung (MCP)"() -> (w231:dbl[][])
                        n984 = Divide(x=w220, y=1000.0) -> (x/y=w217:dbl)
                        n985 = call "create_axis_vector_file.vi"("Save folder"=w218, "Dateiname"="yAchse.dat", "Start"=w224, "Schrittlänge"=w223, "# Schritte"=w222) -> ()  [unwired: 11 in]
                        n986 = Concatenate Strings(w218, "\\" ("String"), "2D_Intensitaetsverteilung_MCP.dat" ("String")) -> (w228:string)
                        n987 = Not Equal?(x=w214, y=0.0) -> (x != y?=w215:bool)
                        n988 = call "create_axis_vector_file.vi"("Save folder"=w218, "Dateiname"="xAchse.dat", "Start"=w221, "Schrittlänge"=w217, "# Schritte"=w216) -> ()  [unwired: 11 in]
                        n989 = String To Path(string=w228) -> (path=w229:path)
                        n990 = case shown="True" w215 {
                          tunnel: w218 -> [_ w239]
                          tunnel: w217 -> [_ w236]
                          tunnel: w216 -> [_ w233]
                          frame #0 {
                          }
                          frame #1 {
                            n991 = local read "x-U-Scan (Ausgleichslage) Steigung"() -> (w237:dbl)
                            n992 = local read "x-U-Scan y-Startposition [mm]"() -> (w234:dbl)
                            n993 = Multiply(x=w236, y=w237) -> (x*y=w235:dbl)
                            n994 = call "create_axis_vector_file.vi"("Save folder"=w239, "Dateiname"="zAchse.dat", "Start"=w234, "Schrittlänge"=w235, "# Schritte"=w233) -> ()  [unwired: 11 in]
                          }
                        }
                        n995 = call-poly <vilib>:"Write To Spreadsheet File.vi"("format (%.3f)"="%.;%8.0f", "2D data"=w231, "file path (dialog if empty)"=w229) -> ()  [unwired: 5 in, 1 out]
                      }
                    }
                    n996 = control-ref of="2D-Intensitätsverteilung (MCP)"() -> (w185:refnum<vi>)
                    n997 = Array Max & Min(array=w189) -> (max value=w188:dbl, min value=w187:dbl)  [unwired: 2 out]
                    n998 = property class="IntGraph (strikt)"(reference=w185, "ZScale.Maximum"=w188, "ZScale.Minimum"=w187) -> ()  [unwired: 1 in, 2 out]
                  }
                }
              }
            }
          }
        }
        n999 = Or(x=w65, y=w66) -> (x .or. y?=w63:bool)
      }
      n1000 = while "Spannungsscan-Schleife" {
        stop <- w241 stop-if-true
        n1001 = local read "Fehler (Ausgang)"() -> (w242:errorcluster)
        n1002 = local read "Spannungsscan läuft"() -> (w240:bool)
        n1003 = local read "Programm beenden"() -> (w244:bool)
        n1004 = Unbundle By Name(w242) -> ("status"=w243:bool)
        n1005 = Or(x=w243, y=w244) -> (x .or. y?=w241:bool)
        n1006 = case shown="True" w240 {
          frame #0 {
          }
          frame #1 {
            n1007 = stacked-sequence {
              frame #0 {
                n1008 = local read "# Spannungsschritte"() -> (w249:i32[])
                n1009 = Index Array(array=w249, index #1=0 ("Index"), index #2=1 ("Index")) -> (element #1=w246:i32, element #2=w245:i32)
                n1010 = for "Schleife für Tip-Spannung" {
                  N: w246 -> [_]
                  tunnel: w245 -> [w250]
                  i -> [w251]
                  n1011 = local read "Spannungsscan läuft"() -> (w252:bool)
                  n1012 = case shown="True" w252 {
                    tunnel: w251 -> [_ w254]
                    tunnel: w250 -> [_ w253]
                    frame #0 {
                    }
                    frame #1 {
                      n1013 = stacked-sequence {
                        tunnel: w254 -> [w256 _]
                        tunnel: w253 -> [w255 _]
                        frame #0 {
                          n1014 = for "Schleife für Suppressor-Spannung" {
                            N: w255 -> [_]
                            tunnel: w256 -> [w258]
                            i -> [w257]
                            n1015 = local read "Spannungsscan läuft"() -> (w259:bool)
                            n1016 = case shown="True" w259 {
                              tunnel: w258 -> [_ w261]
                              tunnel: w257 -> [_ w260]
                              frame #0 {
                              }
                              frame #1 {
                                n1017 = stacked-sequence {
                                tunnel: w261 -> [_ _ w303 _]
                                tunnel: w260 -> [_ _ w302 _]
                                frame #0 {
                                n1018 = local read "ROI"() -> (w267:i32[])
                                n1019 = local write "Summierte Helligkeit (a.u.)"(u64 0 ("Summierte Helligkeit (a.u.)")) -> ()
                                n1020 = local read "Aktueller Messschritt"() -> (w264:i32)
                                n1021 = Index Array(array=w267, index #1=0 ("Index"), index #2=1 ("Index")) -> (element #1=w271:i32, element #2=w270:i32)
                                n1022 = Initialize Array(u64 0 ("Element"), w270, w271) -> (w265:u64[][])
                                n1023 = Increment(x=w264) -> (x+1=w263:i32)
                                n1024 = local write "Gemitteltes Bild"(w265) -> ()
                                n1025 = local write "Aktueller Messschritt"(w263) -> ()
                                }
                                frame #1 {
                                n1026 = local read "# Bilder/Messschritt"() -> (w275:i32)
                                n1027 = local read "Detektionskamera"() -> (w278:T4)
                                n1028 = local read "Einzelbilder speichern"() -> (w273:bool)
                                n1029 = call "camera_acquisition_sequence.vi"("Session In"=w278, "Desired image number"=w275) -> ("Image Array"=w272:T3[], "error out"=w277:errorcluster)  [unwired: 2 in, 1 out]
                                n1030 = case shown="True" w273 {
                                tunnel: w277 -> [w280 w288]
                                tunnel: [w280 w287] -> w276
                                tunnel: w275 -> [w279 w286]
                                tunnel: [w279 w286] -> w274
                                tunnel: w272 -> [_ w285]
                                frame #0 {
                                }
                                frame #1 {
                                n1031 = local read "Aktueller Messschritt"() -> (w291:i32)
                                n1032 = local read "Save folder"() -> (w283:string)
                                n1033 = Concatenate Strings(w283, "Einzelbilder\\" ("String")) -> (w281:string)
                                n1034 = Format Into String(format string="%05.0f" ("Format-String"), initial string="#" ("Eingangs-String"), w291) -> (resulting string=w284:string)  [unwired: 1 in, 1 out]
                                n1035 = call "save images.vi"("Save Folder"=w281, "File name prefix"=w284, "Array"=w285, "error out 2"=w288, "Bilder/Messschritt"=w286) -> ("error out"=w287:errorcluster)
                                }
                                }
                                n1036 = for {
                                N: w274 -> [_]
                                tunnel: w276 -> [w297]
                                tunnel: w272 -> [w295] mode=indexing
                                n1037 = call "IMAQ ImageToArray"("error in (no error)"=w297, "Image"=w295) -> ("error out"=w296:errorcluster, "Image Pixels (U8)"=w294:u8[][])  [unwired: 2 in, 3 out]
                                n1038 = local read "Gemitteltes Bild"() -> (w292:u64[][])
                                n1039 = To Unsigned Quad Integer(1:w294) -> (0:w299:u64[][])
                                n1040 = local read "Summierte Helligkeit (a.u.)"() -> (w300:u64)
                                n1041 = local write "Fehler (Ausgang)"(w296) -> ()
                                n1042 = Add Array Elements(numeric array=w299) -> (sum=w298:u64)
                                n1043 = Add(x=w292, y=w294) -> (x+y=w293:u64[][])
                                n1044 = local write "Gemitteltes Bild"(w293) -> ()
                                n1045 = Add(x=w298, y=w300) -> (x+y=w301:u64)
                                n1046 = local write "Summierte Helligkeit (a.u.)"(w301) -> ()
                                }
                                }
                                frame #2 {
                                n1047 = local read "# Bilder/Messschritt"() -> (w309:i32)
                                n1048 = local read "Gemitteltes Bild"() -> (w307:u64[][])
                                n1049 = local read "Gemittelte Bilder speichern"() -> (w313:bool)
                                n1050 = local read "2D-Intensitätsverteilung (MCP)"() -> (w306:dbl[][])
                                n1051 = local read "Image Display"() -> (w311:T3)
                                n1052 = local read "Summierte Helligkeit (a.u.)"() -> (w304:u64)
                                n1053 = Divide(x=w307, y=w309) -> (x/y=w308:dbl[][])
                                n1054 = call "IMAQ ArrayToImage"("Image Pixels (U8)"=w308, "Image"=w311) -> ("Image Out"=w310:T3)  [unwired: 8 in, 1 out]
                                n1055 = case shown="True" w313 {
                                tunnel: w310 -> [w314 w325]
                                tunnel: [w314 w316] -> w312
                                frame #0 {
                                }
                                frame #1 {
                                n1056 = local read "Aktueller Messschritt"() -> (w320:i32)
                                n1057 = local read "Save folder"() -> (w322:string)
                                n1058 = Format Into String(format string="%05.0f" ("Format-String"), initial string="#" ("Eingangs-String"), w320) -> (resulting string=w319:string)  [unwired: 1 in, 1 out]
                                n1059 = Concatenate Strings(w322, "Gemittelte Bilder\\" ("String"), w319, ".png" ("String")) -> (w318:string)
                                n1060 = String To Path(string=w318) -> (path=w317:path)
                                n1061 = call-poly "IMAQ Write File 2"("File Path"=w317, "Image"=w325) -> ("Image Out (duplicate)"=w316:T3)  [unwired: 8 in, 1 out]
                                }
                                }
                                n1062 = Replace Array Subset(array=w306, new element=w304, index (row)=w303, index (col)=w302) -> (w305:dbl[][])
                                n1063 = local write "2D-Intensitätsverteilung (MCP)"(w305) -> ()
                                n1064 = local write "Image Display"(w312) -> ()
                                }
                                frame #3 {
                                n1065 = flat-sequence {
                                frame #0 {
                                n1066 = local read "Aktuelle Spannung [V]"() -> (w328:dbl[])
                                n1067 = local read "Spannungsschritt [V]"() -> (w332:dbl[])
                                n1068 = Index Array(array=w328, index=1 ("Index")) -> (element=w330:dbl)
                                n1069 = Index Array(array=w332, index=1 ("Index")) -> (element=w331:dbl)
                                n1070 = Add(x=w330, y=w331) -> (x+y=w326:dbl)
                                n1071 = call "HV_power_supply_set_voltage.vi"("Desired output voltage in V (HV power supply)"=w326, "Channel of HV power supply"=refnum<k21> "Dev0/Ao0") -> ("error out"=w335:errorcluster)  [unwired: 8 in]
                                n1072 = Replace Array Subset(array=w328, new element=w326, index=1 ("Index")) -> (w327:dbl[])
                                n1073 = local write "Fehler (Ausgang)"(w335) -> ()
                                n1074 = local write "Suppressor-Spannung [V]"(w326) -> ()
                                n1075 = local write "Aktuelle Spannung [V]"(w327) -> ()
                                }
                                frame #1 {
                                # "Wartezeit für\nneue Spannung"
                                n1076 = Wait (ms)(milliseconds to wait=u32 200 ("Zu wartende ms")) -> ()  [unwired: 1 out]
                                }
                                frame #2 {
                                n1077 = local read "Aktueller Messschritt"() -> (w339:i32)
                                n1078 = local read "Start time [ms]"() -> (w341:timestamp)
                                n1079 = local read "# Messschritte"() -> (w340:i32)
                                n1080 = call "estimate_stopp_time.vi"("Aktueller Messschritt"=w339, "# Messschritte"=w340, "Startzeit"=w341) -> ("Stopp Zeit"=w338:string)  [unwired: 8 in]
                                n1081 = local write "Geschätzte Messzeit"(w338) -> ()
                                }
                                }
                                }
                                }
                              }
                            }
                          }
                        }
                        frame #1 {
                          n1082 = flat-sequence {
                            frame #0 {
                              n1083 = local read "Spannungsstart [V]"() -> (w347:dbl[])
                              n1084 = local read "Aktuelle Spannung [V]"() -> (w349:dbl[])
                              n1085 = Index Array(array=w347, index=1 ("Index")) -> (element=w342:dbl)
                              n1086 = call "HV_power_supply_set_voltage.vi"("Desired output voltage in V (HV power supply)"=w342, "Channel of HV power supply"=refnum<k21> "Dev0/Ao0") -> ("error out"=w343:errorcluster)  [unwired: 8 in]
                              n1087 = local write "Suppressor-Spannung [V]"(w342) -> ()
                              n1088 = Replace Array Subset(array=w349, new element=w342, index=1 ("Index")) -> (w345:dbl[])
                              n1089 = local write "Fehler (Ausgang)"(w343) -> ()
                              n1090 = local write "Aktuelle Spannung [V]"(w345) -> ()
                            }
                            frame #1 {
                              n1091 = local read "Aktuelle Spannung [V]"() -> (w352:dbl[])
                              n1092 = local read "Spannungsschritt [V]"() -> (w356:dbl[])
                              n1093 = Index Array(array=w352, index=0 ("Index")) -> (element=w354:dbl)
                              n1094 = Index Array(array=w356, index=0 ("Index")) -> (element=w355:dbl)
                              n1095 = Add(x=w354, y=w355) -> (x+y=w350:dbl)
                              n1096 = call "HV_power_supply_set_voltage.vi"("Desired output voltage in V (HV power supply)"=w350, "Channel of HV power supply"=refnum<k21> "Dev0/Ao1") -> ("error out"=w359:errorcluster)  [unwired: 8 in]
                              n1097 = local write "Tip-Spannung [V]"(w350) -> ()
                              n1098 = local write "Fehler (Ausgang)"(w359) -> ()
                              n1099 = Replace Array Subset(array=w352, new element=w350, index=0 ("Index")) -> (w351:dbl[])
                              n1100 = local write "Aktuelle Spannung [V]"(w351) -> ()
                            }
                            frame #2 {
                              # "Wartezeit für\nStartspannung"
                              n1101 = Wait (ms)(milliseconds to wait=u32 6000 ("Zu wartende ms")) -> ()  [unwired: 1 out]
                            }
                          }
                        }
                      }
                    }
                  }
                }
              }
              frame #1 {
                n1102 = local read "Spannungsscan läuft"() -> (w362:bool)
                n1103 = case shown="True" w362 {
                  frame #0 {
                    n1104 = flat-sequence {
                      frame #0 {
                        # "Zur Ausgangsposition zurückfahren"
                        n1105 = local read "Spannungsstart [V]"() -> (w363:dbl[])
                        n1106 = local read "Spannungsstart [V]"() -> (w368:dbl[])
                        n1107 = local read "Detektionskamera"() -> (w375:T4)
                        n1108 = local read "Buffer Interval"() -> (w374:u32)
                        n1109 = local write "Aktuelle Spannung [V]"(w363) -> ()
                        n1110 = call "camera_create_configuration.vi"("BufferInterval"=w374, "Session Out 2"=w375) -> ("Fehler (Ausgang)"=w369:errorcluster, "Ereignisregistrierung (Referenz)"=w376:refnum<event-registration>)  [unwired: 1 in, 1 out]
                        n1111 = Index Array(array=w368, index #1=0 ("Index"), index #2=1 ("Index")) -> (element #1=w364:dbl, element #2=w365:dbl)
                        n1112 = local write "Tip-Spannung [V]"(w364) -> ()
                        n1113 = local write "Suppressor-Spannung [V]"(w365) -> ()
                        n1114 = local write "Ereignis: FrameDone?"(w376) -> ()
                        n1115 = call "HV_power_supply_set_voltage.vi"("error in"=w369, "Desired output voltage in V (HV power supply)"=w365, "Channel of HV power supply"=refnum<k21> "Dev0/Ao0") -> ("error out"=w371:errorcluster)  [unwired: 7 in]
                        n1116 = call "HV_power_supply_set_voltage.vi"("error in"=w371, "Desired output voltage in V (HV power supply)"=w364, "Channel of HV power supply"=refnum<k21> "Dev0/Ao1") -> ("error out"=w370:errorcluster)  [unwired: 7 in]
                        n1117 = local write "Fehler (Ausgang)"(w370) -> ()
                      }
                    }
                  }
                  frame #1 {
                    w378 = FALSE ("Spannungsscan läuft")
                    n1118 = local read "Summierte Helligkeit speichern"() -> (w382:bool)
                    n1119 = local write "Spannungsscan läuft"(w378) -> ()
                    n1120 = local write "Spannungsscan ON/OFF"(w378) -> ()
                    n1121 = flat-sequence {
                      frame #0 {
                        # "Zur Ausgangsposition zurückfahren"
                        n1122 = local read "Spannungsstart [V]"() -> (w383:dbl[])
                        n1123 = local read "Spannungsstart [V]"() -> (w388:dbl[])
                        n1124 = local read "Detektionskamera"() -> (w395:T4)
                        n1125 = local read "Buffer Interval"() -> (w394:u32)
                        n1126 = local write "Aktuelle Spannung [V]"(w383) -> ()
                        n1127 = call "camera_create_configuration.vi"("BufferInterval"=w394, "Session Out 2"=w395) -> ("Fehler (Ausgang)"=w389:errorcluster, "Ereignisregistrierung (Referenz)"=w396:refnum<event-registration>)  [unwired: 1 in, 1 out]
                        n1128 = Index Array(array=w388, index #1=0 ("Index"), index #2=1 ("Index")) -> (element #1=w384:dbl, element #2=w385:dbl)
                        n1129 = local write "Tip-Spannung [V]"(w384) -> ()
                        n1130 = local write "Suppressor-Spannung [V]"(w385) -> ()
                        n1131 = local write "Ereignis: FrameDone?"(w396) -> ()
                        n1132 = call "HV_power_supply_set_voltage.vi"("error in"=w389, "Desired output voltage in V (HV power supply)"=w385, "Channel of HV power supply"=refnum<k21> "Dev0/Ao0") -> ("error out"=w391:errorcluster)  [unwired: 7 in]
                        n1133 = call "HV_power_supply_set_voltage.vi"("error in"=w391, "Desired output voltage in V (HV power supply)"=w384, "Channel of HV power supply"=refnum<k21> "Dev0/Ao1") -> ("error out"=w390:errorcluster)  [unwired: 7 in]
                        n1134 = local write "Fehler (Ausgang)"(w390) -> ()
                      }
                    }
                    n1135 = case shown="True" w382 {
                      frame #0 {
                      }
                      frame #1 {
                        w397 = 1 ("Index")
                        w409 = 0 ("Index")
                        n1136 = local read "Spannungsschritt [V]"() -> (w407:dbl[])
                        n1137 = local read "# Spannungsschritte"() -> (w408:i32[])
                        n1138 = local read "Spannungsstart [V]"() -> (w406:dbl[])
                        n1139 = local read "Save folder"() -> (w398:string)
                        n1140 = local read "2D-Intensitätsverteilung (MCP)"() -> (w415:dbl[][])
                        n1141 = Index Array(array=w408, index #1=w409, index #2=w397) -> (element #1=w403:i32, element #2=w399:i32)
                        n1142 = Index Array(array=w406, index #1=w409, index #2=w397) -> (element #1=w405:dbl, element #2=w401:dbl)
                        n1143 = Index Array(array=w407, index #1=w409, index #2=w397) -> (element #1=w404:dbl, element #2=w400:dbl)
                        n1144 = call "create_axis_vector_file.vi"("Save folder"=w398, "Dateiname"="yAchse.dat", "Start"=w401, "Schrittlänge"=w400, "# Schritte"=w399) -> ()  [unwired: 11 in]
                        n1145 = call "create_axis_vector_file.vi"("Save folder"=w398, "Dateiname"="xAchse.dat" ("Save folder"), "Start"=w405, "Schrittlänge"=w404, "# Schritte"=w403) -> ()  [unwired: 11 in]
                        n1146 = Concatenate Strings(w398, "\\" ("String"), "2D_Intensitaetsverteilung_MCP.dat" ("String")) -> (w412:string)
                        n1147 = String To Path(string=w412) -> (path=w413:path)
                        n1148 = call-poly <vilib>:"Write To Spreadsheet File.vi"("format (%.3f)"="%.;%8.0f", "2D data"=w415, "file path (dialog if empty)"=w413) -> ()  [unwired: 5 in, 1 out]
                      }
                    }
                    n1149 = local read "2D-Intensitätsverteilung (MCP)"() -> (w381:dbl[][])
                    n1150 = control-ref of="2D-Intensitätsverteilung (MCP)"() -> (w377:refnum<vi>)
                    n1151 = Array Max & Min(array=w381) -> (max value=w380:dbl, min value=w379:dbl)  [unwired: 2 out]
                    n1152 = property class="IntGraph (strikt)"(reference=w377, "ZScale.Maximum"=w380, "ZScale.Minimum"=w379) -> ()  [unwired: 1 in, 2 out]
                  }
                }
              }
            }
          }
        }
      }
    }
    frame #2 {
      n1153 = flat-sequence {
        frame #0 {
          n1154 = local read "Kamera"() -> (w1363:bool)
          n1155 = case shown="True" w1363 {
            frame #0 {
            }
            frame #1 {
              n1156 = local read "Detektionskamera"() -> (w1365:T4)
              n1157 = local read "Image Memory"() -> (w1367:T3)
              n1158 = call "camera_release configuration_stop.vi"("Image Memory"=w1367, "Detektionskamera"=w1365) -> ("error out"=w1364:errorcluster, "status"=w1366:bool)
              n1159 = local write "Kamera"(w1366) -> ()
              n1160 = local write "Fehler (Ausgang)"(w1364) -> ()
            }
          }
        }
        frame #1 {
          # "Wegen Abstürzen des Programms wird dieser Teil verhindert\nAchtung: IMMER manuell Netzteile auf 0V setzen oder HV-\nSteuerung von Hand ausmachen"
          n1161 = local read "HV-Steuerung"() -> (w1370:bool)
          n1162 = And(x=w1370, y=FALSE) -> (x .and. y?=w1368:bool)
          n1163 = case shown="True" w1368 {
            frame #0 {
            }
            frame #1 {
              n1164 = call "HV_power_supply_set_voltage.vi"("Desired output voltage in V (HV power supply)"=0.0, "Channel of HV power supply"=refnum<k21> "Dev0/Ao1") -> ("error out"=w1371:errorcluster)  [unwired: 8 in]
              n1165 = call "HV_power_supply_set_voltage.vi"("Desired output voltage in V (HV power supply)"=0.0, "Channel of HV power supply"=refnum<k21> "Dev0/Ao0") -> ("error out"=w1372:errorcluster)  [unwired: 8 in]
              n1166 = local write "Fehler (Ausgang)"(w1371) -> ()
              n1167 = local write "Fehler (Ausgang)"(w1372) -> ()
            }
          }
        }
        frame #2 {
          n1168 = local read "Wellenplatte"() -> (w1377:bool)
          n1169 = case shown="True" w1377 {
            frame #0 {
            }
            frame #1 {
              n1170 = local read "Wellenplatte [°]"() -> (w1378:refnum<k7>)
              n1171 = invoke class="MG17Motor" method="StopCtrl"(reference=w1378) -> ()  [unwired: 2 in, 3 out]
            }
          }
        }
        frame #3 {
          w1379 = FALSE ("Bühne bereit")
          w1380 = 0.0 ("Suppressor-Spannung [V]")
          n1172 = local write "Bühne"(w1379) -> ()
          n1173 = local write "Tip-Spannung [V]"(w1380) -> ()
          n1174 = local write "Suppressor-Spannung [V]"(w1380) -> ()
          n1175 = local write "Wellenplatte"(w1379) -> ()
          n1176 = local write "Spannungsscan läuft"(w1379) -> ()
          n1177 = local write "HV-Steuerung"(w1379) -> ()
          n1178 = local write "x-U-Scan läuft"(w1379) -> ()
          n1179 = local write "Waveplate ON/OFF"(w1379) -> ()
          n1180 = local write "x-U-Scan ON/OFF"(w1379) -> ()
          n1181 = local write "Kamera ON/OFF"(w1379) -> ()
        }
      }
    }
  }
